vi "ControlProgram6.6_5.vi"() -> ()   [LabVIEW 2016]
uses:
  <vilib>/Utility/miscctls.llb/LVPoint32TypeDef.ctl
  <vilib>/Platform/TimedLoop/XDataNode/timing_clust.ctl
  <vilib>/Platform/TimedLoop/XDataNode/nitl_modes.ctl
  <vilib>/Platform/TimedLoop/XDataNode/wakeup.ctl
  <vilib>/Instr/_visa.llb/Select Event Type.ctl
  <vilib>/vision/Avi1.llb/AviRefnum.ctl
  <vilib>/Utility/error.llb/DialogType.ctl
  <vilib>/DAQmx/write.llb/DAQmx Write (Analog 1D DBL NChan 1Samp).vi
  <vilib>/DAQmx/read.llb/DAQmx Read (Analog 2D DBL NChan NSamp).vi
  <vilib>/Analysis/baseanly.llb/Mean (DBL).vi
  <vilib>/DAQmx/write.llb/DAQmx Write (Digital Bool 1Line 1Point).vi
  <vilib>/DAQmx/create/channels.llb/DAQmx Create Channel (DO-Digital Output).vi
  <vilib>/DAQmx/create/channels.llb/DAQmx Create Channel (AI-Voltage-Basic).vi
  <vilib>/DAQmx/create/channels.llb/DAQmx Create Channel (AO-Voltage-Basic).vi
  <vilib>/DAQmx/configure/timing.llb/DAQmx Timing (Sample Clock).vi
  <vilib>/DAQmx/miscellaneous.llb/DAQmx Fill In Error Info.vi
  <vilib>/Instr/_visa.llb/VISA Configure Serial Port (Instr).vi
  Arnulf--joystick/git(most_up_to_date)/Logitech-joystick/Old Trap/FAST_Global_var.vi
  <vilib>/Utility/inputDevices.llb/mouseAcquire.vi
  <vilib>/Utility/inputDevices.llb/closeMouse.vi
  <vilib>/platform/TimedLoop/XDataNode/XDataNode.xnode
  <vilib>/Platform/TimedLoop/XDataNode/XDNodeRunTimeDep.lvlib
  <resource>/objmgr/daqmx.rc
  <vilib>/Analysis/NI_AALBase.lvlib
panel:
  in  "Save file index":i32
  out "Saving Move":bool
  out "Move time":string
  out "Primary Video Display":T1(plugin-control)
  out "Flush Sample Start Time":u32=2111292881
  out "Sample flush time (s)":dbl=48.0
  in  "Inject Sample":bool
  out "Cal values":T2={"AX alpha"=612.9626061060078, "BX alpha"=549.6584469744151, "AX kappa"=0.3485731373010688, "BX kappa"=0.3853424216291352, "AX offset"=-0.03900484438240665, "BX offset"=-0.11295550662085417, "AY alpha"=582.7562541114835, "BY alpha"=571.1587543790358, "AY kappa"=0.37498408087930674, "BY kappa"=0.36252029651198364, "AY offset"=-0.21125584642206058, "BY offset"=-0.12469077200400738}
  in  "Inject Pump 1":bool
  in  "Inject Pump 2":bool
  in  "Tab Control 2":T3(tab)
  in  "Force FB script":bool
  in  "Got ADig bead":bool
  in  "Move Cap. 2 (ADig Top)":bool
  in  "Dump beads":bool
  in  "Got DNA bead":bool
  in  "Flow on\ncap 2?":bool=TRUE
  in  "Flow on\ncap 1?":bool=TRUE
  in  "Flow on\ndump?":bool=TRUE
  in  "Raster set":i32=1
  in  "Fish After TA?":bool=TRUE
  in  "Delta after tether":dbl=1700.0
  in  "TA Cancel Save?":bool=TRUE
  in  "Min fish\ndelta (nm)":dbl=1425.0 min=0.0 max=5000.0 step=50.0
  in  "Max fish\ndelta (nm)":dbl=1900.0 min=0.0 max=5000.0 step=25.0
  in  "Fish Speed (ms)":i32=5000
  in  "Wait (ms)":i32=1500
  in  "# attempts":dbl=10.0
  in  "Cutoff force (pN)":dbl=4.5
  in  "Raster after\n tether?":bool=TRUE
  out "Tether":bool
  out "Attempt #":i32
  in  "Flow on\nwhile fish?":bool=TRUE
  in  "Flow on\nafter raster?":bool=TRUE
  in  "Offset raster set":i32
  in  "Offset @ Delta (nm)":dbl=1700.0
  in  "Cal @ Delta (nm)":dbl=2500.0
  in  "Cal stage position":i32=3
  out "Cal Final Sampling Rate":dbl=125000.0
  in  "Cal Averaging":i32=1
  in  "Wait before dip (s)":dbl=3.0
  in  "Start dipping after?":bool
  in  "Start trap delta (nm)":dbl=1700.0
  in  "Repeat Dip":bool
  out "Dip #":i32
  in  "Dip attempts":dbl=3.0
  in  "Cancel Rep\n Dip":bool
  out "Return elasped time":i32
  in  "Return duration":dbl=15.0
  in  "Cancel dwell":bool=TRUE
  in  "Pause dwell":bool
  in  "Start/Return position":dbl=3.0
  in  "Dip duration":dbl=15.0
  in  "Dip position":dbl=4.0
  in  "Dip":bool
  out "Dip elasped time":i32
  in  "Stop":bool=TRUE
  in  "?":T4(tab)
  out "FAST X-Y":bool
  out "FAST Z":bool
  in  "Cal time (s)":dbl=5.0
  in  "Save N sets":bool
  in  "N sets":i32=200
  out "Cal sets to save":i32=500
  in  "Reset data stream":bool
  out "Buffer Overflow":bool
  out "Stage moving":bool
  in  "Comment":string
  in  "Raster scan":bool
  out "Saving":bool
  in  "Save cal":bool
  in  "Save Data":bool
  in  "Stop saving":bool
  out "Calibrating":bool
  out "Progress":dbl(slide) scale=0.0..100.0
  in  "Read Cal":bool
  in  "Fish":bool
  in  "Averaging Number":i32=1250
  out "Final Sampling Rate":dbl=100.0
  in  "Trap position (V)":cluster{"X":dbl, "Y":dbl}={"X"=3.9042624789680316, "Y"=0.2}
  in  "Trap delta (nm)":dbl=2500.0 min=0.0 max=5000.0 step=50.0
  in  "Fixed X":dbl=1.1
  in  "Fixed Y":dbl=0.15
  in  "Shutter 1 (B)":bool
  in  "Shutter 2 (A)":bool
  in  "Pulling direction":bool
  out "Raster scanning...":bool
  out "Current file name":path=path "D:/data/160111/160111_006.dat"
  in  "AX alpha":dbl=612.9626061060078 format="%#_3p"
  in  "BX alpha":dbl=549.6584469744151 format="%#_3g"
  in  "AX kappa":dbl=0.3485731373010688 format="%#_3g"
  in  "BX kappa":dbl=0.3853424216291352 format="%#_3g"
  in  "AX offset":dbl=-0.03900484438240665 format="%#_3g"
  in  "BX offset":dbl=-0.11295550662085417 format="%#_3g"
  in  "AY alpha":dbl=582.7562541114835 format="%#_3g"
  in  "BY alpha":dbl=571.1587543790358 format="%#_3g"
  in  "AY kappa":dbl=0.37498408087930674 format="%#_3g"
  in  "BY kappa":dbl=0.36252029651198364 format="%#_3g"
  in  "AY offset":dbl=-0.21125584642206058 format="%#_3g"
  in  "BY offset":dbl=-0.12469077200400738 format="%#_3g"
  out "Buffer status":u8(slide) scale=0.0..100.0
  in  "Target":bool
  in  "Set Current\nPos to (0,0,0)":bool
  in  "dump spot":string="Dump beads spot"
  in  "up flow spot":string="Upper flow spot"
  in  "low flow spot":string="Lower flow spot"
  in  "up cap":string="Upper capillary (ADig beads)"
  in  "bottom cap":string="Lower capillary (DNA beads)"
  in  "Move to Position 5":bool
  in  "Set Position 5":bool
  in  "Saved stage positions":dbl[][](array[numeric])=[[1.0, 0.0, 0.0, 0.0], [2.0, -0.13716, -3.21132, 0.01436], [3.0, 0.45, -0.73974, 0.005], [4.0, 0.45, -2.1978, 0.005], [5.0, 0.45, -2.63158, -0.02256]]
  in  "Set Position 2":bool
  in  "Move to Position 2":bool
  in  "Set Position 1":bool
  in  "Move to Position 1":bool
  in  "Set Position 4":bool
  in  "Move to Position 4":bool
  in  "Set Position 3":bool
  in  "Move to Position 3":bool
  out "Stage error":errorcluster
  in  "Clear Volume":bool
  out "Sample Flush Meter":u8(slide) scale=0.0..100.0
  out "Flushing Sample":bool
  in  "Flush Sample":bool
  in  "Normal \nRate (ul/hr)  3":dbl=100.0
  in  "Normal \nVolume (ul) 3":dbl=250.0
  in  "Normal \nVolume (ul) 2":dbl
  in  "Normal \nRate (ul/hr)":dbl
  in  "Normal \nVolume (ul)":dbl
  in  "Flush\nRate (ul/min)":dbl
  in  "Flush\nVolume (ul)":dbl
  in  "Flush \nRate (ul/min)  2":dbl
  in  "Flush Pump 2":bool
  in  "Flush\nVolume (ul)  2":dbl
  in  "Flush Pump 1":bool
  in  "Normal \nRate (ul/hr)  2":dbl
  in  "Write Wait":i32=1000
  in  "Flush \nRate (ul/min)  3":dbl=100.0
  in  "Flush\nVolume (ul)  3":dbl=80.0
  out "error out":errorcluster
  in  "Use Mouse to Move Trap?":bool
  in  "Pause Mouse/Mirror Connection":bool
  out "Reference Voltage":cluster{dbl, dbl}={0.0, -0.0}
  out "Saved voltage":cluster{dbl, dbl}={5.766666666666665, 1.45}
  out "Real Coordinates":cluster{"Horizontal":i32, "Vertical":i32}={"Horizontal"=897, "Vertical"=-1271}
  out "CoordinatesMousePressed":T5
  in  "Force Feedback 2":bool
  in  "Offset 2":cluster{"Off Y":dbl, "Off X":dbl}={"Off Y"=1.5, "Off X"=0.17}
  in  "Setpoint voltage 2":cluster{"SP Y":dbl, "SP X":dbl}={"SP Y"=0.6, "SP X"=0.0}
  out "Sum error":dbl(knob) scale=-0.2..0.2
  out "Trap sep":waveform(dbl)[](graph)=[{"t0"=timestamp(4.489999999999949 s since 1904-01-01), "dt"=0.002, "Y"=[-1157.7639781743756, -1157.678951177374, -1157.7582331070425, -1157.7490409992681, -1157.8995617642552], "attributes"=variant("NI_ChannelName"=variant(string "T2 X"))}, {"t0"=timestamp(4.489999999999949 s since 1904-01-01), "dt"=0.002, "Y"=[-909.0775466981794, -909.1316439023619, -909.1322956759037, -909.1570630705896, -909.1264297140281], "attributes"=variant("NI_ChannelName"=variant(string "T2 Y"))}]
  in  "Set reading to\nsetpoint 1":bool
  in  "Offset Y (nm)":dbl format="%0.2f"
  in  "Offset X (nm)":dbl format="%0.2f"
  in  "Remove offsets":bool
  in  "Force Feedback 1":bool
  out "Feedback Output \nVoltage 2":cluster{dbl, dbl} {"?" format="%#_4g"; "?" format="%#_4g"}
  in  "Offset 1":cluster{"Off Y":dbl, "Off X":dbl}={"Off Y"=1.5, "Off X"=0.17}
  in  "Setpoint voltage 1":cluster{"SP Y":dbl, "SP X":dbl}={"SP Y"=0.6, "SP X"=0.0}
  in  "Feedback const":T6={"Ki_B_Y"=0.5, "Ki_B_X"=0.0, "Kp Y"=1.0, "Kp X"=0.0}
  out "Mean Trap Pos X 2 (nm)":dbl=-1157.769953044463 format="%0.2f"
  out "Mean Trp Pos Y 2 (nm)":dbl=-909.1249958122125 format="%0.2f"
  out "T2 X RMS (A)":dbl=0.7168002469275427 format="%0.2f"
  out "T2 Y RMS (A)":dbl=0.25997187037503383 format="%0.2f"
  in  "Set reading to\nsetpoint 2":bool
  in  "Scan range (nm)":dbl=425.0
  in  "Scan speed (nm/s)":dbl=100.0 min=0.0 max=100.0
  in  "Step size (nm)":dbl=1.0
  in  "Save scans":bool=TRUE
  in  "# scans":i32=1
  in  "Load param":bool
  in  "Scan Parameters":T7(array[cluster])
  in  "Trap delta\nafter (nm)":dbl=1550.0
  in  "Stop raster":bool
  out "Scan range (V)":dbl=0.47672462142456534
  out "Scan steps (mirror)":u64=425
  out "Scan increment (V)":dbl=0.0011217049915872126
  out "Time per step (ms)":dbl=10.0
  out "Total raster time (s)":dbl=8.5
  out "N sets to be saved":dbl=850.0
  in  "Zoom Factor":sgl=7.0
  in  "Center Point":cluster{"X":i32, "Y":i32}={"X"=335, "Y"=271}
  in  "Intensity Upper":dbl=88.0
  in  "Intensity Lower":dbl=66.0
  out "Window Size":cluster{"Height":i32, "Width":i32}
  in  "Image Index":dbl=1.0 min=1.0
  in  "Save Image":bool
  in  "Averaging":bool
  in  "Reset Averaging":bool
  in  "Save Video":bool
  in  "New Video File":bool
  in  "Video Index":dbl=1.0 min=1.0 step=1.0
  in  "Video Capture Rate (Hz)":dbl=30.0
  in  "Initial Window Size":cluster{"Width":i32, "Height":i32}={"Width"=884, "Height"=619}
  in  "Initial Window Position":cluster{"X Position":i32, "Y Position":i32}={"X Position"=796, "Y Position"=4}
  out "Window Position":cluster{"X Position":i32, "Y Position":i32}={"X Position"=40, "Y Position"=40}
  out "Path Out":path
  in  "Target coordinates":cluster{"X1":dbl, "Y1":dbl, "X2":dbl, "Y2":dbl}={"X1"=328.0, "Y1"=274.0, "X2"=368.0, "Y2"=314.0}
  in  "# Samples/channel (in)":i32=40000 format="%.2f"
  out "Buffer size\n(Samples/channel)":u32=511
  out "DAQ rate\n(Samples/s)":dbl=125000.0 format="%#_6p"
  out "# Samples/channel":i32=1250
  out "# Samples/channel/s":dbl=100.0
  out "AvailSampPerChan":u32=9
  out "Data update period (s/set)":dbl=0.01 format="%#_6p"
  out "AvailSampPerChan 2":u32=110
  in  "PC samp per channel":i32=1000
  in  "Sampling Rate":dbl=125000.0 format="%0.0p"
  in  "DAQ Rate2":dbl=1000000.0 format="%#_6p"
  out "Data period (s)":dbl=8e-06 format="%#_6p"
  in  "Save user params":bool
  in  "User":string(combo)
  in  "Load user params":bool
  in  "Tether break\nforce (pN)":dbl=1.0
  in  "Path":path=path "E:/Data"
  out "Mirror task":refnum<k21>
  in  "Conv X (nm/V)":dbl=891.5
  in  "Conv Y (nm/V)":dbl=505.7
  in  "Min value Y":dbl format="%.1g"
  in  "Max value Y":dbl=10.0 format="%.1f"
  in  "Min value X":dbl format="%0.1f"
  in  "Max value X":dbl=10.0 format="%.1f"
  in  "HWP1":string="Half waveplate 1: differential trap power"
  in  "HWP0":string="Half waveplate 0: total trap power"
  in  "Move 1":bool
  in  "\"Degrees\" 1":dbl
  in  "Move 0":bool
  in  "\"Degrees\" 0":dbl
  in  "Y command":enum16{"Fish", "Dump", "Got ADig", "Got DNA"}(ring)
  in  "B command":enum16{"Got DNA", "Got ADig", "Dump", "Fish"}(ring)
  in  "A command":enum16{"Got ADig", "Dump", "Fish", "Got DNA"}(ring)
  in  "X command":enum16{"Dump", "Fish", "Got ADig", "Got DNA"}(ring)
  out "Logitech":bool
  out "START":bool
  out "BACK":bool
  out "Right stick button":bool
  out "Left Y":i8(slide) scale=-128.0..127.0
  out "Left X":i8(slide) scale=-128.0..127.0
  out "Right Y":i8(slide) scale=-128.0..127.0
  out "Right X":i8(slide) scale=-128.0..127.0
  out "X":bool
  out "Y":bool
  out "A":bool
  out "B":bool
  out "RB":bool
  out "LB":bool
  out "R":bool
  out "L":bool
  out "D":bool
  out "U":bool
  out "Left stick button":bool
  out "FAST Z":bool
  out "FAST X-Y":bool
  in  "XY Speed Definitions":T8={"Slow X velocity input"="0.05", "Slow Y velocity input"="0.05", "Fast1 X velocity input"="0.1", "Fast1 Y velocity input"="0.1", "Fast2 X velocity input"="0.2", "Fast2 Y velocity input"="0.2"}
  in  "Z Speed Definitions":cluster{"Slow Z":string, "Fast Z":string}={"Slow Z"="0.025", "Fast Z"="0.05"}
  in  "Z Wait time":string="120"
  in  "X-Y Wait time":string="125"
  in  "USB port":refnum<visa-resource-name>="USB0::0x046D::0xC21D::CC66247B::RAW"
  out "Deflection":T5
  in  "Sampling Rate":dbl=125000.0 format="%0.2f"
  in  "Averaging Number":i32=12500
  in  "DAQ Rate":dbl=1000000.0
  out "Final Sampling Rate":dbl
  in  "Tab Control":T9(tab)
  in  "Downsamp\nfact":dbl=250.0
  out "Bead sep":waveform(dbl)[](graph)=[{"t0"=timestamp(4.489999999999949 s since 1904-01-01), "dt"=0.002, "Y"=[8093.963535945606, 8103.1617772716045, 8385.72390184118, 8245.733099167523, 8154.925676756515], "attributes"=variant("NI_ChannelName"=variant(string "T2"))}, {"t0"=timestamp(4.489999999999949 s since 1904-01-01), "dt"=0.002, "Y"=[1717.924930434114, 1628.723007842151, 1787.6888378897193, 1598.475730715916, 1776.2517588078954], "attributes"=variant("NI_ChannelName"=variant(string "T1"))}]
  out "Force (pN)":waveform(dbl)[](graph)=[{"t0"=timestamp(4.489999999999949 s since 1904-01-01), "dt"=0.002, "Y"=[2821.5994183803123, 2824.8226375853515, 2923.3663028678166, 2874.5254578927593, 2842.869034836209], "attributes"=variant("NI_ChannelName"=variant(string "T2"))}, {"t0"=timestamp(4.489999999999949 s since 1904-01-01), "dt"=0.002, "Y"=[623.5850847499229, 591.0680427774053, 648.761979867749, 579.944408346982, 644.7436619059413], "attributes"=variant("NI_ChannelName"=variant(string "T1"))}]
  out "Mean force (pN)":dbl=1737.5286029210451 format="%0.2f"
  out "Force noise (pN)":dbl=26.83032703631318 format="%0.2f"
  out "Mean Bead Sep\n(nm)":dbl=4949.257225667222 format="%0.2f"
  out "Bead Sep Noise\n(A)":dbl=757.8078481959694 format="%0.2f"
  out "PSD 2":cluster{dbl[], dbl[]}(graph)
  out "PSD 1":cluster{dbl[], dbl[]}(graph)
  out "PSD 1 Sum":dbl(slide) scale=0.0..10.0
  out "PSD 2 Sum":dbl(slide) scale=0.0..10.0
  in  "Start":bool
  out "All signals 2":waveform(dbl)[](graph)=[{"t0"=timestamp(4.489999999999949 s since 1904-01-01), "dt"=0.002, "Y"=[0.0010396217068286443, 0.0010666908927528754, 0.001103298744846499, 0.0010651440823993424, 0.0010656596859401936], "attributes"=variant("NI_ChannelName"=variant(string "A y"))}, {"t0"=timestamp(4.489999999999949 s since 1904-01-01), "dt"=0.002, "Y"=[0.02000680227246931, 0.020097032918054827, 0.02003412926844257, 0.020136734401221615, 0.020087494249822452], "attributes"=variant("NI_ChannelName"=variant(string "A x"))}, {"t0"=timestamp(4.489999999999949 s since 1904-01-01), "dt"=0.002, "Y"=[-0.0014958587831537804, -0.0015046240440107857, -0.0014930229638311983, -0.001533240041751485, -0.0015262793936602433], "attributes"=variant("NI_ChannelName"=variant(string "B y"))}, {"t0"=timestamp(4.489999999999949 s since 1904-01-01), "dt"=0.002, "Y"=[0.0002901198559372817, 0.0002731049385577592, 0.00026511308349727467, 0.0002517073909711183, 0.0002916666665966012], "attributes"=variant("NI_ChannelName"=variant(string "B x"))}, {"t0"=timestamp(4.489999999999949 s since 1904-01-01), "dt"=0.002, "Y"=[-0.001511556786147372, -0.0015167122027053212, -0.0014612914746018214, -0.0014935128282145193, -0.0015064013696263116], "attributes"=variant("NI_ChannelName"=variant(string "A sum"))}, {"t0"=timestamp(4.489999999999949 s since 1904-01-01), "dt"=0.002, "Y"=[-0.0005242945138364382, -0.0005565158674093218, -0.000501095139248956, -0.0005771375336978897, -0.0005165613890095197], "attributes"=variant("NI_ChannelName"=variant(string "B sum"))}, {"t0"=timestamp(4.489999999999949 s since 1904-01-01), "dt"=0.002, "Y"=[0.0013303666019343777, 0.0014257418088905328, 0.0013368108726387405, 0.0013471217058124534, 0.0011782818123890176], "attributes"=variant("NI_ChannelName"=variant(string "Trap x"))}, {"t0"=timestamp(4.489999999999949 s since 1904-01-01), "dt"=0.002, "Y"=[0.0023382505474007294, 0.002231275652833831, 0.002229986798687363, 0.0021810103409340116, 0.002241586486003531], "attributes"=variant("NI_ChannelName"=variant(string "Trap y"))}]
  out "All signals":waveform(dbl)[](graph)=[{"t0"=timestamp(4.489999999999949 s since 1904-01-01), "dt"=0.002, "Y"=[0.0010396217068286443, 0.0010666908927528754, 0.001103298744846499, 0.0010651440823993424, 0.0010656596859401936], "attributes"=variant("NI_ChannelName"=variant(string "A y"))}, {"t0"=timestamp(4.489999999999949 s since 1904-01-01), "dt"=0.002, "Y"=[0.02000680227246931, 0.020097032918054827, 0.02003412926844257, 0.020136734401221615, 0.020087494249822452], "attributes"=variant("NI_ChannelName"=variant(string "A x"))}, {"t0"=timestamp(4.489999999999949 s since 1904-01-01), "dt"=0.002, "Y"=[-0.0014958587831537804, -0.0015046240440107857, -0.0014930229638311983, -0.001533240041751485, -0.0015262793936602433], "attributes"=variant("NI_ChannelName"=variant(string "B y"))}, {"t0"=timestamp(4.489999999999949 s since 1904-01-01), "dt"=0.002, "Y"=[0.0002901198559372817, 0.0002731049385577592, 0.00026511308349727467, 0.0002517073909711183, 0.0002916666665966012], "attributes"=variant("NI_ChannelName"=variant(string "B x"))}, {"t0"=timestamp(4.489999999999949 s since 1904-01-01), "dt"=0.002, "Y"=[-0.001511556786147372, -0.0015167122027053212, -0.0014612914746018214, -0.0014935128282145193, -0.0015064013696263116], "attributes"=variant("NI_ChannelName"=variant(string "A sum"))}, {"t0"=timestamp(4.489999999999949 s since 1904-01-01), "dt"=0.002, "Y"=[-0.0005242945138364382, -0.0005565158674093218, -0.000501095139248956, -0.0005771375336978897, -0.0005165613890095197], "attributes"=variant("NI_ChannelName"=variant(string "B sum"))}, {"t0"=timestamp(4.489999999999949 s since 1904-01-01), "dt"=0.002, "Y"=[0.0013303666019343777, 0.0014257418088905328, 0.0013368108726387405, 0.0013471217058124534, 0.0011782818123890176], "attributes"=variant("NI_ChannelName"=variant(string "Trap x"))}, {"t0"=timestamp(4.489999999999949 s since 1904-01-01), "dt"=0.002, "Y"=[0.0023382505474007294, 0.002231275652833831, 0.002229986798687363, 0.0021810103409340116, 0.002241586486003531], "attributes"=variant("NI_ChannelName"=variant(string "Trap y"))}]
  out "Chart Freq (Hz)":dbl=500.0
  # "Bead Calibration"
  # "Y"
  # "X"
  # "Pump #1 Controls"
  # "Pump #2 Controls"
  # "Sample Pump Controls"
  # "Retract the pumps manually. Change it back to INFUSE when you're done. Suck it up, don't whine."
  # "Shutter 1 (B)"
  # "Move to Lower Cap"
  # "Inject Sample"
  # "Move to Upper Cap"
  # "Shutter 2 (A)"
  # "Select the Joystick input:"
  # "Overflow happens when >40 commands\nsent in 5 seconds. Then 4 consecutive beeps."
  # "Try increasing wait time to reduce 'following error threshold exceeded' occurances."
  # "Left stick controls Z axis.\nRight on stick: neg Z-dir\nUp on stick: neg Z-dir"
  # "Toggles FAST Z"
  # "Toggles FAST X-Y"
  # "The default Newport max velocity is 0.4"
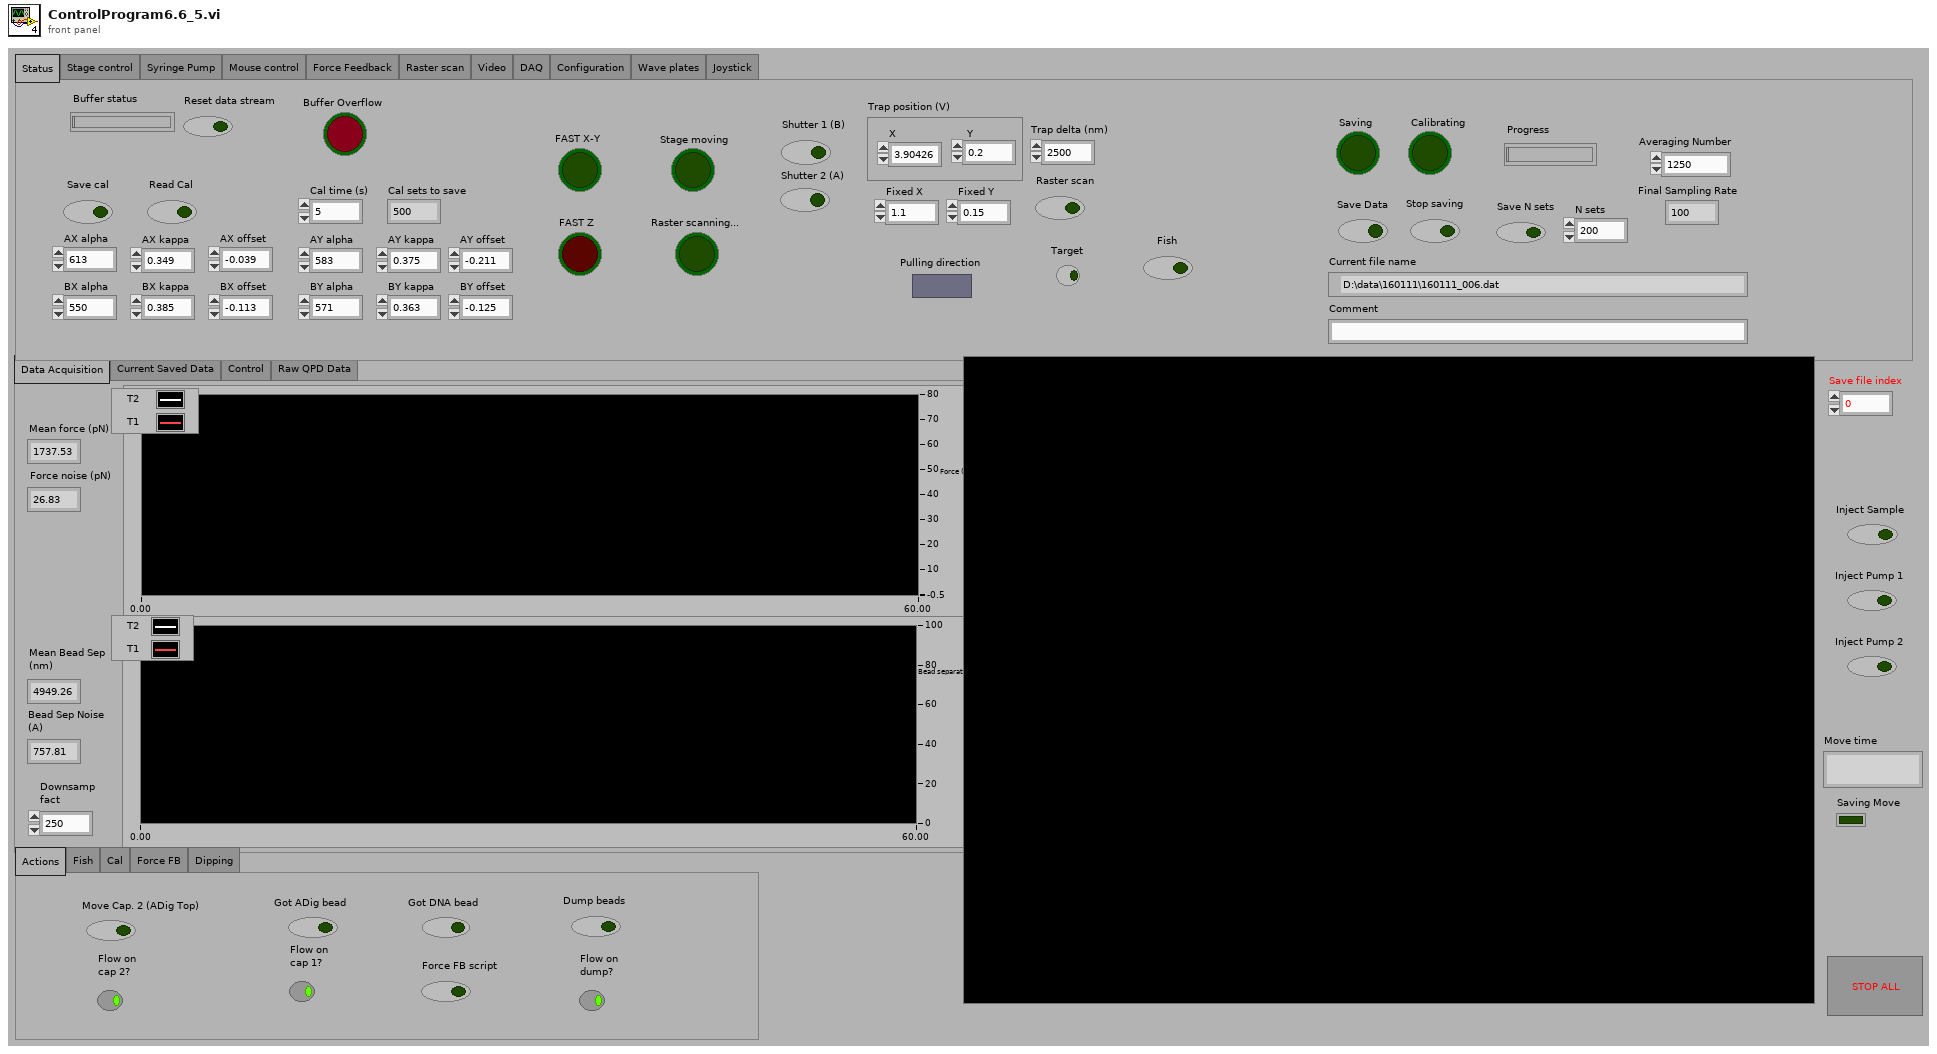
[diagram p1: front panel]
types:
  T1 = typedef "IMAQ Image.ctl" = refnum<image>
  T2 = cluster{"AX alpha":dbl, "BX alpha":dbl, "AX kappa":dbl, "BX kappa":dbl, "AX offset":dbl, "BX offset":dbl, "AY alpha":dbl, "BY alpha":dbl, "AY kappa":dbl, "BY kappa":dbl, "AY offset":dbl, "BY offset":dbl}
  T3 = enum32{"Actions", "Fish", "Cal", "Force FB", "Dipping"}
  T4 = enum32{"Status", "Stage control", "Syringe Pump", "Mouse control", "Force Feedback", "Raster scan", "Video", "DAQ", "Configuration", "Wave plates", "Joystick"}
  T5 = typedef "LVPoint32TypeDef.ctl" = cluster{"Horizontal":i32, "Vertical":i32}
  T6 = cluster{"Ki_B_Y":dbl, "Ki_B_X":dbl, "Kp Y":dbl, "Kp X":dbl}
  T7 = cluster{"Label":string, "Scan range 1":dbl, "Step size 1":dbl, "Scan speed 1":i32, "# scans 2":i32}[]
  T8 = cluster{"Slow X velocity input":string, "Slow Y velocity input":string, "Fast1 X velocity input":string, "Fast1 Y velocity input":string, "Fast2 X velocity input":string, "Fast2 Y velocity input":string}
  T9 = enum32{"Data Acquisition", "Current Saved Data", "Control", "Raw QPD Data"}
  T10 = typedef "Select Event Type.ctl" = u32
  T11 = enum32{"setting", "request", "request control", "info", "statistics", "system settings", "I/O sub system", "HRT control", "camera descriptions", "device specific data", "event sub system settings", "event sub system results", "image memory manager"}
  T12 = typedef "AviRefnum.ctl" = refnum<k1>
  T13 = typedef "XDNodeRunTimeDep.lvlib/timing_clust.ctl" = cluster{"Expected End [f-1]":u64, "Actual End [f-1]":u64, "Finished Late? [f-1]":bool, "Expected End [i-1]":u64, "Actual End [i-1]":u64, "Finished Late? [i-1]":bool, "Expected Start [i]":u64, "Actual Start [i]":u64, "Expected Start [f]":u64, "Actual Start [f]":u64, "Source Name":string, "Structure Name":string, "Period":i64, "Deadline":i64, "Offset":i64, "Start":i64, "Priority":i32, "Timeout":i32, "Mode":T14, "Wakeup Reason":T15, "Error":errorcluster, "Source Type":string, "Secondary Source Type":string, "Global End Time":u64, "Global Start Time":u64, "Frame Duration":u64, "Iteration Duration":u64, "Assigned CPU":i32, "I/O Scan Engine Mode":u32}
  T14 = typedef "XDNodeRunTimeDep.lvlib/nitl_modes.ctl" = enum32{"No Change", "Process missed periods, maintain original phase", "Discard missed periods, maintain original phase", "Process missed periods, ignore original phase", "Discard missed periods, ignore original phase"}
  T15 = typedef "XDNodeRunTimeDep.lvlib/wakeup.ctl" = enum32{"Normal", "Aborted", "Asynchronous wakeup", "Timing source error", "Timed loop error", "Timeout"}
  T16 = typedef "Image Type" = u32
  T17 = typedef "imagedata.ctl" = cluster{"image type":i32, "image depth":i32, "image":u8[], "mask":u8[], "colors":u32[], "Rectangle":cluster{"left":i16, "top":i16, "right":i16, "bottom":i16}}
  T18 = enum16{"open", "replace", "create", "open or create", "replace or create", "replace or create with confirmation"}
  T19 = enum16{"big-endian, network order", "native, host order", "little-endian"}
  T20 = cluster{string, string, string, string, string, string, string, string}
  T21 = cluster{"LB":bool, "RB":bool, "BACK":bool, "Logitech":bool, "START":bool}
  T22 = cluster{"Right X":i8, "Right Y":i8, "Left X":i8, "Left Y":i8}
  T23 = enum32{"Status", "Stage control", "Syringe Pump", "Mouse control", "Force Feedback", "Raster scan", "Video", "DAQ", "Configuration", "Wave plates"}
  T24 = typedef "DialogType.ctl" = u16
  T25 = cluster{"button 1":bool, "button 2":bool, "button 3":bool, "button 4":bool}
  T26 = cluster{"[0]":dbl, "[1]":dbl, "[2]":dbl, "[3]":dbl, "[4]":dbl, "[5]":dbl, "[6]":dbl, "[7]":dbl, "[8]":dbl, "[9]":dbl, "[10]":dbl, "[11]":dbl}
  T27 = cluster{"Label":string, "Scan range 1":dbl, "Step size 1":dbl, "Scan speed 1":i32, "# scans 2":i32}
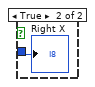
[diagram p5: hidden frame]
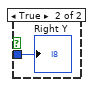
[diagram p6: hidden frame]
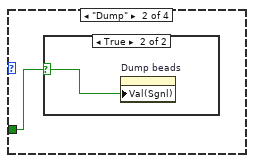
[diagram p10: hidden frame]
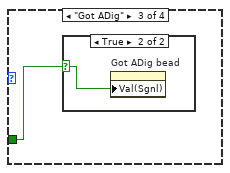
[diagram p12: hidden frame]
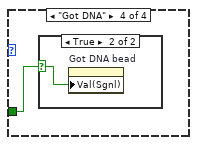
[diagram p14: hidden frame]
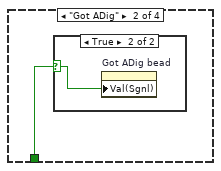
[diagram p17: hidden frame]
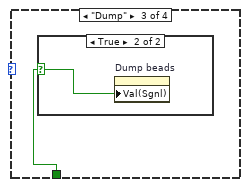
[diagram p19: hidden frame]
diagram:
  w10 = T10 1073684535 items=["Service Request"=1073684491, "Trigger"=3221168138, "Clear"=1073684493, "VXI Signal"=1073684512, "VXI/VME Interrupt"=3221168161, "VXI/VME Sysfail"=1073684509, "VXI/VME Sysreset"=1073684510, "GPIB CIC"=1073684498, "GPIB Talk"=1073684499, "GPIB Listen"=1073684500, "PXI Interrupt"=1073684514, "Serial Break"=1073684515, "Serial TermChar"=1073684516, "Serial CTS"=1073684521, "Serial DSR"=1073684522, "Serial DCD"=1073684524, "Serial RI"=1073684526, "Serial Character"=1073684533, "USB Interrupt"=1073684535, "All Enabled"=1073709055] ("Event Type")
  w49 = 10.0 ("Minimum Value")
  w50 = -10.0 ("Minimum Value")
  w52 = -2.0 ("Minimum Value")
  w53 = 2.0 ("Maximum Value")
  w78 = 10123 items=["Finite Samples"=10178, "Continuous Samples"=10123] ("sample mode")
  w98 = tag "Dev1/port2/line1"  # Shutter 2
  w101 = tag "Dev1/port1/line4"  # Shutter 1
  # "Open the RAW resource"
  # "Enable USB Interrupt Event"
  # "Create channels for movable mirror"
  # "Create channels for detectors"
  n1 = call-poly <vilib>:"DAQmx Create Virtual Channel.vi"("maximum value"=w53, "minimum value"=w52, "physical channels"=tag "Dev1/ai0" ("Physical Channel")) -> ("task out"=w54:refnum<k21>, "error out"=w77:errorcluster)  [unwired: 11 in]
  n2 = call-poly <vilib>:"DAQmx Create Virtual Channel.vi"("task in"=w54, "maximum value"=w53, "minimum value"=w52, "physical channels"=tag "Dev1/ai1", "error in"=w77) -> ("task out"=w75:refnum<k21>, "error out"=w74:errorcluster)  [unwired: 9 in]
  n3 = call-poly <vilib>:"DAQmx Create Virtual Channel.vi"("task in"=w75, "maximum value"=w53, "minimum value"=w52, "physical channels"=tag "Dev1/ai2", "error in"=w74) -> ("task out"=w66:refnum<k21>, "error out"=w65:errorcluster)  [unwired: 9 in]
  n4 = call-poly <vilib>:"DAQmx Create Virtual Channel.vi"("task in"=w66, "maximum value"=w53, "minimum value"=w52, "physical channels"=tag "Dev1/ai3" ("Physical Channel"), "error in"=w65) -> ("task out"=w51:refnum<k21>, "error out"=w71:errorcluster)  [unwired: 9 in]
  n5 = call-poly <vilib>:"DAQmx Create Virtual Channel.vi"("task in"=w51, "maximum value"=w49, "minimum value"=w50, "physical channels"=tag "Dev1/ai4", "error in"=w71) -> ("task out"=w69:refnum<k21>, "error out"=w68:errorcluster)  [unwired: 9 in]
  n6 = call-poly <vilib>:"DAQmx Create Virtual Channel.vi"("task in"=w69, "maximum value"=w49, "minimum value"=w50, "physical channels"=tag "Dev1/ai5", "error in"=w68) -> ("task out"=w64:refnum<k21>, "error out"=w63:errorcluster)  [unwired: 9 in]
  n7 = call-poly <vilib>:"DAQmx Create Virtual Channel.vi"("task in"=w64, "maximum value"=w49, "minimum value"=w50, "physical channels"=tag "Dev1/ai6", "error in"=w63) -> ("task out"=w58:refnum<k21>, "error out"=w56:errorcluster)  [unwired: 9 in]
  n8 = call-poly <vilib>:"DAQmx Create Virtual Channel.vi"("task in"=w58, "maximum value"=w49, "minimum value"=w50, "physical channels"=tag "Dev1/ai7", "error in"=w56) -> ("task out"=w57:refnum<k21>, "error out"=w55:errorcluster)  [unwired: 9 in]
  n9 = call-poly <vilib>:"DAQmx Timing.vi"("task/channels in"=w57, "sample mode"=w78, "samples per channel"="PC samp per channel", "rate"="Sampling Rate", "error in"=w55) -> ("task out"=w61:refnum<k21>, "error out"=w60:errorcluster)  [unwired: 9 in]
  n10 = call-poly <vilib>:"DAQmx Create Virtual Channel.vi"("maximum value"="Max value Y", "minimum value"="Min value Y", "physical channels"=tag "Dev1/ao1" ("Trap X Axis")) -> ("task out"=w46:refnum<k21>, "error out"=w48:errorcluster)  [unwired: 11 in]
  n11 = property class="DAQmx Timing"(reference=w61, error in=w60, "More:AI Convert:Rate"="DAQ Rate2") -> (reference out=w19:refnum<k21>, error out=w18:errorcluster, "SampClk.Rate"=→"DAQ rate\n(Samples/s)":dbl)
  n12 = call-poly <vilib>:"DAQmx Create Virtual Channel.vi"("task in"=w46, "maximum value"="Max value X", "minimum value"="Min value X", "physical channels"=tag "Dev1/ao0" ("Trap Y Axis"), "error in"=w48) -> ("task out"=w37:refnum<k21>, "error out"=w36:errorcluster)  [unwired: 9 in]
  "Mirror task" <- w37
  n13 = property class="DAQmx Buffer"(reference=w19, error in=w18) -> (reference out=w16:refnum<k21>, error out=w15:errorcluster, "Input.OnbrdBufSize"=→"Buffer size\n(Samples/channel)":u32)
  n14 = call <vilib>:"DAQmx Start Task.vi"("task/channels in"=w16, "error in"=w15) -> ("task out"=w38:refnum<k21>)  [unwired: 12 in, 1 out]
  n15 = flat-sequence "Video" {
    tunnel: [w114] -> w13
    tunnel: w13 -> [w155]
    frame #0 {
      n16 = while {
        stop <- w107 continue-if-true
        n17 = call "Close Video Capture.vi"() -> ("error code OUT"=w109:i32)
        n18 = Equal?(x=w109, y=0) -> (x = y?=w107:bool)
      }
      n19 = local write "Stop"(FALSE ("Stop All")) -> ()
    }
    frame #1 {
      n20 = call "DMR_Init.vi"() -> ()  [unwired: 3 out]
    }
    frame #2 {
      # "Setting the destination format to Mono8 makes sure that the image can be displayed in the intensity plot."
      n21 = call "DMR_GetDevice.vi"("search string IN"="DE514724602") -> ("device handle OUT"=w132:i32)  [unwired: 4 in, 2 out]
      n22 = call "DMR_OpenDevice.vi"("device handle IN"=w132) -> ("driver handle OUT"=w115:i32)  [unwired: 4 out]
      n23 = call "DMR_FindList.vi"("flags IN"=u32 0 ("flags"), "list name IN"="" ("String"), "list type IN"=T11."camera descriptions", "driver handle IN"=w115) -> ("list handle OUT"=w118:i32)  [unwired: 2 out]
      n24 = call "DMR_FindList.vi"("flags IN"=u32 0 ("flags"), "list name IN"="Base", "list type IN"=T11."setting", "driver handle IN"=w115) -> ("list handle OUT"=w116:i32)  [unwired: 2 out]
      n25 = call "OBJ_GetHandle.vi"("object name IN"="VideoStandard", "list handle IN"=w118) -> ("object handle OUT"=w112:i32)  [unwired: 3 out]
      n26 = call "OBJ_GetHandle.vi"("object name IN"="PixelFormat", "list handle IN"=w116) -> ("object handle OUT"=w126:i32)  [unwired: 3 out]
      n27 = call "OBJ_SetS.vi"("value index IN"=0, "value IN"="NTSC M", "object handle IN"=w112) -> ()  [unwired: 2 out]
      n28 = call "OBJ_SetS.vi"("value index IN"=0, "value IN"="Mono8" ("value"), "object handle IN"=w126) -> ()  [unwired: 2 out]
      n29 = call "OBJ_GetHandle.vi"("object name IN"="VideoChannel", "list handle IN"=w116) -> ("object handle OUT"=w122:i32)  [unwired: 3 out]
      n30 = while {
        tunnel: [w137] -> w114
        tunnel: w115 -> [w134]
        stop <- w135 continue-if-true
        n31 = call "DMR_ImageRequestSingle.vi"("request control IN"=0, "driver handle IN"=w134) -> ("error code OUT"=w136:i32, "driver handle OUT"=w137:i32)  [unwired: 2 out]
        n32 = Equal To 0?(x=w136) -> (x = 0?=w135:bool)
      }
      n33 = call "OBJ_SetI.vi"("value index IN"=0, "value IN"=0 ("Video channel"), "object handle IN"=w122) -> ()  [unwired: 2 out]
    }
    frame #3 {
      w143 = T16 0 items=["Grayscale (U8)", "Grayscale (I16)", "Grayscale (SGL)", "Complex (CSG)", "RGB (U32)", "HSL (U32)", "RGB (U64)"] ("Image Type")
      w151 = T16 0 items=["Grayscale (U8)", "Grayscale (I16)", "Grayscale (SGL)", "Complex (CSG)", "RGB (U32)", "HSL (U32)", "RGB (U64)"] ("Image Type")
      n34 = for "Create Greyscale map" {
        N: 256 -> [_]
        tunnel: [w157] -> w140 mode=indexing
        workers-P: _ -> [_]
        i -> [w160]
        n35 = To Unsigned Byte Integer(number=w160) -> (unsigned 8bit integer=w156:u8)
        n36 = Join Numbers(hi=w156, lo=w156) -> ((hi.lo)=w159:u16)
        n37 = Join Numbers(hi=w156, lo=w156) -> ((hi.lo)=w158:u16)
        n38 = Join Numbers(hi=w159, lo=w158) -> ((hi.lo)=w157:u32)
      }
      n39 = call "IMAQ Create"("Image Name"="Scaled video", "Image Type"=w143) -> ("New Image"=w142:T1)  [unwired: 2 in, 2 out]
      n40 = call "IMAQ Create"("Image Name"="Main video", "Image Type"=w151) -> ("New Image"=w152:T1)  [unwired: 2 in, 2 out]
      n41 = node-c288(0 ("Processor")) -> (w150:T13)  [unwired: 3 out]
      n42 = Initialize Array(u32 0 ("Window Number (0...15)"), 480 ("dimension size"), 640 ("dimension size")) -> (w145:u32[][])
      n43 = timed-loop {
        tunnel: w155 -> [w177]
        tunnel: [w176] -> w154
        tunnel: w152 -> [w175]
        timing: w150 -> [_]
        timing-out: [_] -> w149
        tunnel: w145 -> [w164]
        tunnel: w142 -> [w162]
        tunnel: w140 -> [w161]
        stop <- w163 stop-if-true
        # "This block performs the \nactual image capture."
        n44 = node-c288() -> ()  [unwired: 2 out]
        n45 = local read "Stop"() -> (w163:bool)
        n46 = Reciprocal(x="Video Capture Rate (Hz)") -> (1/x=w167:dbl)
        n47 = Multiply(x=w167, y=1000.0) -> (x*y=w165:dbl)
        n48 = call "DMR_ImageRequestWaitFor.vi"("queue number IN"=0, "timeout(ms) IN"=500, "driver handle IN"=w177) -> ("error code OUT"=w181:i32, "request number OUT"=w178:i32, "driver handle OUT"=w179:i32)
        n49 = feedback #1(T12 refnum ("Avi Refnum")) -> (w169:T12)
        n50 = case shown="True" "New Video File" {
          tunnel: [T12 refnum ("Avi Refnum") w198] -> w171
          tunnel: [FALSE TRUE] -> w172
          tunnel: w169 -> [_ w194]
          frame False {
          }
          frame True {
            n51 = call "Create new save file.vi"("Ext"=".avi" ("string"), "Index In"="Video Index") -> ("Path Out"=w190:path, "Index Out"=w191:dbl)  [unwired: 1 in]
            "Path Out" <- w190
            n52 = Not Equal?(x=w194, y=T12 refnum ("Avi Refnum")) -> (x != y?=w195:bool)
            n53 = Increment(x=w191) -> (x+1=w200:dbl)
            n54 = case shown="True" w195 {
              tunnel: w194 -> [_ w201]
              frame False {
              }
              frame True {
                n55 = call "IMAQ AVI Close"("Avi Refnum"=w201) -> ()  [unwired: 1 in, 10 out]
              }
            }
            n56 = local write "Video Index"(w200) -> ()
            n57 = call "IMAQ AVI Create"("Frames Per Second"=u32 30, "AVI Path"=w190) -> ("Avi Refnum"=w198:T12)  [unwired: 5 in, 4 out]
          }
        }
        n58 = Equal To 0?(x=w181) -> (x = 0?=w180:bool)
        n59 = Select(t=w171, s=w172, f=w169) -> (s? t:f=w170:T12)
        n60 = feedback-in #1(w170) -> ()
        n61 = case shown="True" w180 {
          tunnel: w179 -> [w202 w229]
          tunnel: w178 -> [_ w228]
          tunnel: [w202 w225] -> w176
          tunnel: w175 -> [_ w206]
          tunnel: w164 -> [_ w213]
          tunnel: w170 -> [_ w211]
          tunnel: w162 -> [_ w207]
          tunnel: w161 -> [_ w208]
          frame False {
          }
          frame True {
            w219 = u32 0 ("X-offset IN")
            n62 = call "DMR_GetImageRequestBufferData.vi"("driver handle IN"=w229, "request number IN"=w228) -> ("width OUT"=w218:i32, "height OUT"=w217:i32, "driver handle OUT"=w224:i32, "request number OUT"=w223:i32, "bytes per pixel OUT"=w220:i32)  [unwired: 13 out]
            n63 = call "DMR_GetImageRequestBufferImageData.vi"("driver handle IN"=w224, "request number IN"=w223, "bytes per pixel IN"=w220, "X-offset IN"=w219, "Y-offset IN"=w219, "height IN"=w217, "width IN"=w218) -> ("driver handle OUT"=w222:u32, "request number OUT"=w221:u32, "image OUT"=w214:u32[][])  [unwired: 10 out]
            n64 = call "DMR_ImageRequestUnlock.vi"("request number IN"=w221, "driver handle IN"=w222) -> ("driver handle OUT"=w227:i32)  [unwired: 1 in, 2 out]
            n65 = case shown="False" "Averaging" {
              tunnel: w214 -> [w270 w275]
              tunnel: [w270 w274] -> w210
              tunnel: w213 -> [_ w272]
              frame False {
              }
              frame True {
                (unwired) 1
                w280 = 1
                n66 = feedback #2(w272) -> (w271:u32[][])
                n67 = Add(x=w275, y=w271) -> (x+y=w276:u32[][])
                n68 = Select(t=w272, s="Reset Averaging", f=w276) -> (s? t:f=w278:u32[][])
                n69 = feedback-in #2(w278) -> ()
                n70 = feedback #3(w280) -> (w273:i32)
                n71 = Divide(x=w276, y=w273) -> (x/y=w277:dbl[][])
                n72 = Increment(x=w273) -> (x+1=w281:i32)
                n73 = To Unsigned Long Integer(number=w277) -> (unsigned 32bit integer=w274:u32[][])
                n74 = Select(t=w280, s="Reset Averaging", f=w281) -> (s? t:f=w279:i32)
                n75 = feedback-in #3(w279) -> ()
              }
            }
            n76 = call "DMR_ImageRequestSingle.vi"("request control IN"=0, "driver handle IN"=w227) -> ("driver handle OUT"=w225:i32)  [unwired: 3 out]
            n77 = disable-structure shown="Disabled" {
              disable-tunnel: w210 -> [w247 _]
              disable-tunnel: w207 -> [w246 _]
              frame Disabled {
                n78 = To Double Precision Float(number=w247) -> (double precision float=w245:dbl[][])
                n79 = In Range and Coerce(upper limit="Intensity Upper", x=w245, lower limit="Intensity Lower") -> (coerced(x)=w244:dbl[][])  [unwired: 1 out]
                n80 = Subtract(x="Intensity Upper", y="Intensity Lower") -> (x-y=w241:dbl)
                n81 = Subtract(x=w244, y="Intensity Lower") -> (x-y=w242:dbl[][])
                n82 = Divide(x=w242, y=w241) -> (x/y=w243:dbl[][])
                n83 = Multiply(x=255.0, y=w243) -> (x*y=w239:dbl[][])
                n84 = To Unsigned Byte Integer(number=w239) -> (unsigned 8bit integer=w248:u8[][])
                n85 = call "IMAQ ArrayToImage"("Image Pixels (U8)"=w248, "Image"=w246) -> ("Image Out"=w235:T1)  [unwired: 4 in, 5 out]
                n86 = First Call?() -> (First Call?: T/F=w236:bool)
                n87 = case shown="True" w236 {
                  tunnel: w235 -> [w249 w260]
                  frame False {
                    n88 = flat-sequence {
                      tunnel: w249 -> [w255]
                      frame #0 {
                        w252 = FALSE ("Get/Set Status? (Set)")
                        w251 = 0 ("Window Number (0...15)")
                        n89 = call "IMAQ WindSize"("Get/Set Status? (Set)"=w252, "Window Number"=w251) -> ("Width & Height out"=→"Window Size":cluster{"Width":i32, "Height":i32})  [unwired: 4 in, 2 out]
                        n90 = call "IMAQ WindMove"("Window Number (0...15)"=w251, "Get/Set Status? (Set)"=w252) -> ("Coordinates (screen)"=→"Window Position":cluster{"X Position":i32, "Y Position":i32})  [unwired: 3 in, 1 out]
                        n91 = call "IMAQ WindDraw"("Resize to Image Size? (Y)"=FALSE, "Window Number (0...15)"=w251, "Image"=w255) -> ()  [unwired: 7 in, 2 out]
                      }
                      frame #1 {
                        n92 = call "IMAQ WindZoom 2"("Center Point"="Center Point", "Zoom to Fit? (False)"=FALSE, "Zoom Factor"="Zoom Factor") -> ()  [unwired: 5 in, 4 out]
                      }
                    }
                  }
                  frame True {
                    n93 = flat-sequence {
                      tunnel: w260 -> [w263]
                      tunnel: [w261] -> w259
                      tunnel: w259 -> [w265]
                      frame #0 {
                        w262 = TRUE ("Resize to Image Size? (Y)")
                        w261 = 0 ("Window Number (0...15)")
                        n94 = call "IMAQ WindNonTearing"("Window Number"=w261, "NonTearing? (True)"=w262) -> ()  [unwired: 8 in, 2 out]
                        n95 = call "IMAQ WindDraw"("Resize to Image Size? (Y)"=w262, "Window Number (0...15)"=w261, "Image"=w263) -> ()  [unwired: 7 in, 2 out]
                      }
                      frame #1 {
                        n96 = call "IMAQ WindSize"("Scrollbars? (N)"=FALSE, "Width & Height"="Initial Window Size", "Window Number"=w265) -> ()  [unwired: 3 in, 3 out]
                        n97 = call "IMAQ WindMove"("Window Number (0...15)"=w265, "Coordinates (screen)"="Initial Window Position") -> ()  [unwired: 3 in, 2 out]
                      }
                    }
                  }
                }
              }
              frame Enabled {
              }
            }
            n98 = To Unsigned Byte Integer(number=w210) -> (unsigned 8bit integer=w209:u8[][])
            n99 = call "IMAQ ArrayToImage"("Image Pixels (U8)"=w209, "Image"=w206) -> ("Image Out"=w204:T1)  [unwired: 4 in, 5 out]
            n100 = case shown="True" "Save Video" {
              tunnel: w211 -> [_ w269]
              tunnel: w204 -> [_ w268]
              frame False {
              }
              frame True {
                n101 = call "IMAQ AVI Write Frame"("Image"=w268, "Avi Refnum"=w269) -> ()  [unwired: 2 in, 8 out]
              }
            }
            n102 = case shown="False" "Save Image" {
              tunnel: w209 -> [_ w284]
              tunnel: w208 -> [_ w283]
              frame False {
              }
              frame True {
                n103 = call <vilib>:"Flatten Pixmap.vi"("colors"=w283, "8-bit pixmap"=w284) -> ("image data"=w290:T17)  [unwired: 4 in, 5 out]
                n104 = call "Create new save file.vi"("Insert"="video_frame_" ("string"), "Ext"=".bmp" ("string"), "Index In"="Image Index") -> ("Path Out"=w286:path, "Index Out"=w291:dbl)
                n105 = Increment(x=w291) -> (x+1=w285:dbl)
                n106 = local write "Image Index"(w285) -> ()
                n107 = call <vilib>:"Write BMP File.vi"("image data"=w290, "path to BMP file"=w286) -> ()  [unwired: 1 in, 9 out]
              }
            }
            n108 = case shown="False" "Target" {
              tunnel: w204 -> [w230 w234]
              tunnel: [w230 w232] -> w203
              frame False {
              }
              frame True {
                n109 = local read "Target coordinates"() -> (w231:cluster{"X1":dbl, "Y1":dbl, "X2":dbl, "Y2":dbl})
                n110 = call "IMAQ Overlay Oval"("Color"=u32 16711680, "Bounding Rectangle"=w231, "Image"=w234) -> ("Image Out"=w232:T1)  [unwired: 7 in, 1 out]
              }
            }
            "Primary Video Display" <- w203
          }
        }
        n111 = node-c288(w165) -> ()  [unwired: 1 out]
      }
      n112 = node-c288(w149) -> ()  [unwired: 1 out]
      n113 = call "DMR_CloseDevice2.vi"("driver handle IN"=w154) -> ()  [unwired: 3 in, 2 out]
    }
    frame #4 {
      n114 = call "DMR_Close.vi"() -> ()  [unwired: 1 out]
    }
  }
  n115 = while {
    tunnel: [w364] -> w84
    tunnel: [w538] -> w85
    tunnel: [w362] -> w83
    tunnel: [w646] -> w80
    tunnel: w38 -> [w349]
    tunnel: w37 -> [w642]
    tunnel: w36 -> [w647]
    stop <- w646 stop-if-true
    w401 = "NI_ChannelName" ("name")
    w305 = "NI_ChannelName" ("name")
    w466 = -1
    # "Negate these value to make Force feedback work in X. 6-14-18 A.T."
    # "BX - AX"
    # "BY - AY"
    # "Scan # counter"
    # "DAQ loop iteration\ncounter (for timing)"
    # "Step counter"
    # "Force feedback"
    # "Raster scan"
    # "Rewire everything"
    # "Invert these because changed\nfrom PSD to QPD"
    # "Trap Y"
    # "Trap X"
    # "Convert to\npN"
    # "Convert to\nnm"
    # "Subtract\noffset"
    # "Normalize by\nsum"
    # "B sum"
    # "BX"
    # "BY"
    # "AX"
    # "AY"
    # "A sum"
    # "Close files when done saving"
    n116 = disable-structure shown="Disabled" {
      frame Disabled {
        n117 = property class="DAQmx Read"() -> ("AvailSampPerChan"=→"AvailSampPerChan 2":u32)  [unwired: 2 in, 2 out]
      }
      frame Enabled {
      }
    }
    n118 = local read "Averaging Number"() -> (w372:i32)
    n119 = local read "Averaging Number"() -> (w374:i32)
    "# Samples/channel" <- w374
    n120 = local read "Sampling Rate"() -> (w645:dbl)
    n121 = call-poly <vilib>:"DAQmx Read.vi"("task/channels in"=w349, "number of samples per channel"=w372, "timeout"=10.0) -> ("task out"=w348:refnum<k21>, "data"=w373:dbl[][], "error out"=w467:errorcluster)  [unwired: 10 in]
    n122 = Unbundle By Name(w467) -> ("status"=w586:bool)
    n123 = Divide(x=w645, y="Cal Averaging") -> (x/y=→"Cal Final Sampling Rate":dbl)
    n124 = Divide(x=w645, y=w374) -> (x/y=→"Final Sampling Rate" →"# Samples/channel/s":dbl)
    n125 = Index Array(array=w373, index (row)=4) -> (element=w463:dbl[])  [unwired: 1 in]
    n126 = disable-structure shown="Disabled" {
      frame Disabled {
        n127 = local read "Buffer size\n(Samples/channel)"() -> (w664:u32)
        n128 = property class="DAQmx Read"() -> ("AvailSampPerChan"=w665:u32)  [unwired: 2 in, 2 out]
        "AvailSampPerChan" <- w665
        n129 = Divide(x=w665, y=w664) -> (x/y=→"Buffer status":dbl)
      }
      frame Enabled {
      }
    }
    n130 = Index Array(array=w373, index (row)=5) -> (element=w462:dbl[])  [unwired: 1 in]
    n131 = Index Array(array=w373, index (row)=0) -> (element=w324:dbl[])  [unwired: 1 in]
    n132 = Index Array(array=w373, index (row)=3) -> (element=w323:dbl[])  [unwired: 1 in]
    n133 = Index Array(array=w373, index (row)=1) -> (element=w322:dbl[])  [unwired: 1 in]
    n134 = Index Array(array=w373, index (row)=7) -> (element=w320:dbl[])  [unwired: 1 in]
    n135 = Index Array(array=w373, index (row)=2) -> (element=w325:dbl[])  [unwired: 1 in]
    n136 = Index Array(array=w373, index (row)=6) -> (element=w321:dbl[])  [unwired: 1 in]
    n137 = case shown="True" w586 {
      frame False {
      }
      frame True {
        n138 = call <vilib>:"Beep.vi"() -> ()  [unwired: 12 in]
        "Buffer Overflow" <- TRUE
      }
    }
    n139 = Divide(x=w325, y=w321) -> (x/y=w319:dbl[])
    n140 = Divide(x=w324, y=w321) -> (x/y=w318:dbl[])
    n141 = Divide(x=w323, y=w320) -> (x/y=w317:dbl[])
    n142 = Divide(x=w322, y=w320) -> (x/y=w316:dbl[])
    n143 = local read "Cal values"() -> (w578:T2)
    n144 = Build Array(w319, w318, w317, w316) -> (w315:dbl[][])
    n145 = Unbundle(w578) -> ("AX alpha"=w566:dbl, "BX alpha"=w562:dbl, "AX kappa"=w558:dbl, "BX kappa"=w554:dbl, "AX offset"=w572:dbl, "BX offset"=w570:dbl, "AY alpha"=w569:dbl, "BY alpha"=w564:dbl, "AY kappa"=w560:dbl, "BY kappa"=w556:dbl, "AY offset"=w576:dbl, "BY offset"=w574:dbl)
    n146 = Multiply(x=w322, y=w466) -> (x*y=w464:dbl[])
    n147 = Multiply(x=w324, y=w466) -> (x*y=w465:dbl[])
    n148 = local write "AX alpha"(w566) -> ()
    n149 = local write "BY offset"(w574) -> ()
    n150 = Build Array(w465, w325, w464, w323, w321, w320, w463, w462) -> (w398:dbl[][])
    n151 = local write "BX alpha"(w562) -> ()
    n152 = case shown="True" "Reset data stream" {
      selector: "Reset data stream" -> [_ w813]
      tunnel: w348 -> [w805 w811]
      tunnel: [w805 w809] -> w538
      tunnel: w467 -> [w804 w808]
      tunnel: [w804 w806] -> _
      frame False {
      }
      frame True {
        n153 = Not(x=w813) -> (.not. x?=w812:bool)
        n154 = call <vilib>:"DAQmx Stop Task.vi"("task/channels in"=w811, "error in"=w808) -> ("task out"=w810:refnum<k21>, "error out"=w807:errorcluster)  [unwired: 12 in]
        n155 = local write "Reset data stream"(w812) -> ()
        n156 = local write "Buffer Overflow"(w812) -> ()
        n157 = call <vilib>:"DAQmx Start Task.vi"("task/channels in"=w810, "error in"=w807) -> ("task out"=w809:refnum<k21>, "error out"=w806:errorcluster)  [unwired: 12 in]
      }
    }
    n158 = call-poly <vilib>:"Mean.vi"("X"=w462) -> ("mean"=w592:dbl)  [unwired: 1 out]
    n159 = local write "AY offset"(w576) -> ()
    n160 = call-poly <vilib>:"Mean.vi"("X"=w463) -> ("mean"=w593:dbl)  [unwired: 1 out]
    n161 = call-poly <vilib>:"Mean.vi"("X"=w325) -> ("mean"=w599:dbl)  [unwired: 1 out]
    n162 = call-poly <vilib>:"Mean.vi"("X"=w323) -> ("mean"=w597:dbl)  [unwired: 1 out]
    n163 = call-poly <vilib>:"Mean.vi"("X"=w321) -> ("mean"=w596:dbl)  [unwired: 1 out]
    n164 = call-poly <vilib>:"Mean.vi"("X"=w320) -> ("mean"=w595:dbl)  [unwired: 1 out]
    n165 = local read "Averaging Number"() -> (w371:i32)
    n166 = local write "BY kappa"(w556) -> ()
    n167 = local write "AX kappa"(w558) -> ()
    n168 = call-poly <vilib>:"Mean.vi"("X"=w464) -> ("mean"=w598:dbl)  [unwired: 1 out]
    n169 = local write "AY kappa"(w560) -> ()
    n170 = call-poly <vilib>:"Mean.vi"("X"=w465) -> ("mean"=w600:dbl)  [unwired: 1 out]
    n171 = local read "DAQ rate\n(Samples/s)"() -> (w377:dbl)
    n172 = Build Array(w593, w592) -> (w591:dbl[])
    n173 = local write "BX kappa"(w554) -> ()
    n174 = local write "BY alpha"(w564) -> ()
    n175 = local write "AX offset"(w572) -> ()
    n176 = local write "BX offset"(w570) -> ()
    n177 = local write "AY alpha"(w569) -> ()
    n178 = Build Array(w600, w599, w598, w597, w596, w595) -> (w589:dbl[])
    n179 = local read "Total raster time (s)"() -> (w345:dbl)
    n180 = Divide(x=w371, y=w377) -> (x/y=w341:dbl)
    "Data update period (s/set)" <- w341
    n181 = Reciprocal(x=w377) -> (1/x=w378:dbl)
    "Data period (s)" <- w378
    n182 = Divide(x=w345, y=w341) -> (x/y=w344:dbl)
    n183 = Divide(x="Cal time (s)", y=w341) -> (x/y=w340:dbl)
    n184 = Divide(x=w600, y=w596) -> (x/y=w630:dbl)
    n185 = Divide(x=w599, y=w596) -> (x/y=w336:dbl)
    n186 = Round Toward -Infinity(1:w344) -> (0:w343:dbl)
    n187 = Divide(x=w598, y=w595) -> (x/y=w637:dbl)
    n188 = Divide(x=w597, y=w595) -> (x/y=w338:dbl)
    n189 = Round Toward -Infinity(1:w340) -> (0:→"Cal sets to save":dbl)
    n190 = local write "N sets to be saved"(w343) -> ()
    n191 = Build Array("Force Feedback 1", "Force Feedback 2") -> (w301:bool[])
    n192 = Boolean Array To Number(Boolean array=w301) -> (number=w300:u32)
    n193 = Negate(x=w336) -> (-x=w335:dbl)
    n194 = Negate(x=w338) -> (-x=w337:dbl)
    n195 = Subtract(x=w630, y="AY offset") -> (x-y=w612:dbl)
    n196 = Subtract(x=w336, y="AX offset") -> (x-y=w613:dbl)
    n197 = Subtract(x=w637, y="BY offset") -> (x-y=w611:dbl)
    n198 = Subtract(x=w338, y="BX offset") -> (x-y=w614:dbl)
    n199 = Subtract(x=w637, y=w630) -> (x-y=w628:dbl)
    n200 = Subtract(x=w337, y=w335) -> (x-y=w629:dbl)
    n201 = feedback #4(0.0) -> (w537:dbl)
    n202 = Multiply(x="Downsamp\nfact", y=w378) -> (x*y=w313:dbl)
    n203 = Multiply(x=w612, y="AY alpha") -> (x*y=w546:dbl)
    n204 = Multiply(x=w613, y="AX alpha") -> (x*y=w544:dbl)
    n205 = Multiply(x=w614, y="BX alpha") -> (x*y=w545:dbl)
    n206 = Multiply(x=w611, y="BY alpha") -> (x*y=w547:dbl)
    n207 = Add(x=w341, y=w537) -> (x+y=w535:dbl)
    n208 = feedback-in #4(w535) -> ()
    n209 = Square(x=w546) -> (x^2=w622:dbl)
    n210 = Square(x=w544) -> (x^2=w623:dbl)
    n211 = Square(x=w547) -> (x^2=w624:dbl)
    n212 = Square(x=w545) -> (x^2=w625:dbl)
    n213 = Bundle(w628, w629) -> (w332:cluster{dbl, dbl})  [unwired: 1 in]
    n214 = case shown="True" "Set reading to\nsetpoint 1" {
      tunnel: w332 -> [_ w802]
      frame False {
      }
      frame True {
        n215 = property on="Setpoint voltage 1" class="Clust (strict)"("Val(Sgnl)"=w802) -> ()  [unwired: 2 in, 2 out]
        n216 = local read "Trap position (V)"() -> (w801:cluster{"X":dbl, "Y":dbl})
        n217 = local write "Set reading to\nsetpoint 1"(FALSE ("Set reading to\nsetpoint")) -> ()
        n218 = Unbundle(w801) -> ("X"=w800:dbl, "Y"=w799:dbl)
        n219 = Bundle("Y"=w799, "X"=w800) -> (w798:cluster{"Y":dbl, "X":dbl})  [unwired: 1 in]
        n220 = property on="Offset 1" class="Clust (strict)"("Val(Sgnl)"=w798) -> ()  [unwired: 2 in, 2 out]
      }
    }
    n221 = Reciprocal(x=w313) -> (1/x=→"Chart Freq (Hz)":dbl)
    n222 = To Time Stamp(1:w535) -> (0:w312:timestamp)
    n223 = Add(x=w622, y=w623) -> (x+y=w626:dbl)
    n224 = Add(x=w624, y=w625) -> (x+y=w636:dbl)
    n225 = Multiply(x=w544, y="AX kappa") -> (x*y=w540:dbl)
    n226 = Bundle("A y", "A x", "B y", "B x", "A sum", "B sum", "Trap x", "Trap y") -> (w526:T20)  [unwired: 1 in]
    n227 = Multiply(x=w545, y="BX kappa") -> (x*y=w541:dbl)
    n228 = Square Root(x=w626) -> (sqrt(x)=w640:dbl)
    n229 = Square Root(x=w636) -> (sqrt(x)=w639:dbl)
    n230 = Multiply(x=w546, y="AY kappa") -> (x*y=w542:dbl)
    n231 = Multiply(x=w547, y="BY kappa") -> (x*y=w543:dbl)
    n232 = Subtract(x=w592, y="Fixed Y") -> (x-y=w627:dbl)
    n233 = Subtract(x=w593, y="Fixed X") -> (x-y=w631:dbl)
    n234 = Cluster To Array(cluster=w526) -> (array=w525:string[])
    n235 = for {
      tunnel: w398 -> [w791] mode=indexing
      tunnel: w313 -> [w790]
      tunnel: "Downsamp\nfact" -> [w796]
      tunnel: [w794] -> w331 mode=indexing
      tunnel: w312 -> [w797]
      tunnel: w525 -> [w793] mode=indexing
      tunnel: w305 -> [w792]
      n236 = call "Downsample 1D array.vi"("Ave N"=w796, "Arrray In"=w791) -> ("Array Out"=w789:dbl[])  [unwired: 9 in]
      n237 = Bundle By Name("Y"=w789, "dt"=w790, "t0"=w797) -> (w795:waveform(dbl))  [unwired: 1 in]
      n238 = Set Waveform Attribute(5:w793, 6:w792, 7:w795) -> (3:w794:waveform(dbl))  [unwired: 1 in, 2 out]
    }
    "All signals" <- w331
    n239 = Square(x=w542) -> (x^2=w615:dbl)
    n240 = Square(x=w540) -> (x^2=w616:dbl)
    n241 = Square(x=w543) -> (x^2=w617:dbl)
    n242 = Square(x=w541) -> (x^2=w618:dbl)
    n243 = Add(x=w615, y=w616) -> (x+y=w619:dbl)
    n244 = Add(x=w617, y=w618) -> (x+y=w620:dbl)
    n245 = Multiply(x=w627, y="Conv Y (nm/V)") -> (x*y=w549:dbl)
    n246 = Multiply(x=w631, y="Conv X (nm/V)") -> (x*y=w550:dbl)
    n247 = feedback #5() -> (w587:cluster{"B_Y":dbl, "B_X":dbl})  [unwired: 1 in]
    n248 = case shown="0, Default" w300 {
      tunnel: [w1150 w1167 w1177] -> w365
      tunnel: [w1149 w1166 w1178] -> w363
      tunnel: w332 -> [_ w1165 w1180]
      tunnel: [cluster{"B_Y":dbl, "B_X":dbl} {"B_Y"=0.0, "B_X"=0.0} ("Sum error past") w1159 w1175] -> w588
      tunnel: w587 -> [_ w1164 w1176]
      tunnel: w642 -> [w1150 w1162 w1171]
      tunnel: w647 -> [w1149 w1161 w1179]
      tunnel: [0.0 ("B_X") w1154 w1169] -> w298
      tunnel: [cluster{"B_Y":dbl, "B_X":dbl} {"B_Y"=0.0, "B_X"=0.0} ("Sum error past") w1153 w1168] -> w297
      tunnel: "Feedback const" -> [_ w1152 w1170]
      frame 0, Default {
        # "Force feedback"
      }
      frame 1 {
        n249 = local write "Force Feedback 2"(FALSE) -> ()
        n250 = call "ForceFeedback2.vi"("PSD/Mirror Voltages"=w1165, "Sum error"=w1164, "task/channels in"=w1162, "error in"=w1161, "Desired voltage"="Setpoint voltage 1", "Feedback const"=w1152, "offset"="Offset 1") -> ("task out"=w1167:refnum<k21>, "Sum error past"=w1159:cluster{"B_Y":dbl, "B_X":dbl}, "Output Voltage"=w1153:cluster{dbl, dbl}, "error out"=w1166:errorcluster)  [unwired: 8 in, 1 out]
        n251 = local read "Pulling direction"() -> (w1158:bool)
        n252 = Unbundle(w1159) -> ("B_Y"=w1157:dbl, "B_X"=w1156:dbl)
        n253 = Select(t=w1157, s=w1158, f=w1156) -> (s? t:f=w1154:dbl)
      }
      frame 2 {
        n254 = local write "Force Feedback 1"(FALSE) -> ()
        n255 = call "ForceFeedback2.vi"("PSD/Mirror Voltages"=w1180, "Sum error"=w1176, "task/channels in"=w1171, "error in"=w1179, "Desired voltage"="Setpoint voltage 2", "Feedback const"=w1170, "offset"="Offset 2") -> ("task out"=w1177:refnum<k21>, "Sum error past"=w1175:cluster{"B_Y":dbl, "B_X":dbl}, "Output Voltage"=w1168:cluster{dbl, dbl}, "error out"=w1178:errorcluster)  [unwired: 8 in, 1 out]
        n256 = local read "Pulling direction"() -> (w1172:bool)
        n257 = Unbundle(w1175) -> ("B_Y"=w1174:dbl, "B_X"=w1173:dbl)
        n258 = Select(t=w1174, s=w1172, f=w1173) -> (s? t:f=w1169:dbl)
      }
    }
    "Sum error" <- w298
    "Feedback Output \nVoltage 2" <- w297
    n259 = feedback-in #5(w588) -> ()
    n260 = Square Root(x=w619) -> (sqrt(x)=w548:dbl)
    n261 = Square Root(x=w620) -> (sqrt(x)=w641:dbl)
    n262 = Add(x=w548, y=w641) -> (x+y=w621:dbl)
    n263 = case shown="True" "Set reading to\nsetpoint 2" {
      tunnel: w332 -> [_ w659]
      frame False {
      }
      frame True {
        n264 = local read "Trap position (V)"() -> (w662:cluster{"X":dbl, "Y":dbl})
        n265 = property on="Setpoint voltage 2" class="Clust (strict)"("Val(Sgnl)"=w659) -> ()  [unwired: 2 in, 2 out]
        n266 = local write "Set reading to\nsetpoint 2"(FALSE) -> ()
        n267 = Unbundle(w662) -> ("X"=w661:dbl, "Y"=w660:dbl)
        n268 = Bundle("Y"=w660, "X"=w661) -> (w658:cluster{"Y":dbl, "X":dbl})  [unwired: 1 in]
        n269 = property on="Offset 2" class="Clust (strict)"("Val(Sgnl)"=w658) -> ()  [unwired: 2 in, 2 out]
      }
    }
    n270 = Build Array(w630, w336, w637, w338, w596, w595, w548, w641, w640, w639, w550, w549) -> ()  [unwired: 1 out]
    n271 = Divide(x=w621, y=2.0) -> (x/y=w585:dbl)
    n272 = Bundle("AX/Asum", "AY/Asum", "BX/Bsum", "BY/Bsum") -> (w307:cluster{string, string, string, string})  [unwired: 1 in]
    n273 = Index Array(array=w331, index=6) -> (element=w403:waveform(dbl))
    n274 = Index Array(array=w331, index=7) -> (element=w405:waveform(dbl))
    n275 = Cluster To Array(cluster=w307) -> (array=w306:string[])
    n276 = for {
      tunnel: w315 -> [w657] mode=indexing
      tunnel: "Downsamp\nfact" -> [w656]
      tunnel: w313 -> [w655]
      tunnel: w312 -> [w653]
      tunnel: w306 -> [w651] mode=indexing
      tunnel: w305 -> [w650]
      tunnel: [w649] -> w304 mode=indexing
      n277 = call "Downsample 1D array.vi"("Ave N"=w656, "Arrray In"=w657) -> ("Array Out"=w654:dbl[])  [unwired: 9 in]
      n278 = Bundle By Name("Y"=w654, "dt"=w655, "t0"=w653) -> (w652:waveform(dbl))  [unwired: 1 in]
      n279 = Set Waveform Attribute(5:w651, 6:w650, 7:w652) -> (3:w649:waveform(dbl))  [unwired: 1 in, 2 out]
    }
    "All signals 2" <- w304
    n280 = local read "Fixed X"() -> (w452:dbl)
    n281 = local read "Fixed Y"() -> (w454:dbl)
    n282 = Unbundle By Name(w403) -> ("Y"=w456:dbl[])
    n283 = Unbundle By Name(w405) -> ("Y"=w455:dbl[])
    n284 = Index Array(array=w331, index=0) -> (element=w410:waveform(dbl))
    n285 = Index Array(array=w331, index=1) -> (element=w522:waveform(dbl))
    n286 = Index Array(array=w331, index=4) -> (element=w516:waveform(dbl))
    n287 = Subtract(x=w456, y=w452) -> (x-y=w453:dbl[])
    n288 = Subtract(x=w455, y=w454) -> (x-y=w450:dbl[])
    n289 = Unbundle By Name(w410) -> ("Y"=w514:dbl[])
    n290 = Unbundle By Name(w522) -> ("Y"=w513:dbl[])
    n291 = Unbundle By Name(w516) -> ("Y"=w512:dbl[])
    n292 = Index Array(array=w331, index=5) -> (element=w515:waveform(dbl))
    n293 = local read "Conv X (nm/V)"() -> (w451:dbl)
    n294 = local read "Conv Y (nm/V)"() -> (w449:dbl)
    n295 = Index Array(array=w331, index=2) -> (element=w326:waveform(dbl))
    n296 = Index Array(array=w331, index=3) -> (element=w519:waveform(dbl))
    n297 = Set Waveform Attribute(5:"T2 X", 6:w401, 7:w403) -> (3:w402:waveform(dbl))  [unwired: 1 in, 2 out]
    n298 = Set Waveform Attribute(5:"T2 Y", 6:w401, 7:w405) -> (3:w404:waveform(dbl))  [unwired: 1 in, 2 out]
    n299 = Unbundle By Name(w515) -> ("Y"=w509:dbl[])
    n300 = Unbundle By Name(w326) -> ("Y"=w511:dbl[])
    n301 = Unbundle By Name(w519) -> ("Y"=w510:dbl[])
    n302 = Divide(x=w514, y=w512) -> (x/y=w330:dbl[])
    n303 = Divide(x=w513, y=w512) -> (x/y=w329:dbl[])
    n304 = local read "AY offset"() -> (w500:dbl)
    n305 = local read "AX offset"() -> (w498:dbl)
    n306 = Multiply(x=w453, y=w451) -> (x*y=w395:dbl[])
    n307 = Multiply(x=w450, y=w449) -> (x*y=w397:dbl[])
    n308 = Divide(x=w510, y=w509) -> (x/y=w327:dbl[])
    n309 = Subtract(x=w329, y=w498) -> (x-y=w501:dbl[])
    n310 = local read "BX offset"() -> (w508:dbl)
    n311 = Subtract(x=w330, y=w500) -> (x-y=w502:dbl[])
    n312 = Divide(x=w511, y=w509) -> (x/y=w328:dbl[])
    n313 = local read "AY alpha"() -> (w499:dbl)
    n314 = local read "AX alpha"() -> (w497:dbl)
    n315 = call-poly <vilib>:"Mean.vi"("X"=w397) -> ("mean"=w432:dbl)  [unwired: 1 out]
    "Mean Trp Pos Y 2 (nm)" <- w432
    n316 = Subtract(x=w328, y=w330) -> (x-y=w422:dbl[])
    n317 = Subtract(x=w327, y=w329) -> (x-y=w421:dbl[])
    n318 = local read "BY offset"() -> (w505:dbl)
    n319 = Subtract(x=w395, y="Offset X (nm)") -> (x-y=w394:dbl[])
    n320 = Subtract(x=w397, y="Offset Y (nm)") -> (x-y=w396:dbl[])
    n321 = Subtract(x=w328, y=w505) -> (x-y=w507:dbl[])
    n322 = Subtract(x=w327, y=w508) -> (x-y=w506:dbl[])
    n323 = Subtract(x=w432, y=w397) -> (x-y=w431:dbl[])
    n324 = call-poly <vilib>:"Mean.vi"("X"=w395) -> ("mean"=w436:dbl)  [unwired: 1 out]
    "Mean Trap Pos X 2 (nm)" <- w436
    n325 = Build Array(w422, w421) -> (w419:dbl[][])
    n326 = Index Array(array=w419, index (row)=0) -> (element=w417:dbl[])  [unwired: 1 in]
    n327 = Index Array(array=w419, index (row)=1) -> (element=w416:dbl[])  [unwired: 1 in]
    n328 = call-poly <vilib>:"Mean.vi"("X"=w417) -> ("mean"=w415:dbl)  [unwired: 1 out]
    n329 = call-poly <vilib>:"Mean.vi"("X"=w416) -> ("mean"=w414:dbl)  [unwired: 1 out]
    n330 = Bundle("mean"=w415, "mean"=w414) -> ()  [unwired: 1 in, 1 out]
    n331 = local read "BX alpha"() -> (w503:dbl)
    n332 = Multiply(x=w502, y=w499) -> (x*y=w490:dbl[])
    n333 = Multiply(x=w501, y=w497) -> (x*y=w489:dbl[])
    n334 = Square(x=w431) -> (x^2=w430:dbl[])
    n335 = Subtract(x=w436, y=w395) -> (x-y=w435:dbl[])
    n336 = Bundle By Name(cluster=w404, "Y"=w396) -> (w447:waveform(dbl))
    n337 = Bundle By Name(cluster=w402, "Y"=w394) -> (w448:waveform(dbl))
    n338 = local read "BY alpha"() -> (w504:dbl)
    n339 = local read "Raster scanning..."() -> (w347:bool)
    n340 = local read "Saving"() -> (w551:bool)
    n341 = local read "Tether"() -> (w552:bool)
    n342 = Square(x=w435) -> (x^2=w434:dbl[])
    n343 = call-poly <vilib>:"Mean.vi"("X"=w430) -> ("mean"=w429:dbl)  [unwired: 1 out]
    n344 = Square(x=w490) -> (x^2=w496:dbl[])
    n345 = Multiply(x=w507, y=w504) -> (x*y=w488:dbl[])
    n346 = Square(x=w489) -> (x^2=w495:dbl[])
    n347 = Multiply(x=w506, y=w503) -> (x*y=w487:dbl[])
    n348 = Less?(x=w585, y="Tether break\nforce (pN)") -> (x < y?=w583:bool)
    n349 = call-poly <vilib>:"Mean.vi"("X"=w434) -> ("mean"=w433:dbl)  [unwired: 1 out]
    n350 = Build Array(w448, w447) -> (w366:waveform(dbl)[])
    "Trap sep" <- w366
    n351 = Square Root(x=w429) -> (sqrt(x)=w428:dbl)
    n352 = Square(x=w488) -> (x^2=w494:dbl[])
    n353 = Square(x=w487) -> (x^2=w493:dbl[])
    n354 = Add(x=w496, y=w495) -> (x+y=w492:dbl[])
    n355 = Square Root(x=w433) -> (sqrt(x)=w426:dbl)
    n356 = Compound Arithmetic op=AND(w551, w552, w583) -> (w582:bool)
    n357 = Multiply(x=w428, y=10) -> (x*y=→"T2 Y RMS (A)":dbl)
    n358 = Square Root(x=w492) -> (sqrt(x)=w390:dbl[])
    n359 = Add(x=w494, y=w493) -> (x+y=w491:dbl[])
    n360 = Set Waveform Attribute(5:"T2", 6:"NI_ChannelName" ("name"), 7:w410) -> (3:w409:waveform(dbl))  [unwired: 1 in, 2 out]
    n361 = Set Waveform Attribute(5:"T1", 6:"NI_ChannelName" ("name"), 7:w326) -> (3:w407:waveform(dbl))  [unwired: 1 in, 2 out]
    n362 = case shown="True" w582 {
      selector: w582 -> [_ w820]
      tunnel: w347 -> [w814 w816]
      tunnel: [w814 w816] -> w346
      frame False {
      }
      frame True {
        n363 = stacked-sequence {
          frame #0 {
            n364 = local write "Cancel Rep\n Dip"(TRUE ("Cancel Rep\n Dip")) -> ()
          }
          frame #1 {
            n365 = local write "Cancel Rep\n Dip"(FALSE ("Cancel Rep\n Dip")) -> ()
          }
        }
        n366 = call <vilib>:"Beep.vi"() -> ()  [unwired: 12 in]
        n367 = Not(x=w820) -> (.not. x?=w815:bool)
        n368 = And(x=w816, y="Fish After TA?") -> (x .and. y?=w818:bool)
        n369 = local write "Force Feedback 1"(w815) -> ()
        n370 = local write "Tether"(w815) -> ()
        n371 = case shown="True" w818 {
          selector: w818 -> [_ w823]
          frame False {
          }
          frame True {
            n372 = property on="Fish" class="Bool (strict)"("Val(Sgnl)"=w823) -> ()  [unwired: 2 in, 2 out]
          }
        }
        n373 = local write "Force Feedback 2"(w815) -> ()
        n374 = property on="Stop saving" class="Bool (strict)"("Val(Sgnl)"="TA Cancel Save?") -> ()  [unwired: 2 in, 2 out]
      }
    }
    n375 = Square Root(x=w491) -> (sqrt(x)=w389:dbl[])
    n376 = Multiply(x=w426, y=10) -> (x*y=→"T2 X RMS (A)":dbl)
    n377 = Bundle By Name(cluster=w409, "Y"=w390) -> (w413:waveform(dbl))
    n378 = Bundle By Name(cluster=w407, "Y"=w389) -> (w469:waveform(dbl))
    n379 = Add(x=w390, y=w389) -> (x+y=w388:dbl[])
    n380 = case shown="True" "Remove offsets" {
      selector: "Remove offsets" -> [_ w787]
      frame False {
      }
      frame True {
        n381 = local read "Mean Trp Pos Y 2 (nm)"() -> (w785:dbl)
        n382 = Not(x=w787) -> (.not. x?=w788:bool)
        n383 = local read "Mean Trap Pos X 2 (nm)"() -> (w786:dbl)
        n384 = local write "Remove offsets"(w788) -> ()
        n385 = local write "Offset Y (nm)"(w785) -> ()
        n386 = local write "Offset X (nm)"(w786) -> ()
      }
    }
    n387 = Build Array(w413, w469) -> (→"Bead sep":waveform(dbl)[])
    n388 = local read "AY kappa"() -> (w486:dbl)
    n389 = local read "AX kappa"() -> (w485:dbl)
    n390 = Divide(x=w388, y=2) -> (x/y=w386:dbl[])
    n391 = local read "BX kappa"() -> (w483:dbl)
    n392 = local read "BY kappa"() -> (w484:dbl)
    n393 = call-poly <vilib>:"Mean.vi"("X"=w386) -> ("mean"=w385:dbl)  [unwired: 1 out]
    "Mean Bead Sep\n(nm)" <- w385
    n394 = local read "Calibrating"() -> (w299:bool)
    n395 = Multiply(x=w490, y=w486) -> (x*y=w479:dbl[])
    n396 = Multiply(x=w489, y=w485) -> (x*y=w480:dbl[])
    n397 = Square(x=w479) -> (x^2=w478:dbl[])
    n398 = Square(x=w480) -> (x^2=w477:dbl[])
    n399 = Subtract(x=w386, y=w385) -> (x-y=w384:dbl[])
    n400 = Multiply(x=w488, y=w484) -> (x*y=w481:dbl[])
    n401 = Multiply(x=w487, y=w483) -> (x*y=w482:dbl[])
    n402 = Or(x=w346, y="Raster scan") -> (x .or. y?=w361:bool)
    n403 = Add(x=w478, y=w477) -> (x+y=w474:dbl[])
    n404 = Square(x=w384) -> (x^2=w383:dbl[])
    n405 = Square Root(x=w474) -> (sqrt(x)=w446:dbl[])
    n406 = Square(x=w481) -> (x^2=w476:dbl[])
    n407 = Square(x=w482) -> (x^2=w475:dbl[])
    n408 = call-poly <vilib>:"Mean.vi"("X"=w383) -> ("mean"=w382:dbl)  [unwired: 1 out]
    n409 = Add(x=w476, y=w475) -> (x+y=w473:dbl[])
    n410 = Bundle By Name(cluster=w409, "Y"=w446) -> (w472:waveform(dbl))
    n411 = local read "Saving"() -> (w581:bool)
    n412 = Or(x=w299, y=w581) -> ()  [unwired: 1 out]
    n413 = Square Root(x=w382) -> (sqrt(x)=w381:dbl)
    n414 = Square Root(x=w473) -> (sqrt(x)=w445:dbl[])
    n415 = Multiply(x=10, y=w381) -> (x*y=→"Bead Sep Noise\n(A)":dbl)
    n416 = Bundle By Name(cluster=w407, "Y"=w445) -> (w471:waveform(dbl))
    n417 = Add(x=w446, y=w445) -> (x+y=w444:dbl[])
    n418 = Build Array(w472, w471) -> (→"Force (pN)":waveform(dbl)[])
    n419 = Divide(x=w444, y=2) -> (x/y=w441:dbl[])
    n420 = call-poly <vilib>:"Mean.vi"("X"=w441) -> ("mean"=w442:dbl)  [unwired: 1 out]
    "Mean force (pN)" <- w442
    n421 = Subtract(x=w442, y=w441) -> (x-y=w440:dbl[])
    n422 = Square(x=w440) -> (x^2=w439:dbl[])
    n423 = call-poly <vilib>:"Mean.vi"("X"=w439) -> ("mean"=w438:dbl)  [unwired: 1 out]
    n424 = flat-sequence {
      tunnel: w299 -> [w866]
      tunnel: w581 -> [_]
      tunnel: w299 -> [_]
      tunnel: w581 -> [_]
      tunnel: w398 -> [w853]
      tunnel: [w853] -> w602
      tunnel: w467 -> [w852]
      tunnel: [w852] -> w601
      tunnel: w589 -> [w851]
      tunnel: [w851] -> w594
      tunnel: w591 -> [w850]
      tunnel: [w850] -> w590
      tunnel: [w847] -> w580
      tunnel: [w844] -> w579
      tunnel: [w841] -> w461
      tunnel: [w840] -> w460
      tunnel: [w837] -> w459
      tunnel: w368 -> [w834]
      tunnel: ["Save Data"] -> w367
      tunnel: [w827] -> w334
      tunnel: w602 -> [w1047]
      tunnel: w601 -> [w1046]
      tunnel: w594 -> [_]
      tunnel: w590 -> [_]
      tunnel: w580 -> [w1045]
      tunnel: w579 -> [w1044]
      tunnel: w461 -> [w1043]
      tunnel: w460 -> [w1042]
      tunnel: w459 -> [w1041]
      tunnel: w367 -> [w1040]
      tunnel: w366 -> [w1039]
      tunnel: w334 -> [w1037]
      frame #0 {
        w833 = 0.0
        # "1: old trap\n0: fleezers"
        # "Create files if saving data"
        n425 = local read "Save N sets"() -> (w836:bool)
        n426 = local read "Fixed X"() -> (w832:dbl)
        n427 = local read "Trap position (V)"() -> (w861:cluster{"X":dbl, "Y":dbl})
        n428 = local read "Fixed Y"() -> (w831:dbl)
        n429 = local read "Sampling Rate"() -> (w864:dbl)
        n430 = Or(x=w836, y="Save Data") -> (x .or. y?=w835:bool)
        n431 = Build Array(w835, "Save cal", w834) -> (w855:bool[])
        n432 = Compound Arithmetic op=OR("Save Data", "Save cal", w834) -> (w857:bool)
        n433 = Boolean Array To Number(Boolean array=w855) -> (number=w854:u32)
        n434 = Unbundle(w861) -> ("X"=w830:dbl, "Y"=w829:dbl)
        n435 = Build Array(w830, w829, w832, w831, w833, w833) -> (w860:dbl[])
        n436 = feedback #6(refnum<k0> refnum) -> (w826:refnum<file>)
        n437 = feedback #7(0) -> (w858:i32)
        n438 = feedback #8(refnum<k0> refnum) -> (w848:refnum<file>)
        n439 = feedback #9() -> (w842:dbl)  [unwired: 1 in]
        n440 = feedback #10(FALSE) -> (w838:bool)
        n441 = feedback #11(refnum<k0> refnum) -> (w845:refnum<file>)
        n442 = case shown="True" w857 {
          tunnel: w866 -> [_ _]
          tunnel: 9 -> [_ w912]
          tunnel: w864 -> [_ w911]
          tunnel: 6 -> [_ w910]
          tunnel: 5 -> [_ w909]
          tunnel: w860 -> [_ w908]
          tunnel: [w872 1] -> w841
          tunnel: w858 -> [w873 _]
          tunnel: w854 -> [_ w884]
          tunnel: [w871 w883] -> w847
          tunnel: w848 -> [w871 _]
          tunnel: [w870 w882] -> w844
          tunnel: w845 -> [w870 _]
          tunnel: 1.0 -> [_ w881]
          tunnel: [w869 w880] -> w840
          tunnel: w842 -> [w869 _]
          tunnel: [w868 w879] -> w837
          tunnel: w838 -> [w868 _]
          tunnel: [w867 w874] -> w827
          tunnel: w826 -> [w867 _]
          frame False {
            n443 = Increment(x=w873) -> (x+1=w872:i32)
          }
          frame True {
            w885 = FALSE ("Save Data")
            w890 = FALSE
            w891 = T19."big-endian, network order" ("byte order (0:big-endian, network order)")
            n444 = local write "Save cal"(w885) -> ()
            n445 = local write "Save Data"(w885) -> ()
            n446 = case shown="1, Default" w884 {
              tunnel: w912 -> [w987 w1005 w1036]
              tunnel: w911 -> [w966 w1004 w1013]
              tunnel: w910 -> [w986 w1002 w1032]
              tunnel: w909 -> [w985 w1001 w1031]
              tunnel: w908 -> [w984 w998 w1028]
              tunnel: [w983 w997 w1017] -> w905
              tunnel: [w964 w988 w1008] -> w879
              tunnel: ["Averaging Number" 200 w1015] -> _
              tunnel: w881 -> [w971 w990 w1014]
              tunnel: [w967 w989 w1009] -> w880
              tunnel: [w964 w988 w1007] -> w876
              frame 1, Default {
                w964 = TRUE
                w972 = 0.0
                # "stage x,yz"
                # "Save N number/length of data. e.g. N =200 \nwill give only 200 long data points"
                # "Time trace"
                n447 = Boolean To (0,1)(Boolean=w964) -> (0, 1=w977:i16)
                n448 = local read "Averaging Number"() -> (w982:i32)
                n449 = Increment(x=w977) -> (x+1=w976:i16)
                n450 = Divide(x=w966, y=w982) -> (x/y=w981:dbl)
                n451 = To Double Precision Float(number=w976) -> (double precision float=w975:dbl)
                n452 = Reciprocal(x=w981) -> (1/x=w980:dbl)
                n453 = Reciprocal(x=w966) -> (1/x=w965:dbl)
                n454 = Build Array(w987, w965, w980, w986, w985, 0 ("f")) -> (w979:dbl[])
                n455 = Build Array(w975, w971, w972, w972, w972) -> (w978:dbl[])
                n456 = Build Array (concatenate)(w979, w984, w978) -> (w983:dbl[])
                n457 = Select(t="N sets", s="Save N sets", f=2147483647) -> (s? t:f=w967:i32)
              }
              frame 2 {
                w988 = FALSE
                w993 = 0.0
                # "Calibration file"
                n458 = Reciprocal(x=w1004) -> (1/x=w1003:dbl)
                n459 = Boolean To (0,1)(Boolean=w988) -> (0, 1=w996:i16)
                n460 = To Double Precision Float(number=w996) -> (double precision float=w995:dbl)
                n461 = Build Array(w1005, w1003, w1003, w1002, w1001, 1) -> (w999:dbl[])
                n462 = Build Array(w995, w990, w993, w993, w993) -> (w994:dbl[])
                n463 = Build Array (concatenate)(w999, w998, w994) -> (w997:dbl[])
                n464 = local read "Cal sets to save"() -> (w989:i32)
                "Calibrating" <- TRUE ("Calibrating")
              }
              frame 4 {
                w1006 = FALSE ("Raster scan")
                w1024 = 0.0
                w1008 = TRUE
                # "Not using ncycles"
                # "FX curve"
                n465 = Not(x=w1008) -> (.not. x?=w1007:bool)
                n466 = local read "Averaging Number"() -> (w1035:i32)
                n467 = Boolean To (0,1)(Boolean=w1008) -> (0, 1=w1027:i16)
                n468 = local write "Saving Move"(w1006) -> ()
                n469 = Divide(x=w1013, y=w1035) -> (x/y=w1034:dbl)
                n470 = Increment(x=w1027) -> (x+1=w1026:i16)
                n471 = local write "Raster scan"(w1006) -> ()
                n472 = To Double Precision Float(number=w1026) -> (double precision float=w1025:dbl)
                n473 = Reciprocal(x=w1034) -> (1/x=w1033:dbl)
                n474 = Reciprocal(x=w1013) -> (1/x=w1012:dbl)
                n475 = Build Array(w1025, w1014, w1024, w1024, w1024) -> (w1023:dbl[])
                n476 = Build Array(w1036, w1012, w1033, w1032, w1031, 2) -> (w1029:dbl[])
                n477 = local read "Scan range (V)"() -> (w1010:dbl)
                n478 = local read "Pulling direction"() -> (w1021:bool)
                n479 = local read "Scan steps (mirror)"() -> (w1011:u64)
                n480 = local read "# scans"() -> (w1019:i32)
                n481 = local read "N sets to be saved"() -> (w1009:dbl)
                n482 = Not(x=w1021) -> (.not. x?=w1020:bool)
                n483 = local read "Averaging Number"() -> (w1015:i32)
                n484 = Boolean To (0,1)(Boolean=w1020) -> (0, 1=w1022:i16)
                n485 = Build Array(w1022, w1010, w1011, 0, w1019) -> (w1018:dbl[])
                n486 = Build Array (concatenate)(w1029, w1028, w1023, w1018) -> (w1017:dbl[])
              }
            }
            n487 = call "CreateSaveFile.vi"("Index In"="Save file index", "Ext"=".dat", "Insert"="", "Directory"="Path") -> ("Index Out"=w878:i32, "Path Out"=w875:path)  [unwired: 6 in]
            "Current file name" <- w875
            n488 = case shown="True" w876 {
              tunnel: w875 -> [_ w924]
              tunnel: [refnum<k0> refnum w921] -> w874
              frame False {
              }
              frame True {
                # "SY 190201 \nAdding functionality to get time points of start and stop moves. \nWehn timetrace save data starts save time point"
                n489 = Path To String(path=w924) -> (string=w928:string)
                n490 = Get Date/Time In Seconds() -> (seconds since 1Jan1904=w938:timestamp)
                n491 = String Length(string=w928) -> (length=w925:i32)
                n492 = Subtract(x=w925, y=4) -> (x-y=w927:i32)
                n493 = Format Date/Time String(time format string (%c)="%H:%M:%S%3u", seconds (now)=w938, UTC format=TRUE) -> (date/time string=w922:string)
                n494 = call <vilib>:"Space Constant.vi"() -> ("String"=w916:string)
                n495 = String Subset(string=w928, length (rest)=w927) -> (substring=w929:string)  [unwired: 1 in]
                n496 = Concatenate Strings(w929, "_stagetime.txt" ("string")) -> (w931:string)
                n497 = String To Path(string=w931) -> (path=w932:path)
                n498 = Open/Create/Replace File(file path (use dialog)=w932, operation (0:open)=T18."create", access (0:read/write)=enum16{"read/write", "read-only", "write-only"}."write-only") -> (refnum out=w936:refnum<file>, error out=w935:errorcluster)  [unwired: 3 in, 1 out]
                n499 = Deny Access(4:w935, 7:w936) -> (3:w937:refnum<file>)  [unwired: 1 in, 1 out]
                n500 = Concatenate Strings(w922, w916, "start", "\r\n") -> (w923:string)
                n501 = Write to Text File(file (use dialog)=w937, text=w923) -> (refnum out=w921:refnum<file>)  [unwired: 2 in, 2 out]
                n502 = local write "Move time"(w922) -> ()
                n503 = local read "Raster scanning..."() -> (w919:bool)
                n504 = local read "Calibrating"() -> (w920:bool)
                n505 = Or(x=w920, y=w919) -> (x .or. y?=w918:bool)
                n506 = Not(x=w918) -> (.not. x?=w917:bool)
                n507 = local write "Saving Move"(w917) -> ()
              }
            }
            n508 = Open/Create/Replace File(file path (use dialog)=w875, operation (0:open)=T18."create", access (0:read/write)=enum16{"read/write", "read-only", "write-only"}."write-only") -> (refnum out=w898:refnum<file>, error out=w899:errorcluster)  [unwired: 3 in, 1 out]
            n509 = local write "Save file index"(w878) -> ()
            n510 = Array Size(array=w905) -> (size(s)=w907:i32)
            n511 = case shown="True" w879 {
              tunnel: w875 -> [_ w963]
              tunnel: [refnum<k0> refnum w942] -> w882
              frame False {
              }
              frame True {
                w949 = 0.0
                n512 = Path To String(path=w963) -> (string=w959:string)
                n513 = Build Array(w949, w949, w949, w949, w949, w949, w949, w949) -> (w946:dbl[])
                n514 = String Length(string=w959) -> (length=w962:i32)
                n515 = Array Size(array=w946) -> (size(s)=w948:i32)
                n516 = Subtract(x=w962, y=4) -> (x-y=w960:i32)
                n517 = To Double Precision Float(number=w948) -> (double precision float=w947:dbl)
                n518 = String Subset(string=w959, length (rest)=w960) -> (substring=w958:string)  [unwired: 1 in]
                n519 = Build Array (concatenate)(w947, w946) -> (w945:dbl[])
                n520 = Concatenate Strings(w958, "_pos.dat" ("string")) -> (w956:string)
                n521 = String To Path(string=w956) -> (path=w955:path)
                n522 = Open/Create/Replace File(file path (use dialog)=w955, operation (0:open)=T18."create", access (0:read/write)=enum16{"read/write", "read-only", "write-only"}."write-only") -> (refnum out=w951:refnum<file>, error out=w952:errorcluster)  [unwired: 3 in, 1 out]
                n523 = Deny Access(4:w952, 7:w951) -> (3:w950:refnum<file>)  [unwired: 1 in, 1 out]
                n524 = Write to Binary File(file (use dialog)=w950, data=w945, 5:FALSE ("prepend array or string size? (T)"), 9:T19."big-endian, network order" ("byte order (0:big-endian, network order)")) -> (refnum out=w942:refnum<file>)  [unwired: 2 in, 2 out]
              }
            }
            n525 = Deny Access(4:w899, 7:w898) -> (0:w889:errorcluster, 3:w897:refnum<file>)  [unwired: 1 in]
            n526 = String Length(string="Comment") -> (length=w904:i32)
            n527 = To Double Precision Float(number=w907) -> (double precision float=w906:dbl)
            n528 = To Double Precision Float(number=w904) -> (double precision float=w903:dbl)
            n529 = Build Array (concatenate)(w906, w905, w903) -> (w894:dbl[])
            n530 = Write to Binary File(file (use dialog)=w897, data=w894, error in=w889, 5:w890, 9:w891) -> (refnum out=w893:refnum<file>, error out=w888:errorcluster)  [unwired: 1 in, 1 out]
            n531 = Write to Binary File(file (use dialog)=w893, data="Comment", error in=w888, 5:w890, 9:w891) -> (refnum out=w883:refnum<file>)  [unwired: 1 in, 2 out]
            "Saving" <- TRUE
          }
        }
        n532 = feedback-in #6(w827) -> ()
        n533 = feedback-in #7(w841) -> ()
        n534 = feedback-in #8(w847) -> ()
        n535 = feedback-in #9(w840) -> ()
        n536 = feedback-in #10(w837) -> ()
        n537 = feedback-in #11(w844) -> ()
      }
      frame #1 {
        n538 = local read "Saving"() -> (w1038:bool)
        n539 = case shown="True" w1038 {
          tunnel: w1047 -> [_ w1067]
          tunnel: w1046 -> [_ w1066]
          tunnel: w1045 -> [_ w1065]
          tunnel: w1044 -> [_ w1064]
          tunnel: w1043 -> [_ w1055]
          tunnel: w1042 -> [_ w1056]
          tunnel: w1041 -> [_ w1059]
          tunnel: w1040 -> [_ w1051]
          tunnel: w1039 -> [_ w1050]
          tunnel: w1037 -> [_ w1048]
          frame False {
            (unwired) FALSE ("Calibrating")
          }
          frame True {
            n540 = local read "Stop"() -> (w1062:bool)
            n541 = Less Or Equal?(x=w1055, y=w1056) -> (x <= y?=w1063:bool)
            n542 = Divide(x=w1055, y=w1056) -> (x/y=w1054:dbl)
            n543 = Or(x=w1062, y="Stop saving") -> (x .or. y?=w1049:bool)
            n544 = Multiply(x=100.0, y=w1054) -> (x*y=w1053:dbl)
            n545 = Not(x=w1049) -> (.not. x?=w1061:bool)
            n546 = And(x=w1063, y=w1061) -> (x .and. y?=w1060:bool)
            n547 = case shown="True" w1060 {
              tunnel: w1065 -> [w1072 w1097]
              tunnel: w1066 -> [_ w1096]
              tunnel: w1067 -> [_ w1095]
              tunnel: w1064 -> [w1071 w1094]
              tunnel: w1059 -> [w1068 _]
              tunnel: [0.0 ("Progress") w1093] -> w1058
              tunnel: w1053 -> [_ w1093]
              tunnel: w1051 -> [_ _]
              tunnel: w1050 -> [_ w1092]
              tunnel: w1048 -> [w1069 w1089]
              frame False {
                n548 = flat-sequence {
                  tunnel: w1072 -> [w1077]
                  tunnel: w1071 -> [w1076]
                  tunnel: w1069 -> [w1075]
                  tunnel: w1068 -> [w1074]
                  frame #0 {
                    n549 = local read "Saving Move"() -> (w1073:bool)
                    n550 = case shown="True" w1074 {
                      tunnel: w1076 -> [_ w1087]
                      frame False {
                      }
                      frame True {
                        n551 = Close File(refnum=w1087) -> ()  [unwired: 1 in, 2 out]
                      }
                    }
                    n552 = case shown="True" w1073 {
                      tunnel: w1075 -> [_ w1082]
                      frame False {
                      }
                      frame True {
                        n553 = Get Date/Time In Seconds() -> (seconds since 1Jan1904=w1086:timestamp)
                        n554 = call <vilib>:"Space Constant.vi"() -> ("String"=w1081:string)
                        n555 = Format Date/Time String(time format string (%c)="%H:%M:%S%3u", seconds (now)=w1086, UTC format=TRUE) -> (date/time string=w1079:string)
                        n556 = Concatenate Strings(w1079, w1081, "end") -> (w1078:string)
                        n557 = Write to Text File(file (use dialog)=w1082, text=w1078) -> (refnum out=w1083:refnum<file>)  [unwired: 2 in, 2 out]
                        n558 = Close File(refnum=w1083) -> ()  [unwired: 1 in, 2 out]
                        n559 = local write "Move time"(w1079) -> ()
                      }
                    }
                    n560 = Close File(refnum=w1077) -> ()  [unwired: 1 in, 2 out]
                  }
                  frame #1 {
                    w1088 = FALSE
                    n561 = local write "Saving"(w1088) -> ()
                    n562 = local write "Stop saving"(w1088) -> ()
                    n563 = local write "Saving Move"(w1088) -> ()
                    n564 = local write "Calibrating"(w1088) -> ()
                    n565 = call <vilib>:"Beep.vi"() -> ()  [unwired: 12 in]
                  }
                }
              }
              frame True {
                n566 = local read "Calibrating"() -> (w1091:bool)
                n567 = local read "Saving Move"() -> (w1090:bool)
                n568 = case shown="True" w1091 {
                  tunnel: w1097 -> [w1130 w1146]
                  tunnel: w1096 -> [_ w1145]
                  tunnel: w1095 -> [w1117 w1139]
                  tunnel: w1094 -> [w1116 _]
                  tunnel: w1092 -> [w1108 _]
                  frame False {
                    n569 = local read "Averaging Number"() -> (w1124:i32)
                    n570 = Array Subset(array=w1117, index (row)=0 ("index"), length (row)=6 ("length")) -> (w1113:dbl[][])  [unwired: 2 in]
                    n571 = Array Subset(array=w1117, index (row)=6 ("index"), length (row)=2 ("length")) -> (w1112:dbl[][])  [unwired: 2 in]
                    n572 = Array Size(array=w1112) -> (size(s)=w1123:i32[])
                    n573 = Array Size(array=w1113) -> (size(s)=w1120:i32[])
                    n574 = Index Array(array=w1108, index=0) -> (element=w1105:waveform(dbl))
                    n575 = Index Array(array=w1108, index=1) -> (element=w1104:waveform(dbl))
                    n576 = for {
                      tunnel: w1113 -> [w1134] mode=indexing
                      tunnel: w1124 -> [w1136]
                      tunnel: [w1135] -> w1111 mode=indexing
                      n577 = call "Downsample 1D array.vi"("Ave N"=w1136, "Arrray In"=w1134) -> ("Array Out"=w1135:dbl[])  [unwired: 9 in]
                    }
                    n578 = Unbundle By Name(w1105) -> ()  [unwired: 1 out]
                    n579 = Unbundle By Name(w1104) -> ()  [unwired: 1 out]
                    n580 = Multiply Array Elements(1:w1120) -> (0:w1119:i32)
                    n581 = for {
                      tunnel: w1112 -> [w1133] mode=indexing
                      tunnel: w1124 -> [w1132]
                      tunnel: [w1131] -> w1115 mode=indexing
                      n582 = call "Downsample 1D array.vi"("Ave N"=w1132, "Arrray In"=w1133) -> ("Array Out"=w1131:dbl[])  [unwired: 9 in]
                    }
                    n583 = Multiply Array Elements(1:w1123) -> (0:w1122:i32)
                    n584 = Divide(x=w1119, y=w1124) -> (x/y=w1125:dbl)
                    n585 = Divide(x=w1122, y=w1124) -> (x/y=w1121:dbl)
                    n586 = Transpose 2D Array(2D array=w1111) -> (transposed array=w1110:dbl[][])
                    n587 = Transpose 2D Array(2D array=w1115) -> (transposed array=w1109:dbl[][])
                    n588 = Reshape Array(w1110, w1125) -> (w1114:dbl[])
                    n589 = Reshape Array(w1109, w1121) -> (w1118:dbl[])
                    n590 = call <vilib>:"Write File+ [SGL].vi"("1D array"=w1118, "refnum"=w1116) -> ()  [unwired: 7 in, 3 out]
                    n591 = call <vilib>:"Write File+ [SGL].vi"("1D array"=w1114, "refnum"=w1130) -> ()  [unwired: 7 in, 3 out]
                  }
                  frame True {
                    n592 = Array Subset(array=w1139, index (row)=0 ("index"), length (row)=6 ("length")) -> (w1137:dbl[][])  [unwired: 2 in]
                    n593 = Transpose 2D Array(2D array=w1137) -> (transposed array=w1143:dbl[][])
                    n594 = Array Size(array=w1137) -> (size(s)=w1138:i32[])
                    n595 = Multiply Array Elements(1:w1138) -> (0:w1144:i32)
                    n596 = Reshape Array(w1143, w1144) -> (w1142:dbl[])
                    n597 = call <vilib>:"Write File+ [SGL].vi"("1D array"=w1142, "error in (no error)"=w1145, "refnum"=w1146) -> ()  [unwired: 6 in, 3 out]
                  }
                }
                n598 = case shown="True" w1090 {
                  tunnel: w1089 -> [_ w1098]
                  frame False {
                  }
                  frame True {
                    n599 = event shown="[0] \"Move time\": Value Change" {
                      selector: _ -> [_ _]
                      dyn-events: _ -> [_ _]
                      timeout: 1 -> [_ _]
                      tunnel: w1098 -> [w1103 _]
                      event "Move time": Value Change {
                        n600 = event-data() -> ("NewVal"=w1102:string)  [unwired: 1 in, 5 out]
                        n601 = Concatenate Strings(w1102, "\r\n") -> (w1100:string)
                        n602 = Write to Text File(file (use dialog)=w1103, text=w1100) -> ()  [unwired: 2 in, 3 out]
                      }
                      event Timeout {
                        n603 = event-data() -> ()  [unwired: 1 in, 3 out]
                      }
                    }
                  }
                }
              }
            }
            "Progress" <- w1058
          }
        }
      }
    }
    n604 = Square Root(x=w438) -> (sqrt(x)=→"Force noise (pN)":dbl)
    n605 = local read "Flushing Sample"() -> (w370:bool)
    n606 = case shown="True" w370 {
      frame False {
      }
      frame True {
        n607 = local read "Flush Sample Start Time"() -> (w781:u32)
        n608 = local read "Sample flush time (s)"() -> (w774:dbl)
        n609 = Tick Count (ms)() -> (millisecond timer value=w782:u32)
        n610 = Subtract(x=w782, y=w781) -> (x-y=w772:u32)
        n611 = Multiply(x=u32 1000, y=w774) -> (x*y=w773:dbl)
        n612 = Divide(x=w772, y=w773) -> (x/y=w777:dbl)
        n613 = Greater?(x=w772, y=w773) -> (0:w780:bool)
        n614 = Not(x=w780) -> (.not. x?=w779:bool)
        n615 = Boolean To (0,1)(Boolean=w779) -> (0, 1=w778:i16)
        n616 = Compound Arithmetic op=MULTIPLY(w778, w777, 100.0 ("value")) -> (→"Sample Flush Meter":dbl)
        n617 = case shown="True" w780 {
          frame False {
          }
          frame True {
            w784 = FALSE ("Inject Sample")
            n618 = property on="Clear Volume" class="Bool (strict)"("Val(Sgnl)"=TRUE ("Value (Signaling)")) -> ()  [unwired: 2 in, 2 out]
            n619 = local write "Inject Sample"(w784) -> ()
            n620 = local write "Flushing Sample"(w784) -> ()
          }
        }
      }
    }
    n621 = feedback #12(0) -> (w354:i32)
    n622 = feedback #13(0) -> (w351:i32)
    n623 = feedback #14(0) -> (w356:i32)
    n624 = case shown="True" w361 {
      tunnel: w365 -> [w673 w731]
      tunnel: [w673 w715] -> w364
      tunnel: w363 -> [w672 w730]
      tunnel: [w672 w714] -> w362
      tunnel: "Raster scan" -> [w671 w708]
      tunnel: [w671 w707] -> w359
      tunnel: [0 w706] -> w357
      tunnel: w356 -> [_ w700]
      tunnel: w354 -> [_ w688]
      tunnel: [0 w691] -> w353
      tunnel: w351 -> [_ w697]
      tunnel: [0 w696] -> w350
      frame False {
      }
      frame True {
        # "Reset step counter"
        # "Current position"
        # "Initial values"
        n625 = local read "Conv Y (nm/V)"() -> (w683:dbl)
        n626 = local read "Conv X (nm/V)"() -> (w684:dbl)
        n627 = local read "Trap delta (nm)"() -> (w682:dbl)
        n628 = disable-structure shown="Disabled" {
          frame Disabled {
            n629 = local write "Raster scan"(FALSE ("Raster scan")) -> ()
            n630 = property on="Reset data stream" class="Bool (strict)"("Val(Sgnl)"=TRUE) -> ()  [unwired: 2 in, 2 out]
          }
          frame Enabled {
          }
        }
        n631 = local read "Data update period (s/set)"() -> (w705:dbl)
        n632 = local read "Time per step (ms)"() -> (w702:dbl)
        n633 = Select(t=w683, s="Pulling direction", f=w684) -> (s? t:f=w681:dbl)
        n634 = Divide(x=w682, y=w681) -> (x/y=w680:dbl)
        n635 = local read "Fixed X"() -> (w724:dbl)
        n636 = local read "Fixed Y"() -> (w725:dbl)
        n637 = local read "Fixed X"() -> (w686:dbl)
        n638 = local read "Fixed Y"() -> (w685:dbl)
        n639 = local read "Trap position (V)"() -> (w687:cluster{"X":dbl, "Y":dbl})
        n640 = Select(t=w685, s="Pulling direction", f=w686) -> (s? t:f=w679:dbl)
        n641 = local read "Scan steps (mirror)"() -> (w713:u64)
        n642 = Unbundle(w687) -> ("X"=w677:dbl, "Y"=w678:dbl)
        n643 = Multiply(x=w705, y=1000.0) -> (x*y=w703:dbl)
        n644 = local read "Stop raster"() -> (w720:bool)
        n645 = local read "Stop saving"() -> (w721:bool)
        n646 = Select(t=w724, s="Pulling direction", f=w725) -> (s? t:f=w732:dbl)
        n647 = Add(x=w680, y=w679) -> ()  [unwired: 1 out]
        n648 = local write "Saving Move"(FALSE) -> ()
        n649 = Divide(x=w702, y=w703) -> (x/y=w701:dbl)
        n650 = Quotient & Remainder(x=w700, y=w701) -> (x-y*floor(x/y)=w699:dbl)  [unwired: 1 out]
        n651 = Not(x=w720) -> (.not. x?=w719:bool)
        n652 = Select(t=w678, s="Pulling direction", f=w677) -> (s? t:f=w675:dbl)
        n653 = Not(x=w721) -> (.not. x?=w718:bool)
        n654 = Multiply(x=u64 2, y=w713) -> (x*y=w709:u64)
        n655 = Equal To 0?(x=w699) -> (x = 0?=w698:bool)
        n656 = Less?(x=w688, y=w709) -> (x < y?=w710:bool)
        n657 = Compound Arithmetic op=AND(w710, w719, w718, w698) -> (w711:bool)
        n658 = Not(x=w710) -> (.not. x?=w694:bool)
        n659 = feedback #15() -> (w716:dbl)  [unwired: 1 in]
        n660 = case shown="True" w711 {
          tunnel: w732 -> [_ w767]
          tunnel: w675 -> [_ w749]
          tunnel: w731 -> [w744 w766]
          tunnel: w730 -> [w743 w765]
          tunnel: [w744 w764] -> w715
          tunnel: [w743 w763] -> w714
          tunnel: [w740 w752] -> w717
          tunnel: w688 -> [w741 w747]
          tunnel: w716 -> [w740 w746]
          tunnel: w708 -> [w742 w751]
          tunnel: [w742 w751] -> w707
          tunnel: [w741 w750] -> w692
          frame False {
          }
          frame True {
            # "Go forward or backward?"
            n661 = local read "Scan increment (V)"() -> (w745:dbl)
            n662 = local read "Scan steps (mirror)"() -> (w756:u64)
            n663 = Multiply(x=w745, y=w747) -> (x*y=w748:dbl)
            n664 = Less?(x=w747, y=w756) -> (x < y?=w755:bool)
            n665 = Add(x=w749, y=w748) -> (x+y=w758:dbl)
            n666 = Subtract(x=w746, y=w745) -> (x-y=w757:dbl)
            n667 = Select(t=w758, s=w755, f=w757) -> (s? t:f=w752:dbl)
            n668 = local read "Pulling direction"() -> (w754:bool)
            n669 = Build Array(w752, w767) -> (w761:dbl[])
            n670 = Build Array(w767, w752) -> (w760:dbl[])
            n671 = Select(t=w761, s=w754, f=w760) -> (s? t:f=w759:dbl[])
            n672 = call-poly <vilib>:"DAQmx Write.vi"("task/channels in"=w766, "auto start"=TRUE, "data"=w759, "error in"=w765) -> ("task out"=w764:refnum<k21>, "error out"=w763:errorcluster)  [unwired: 9 in, 1 out]
            n673 = Increment(x=w747) -> (x+1=w750:i32)
            "Raster scanning..." <- TRUE ("Raster scanning...")
          }
        }
        n674 = feedback-in #15(w717) -> ()
        n675 = case shown="True" w694 {
          tunnel: w697 -> [w737 w739]
          tunnel: [w737 w738] -> w696
          frame False {
          }
          frame True {
            n676 = Increment(x=w739) -> (x+1=w738:i32)
          }
        }
        n677 = local read "# scans"() -> (w695:i32)
        n678 = local read "Stop saving"() -> (w723:bool)
        n679 = Greater Or Equal?(x=w696, y=w695) -> (x >= y?=w689:bool)
        n680 = Not(x=w689) -> (.not. x?=w690:bool)
        n681 = And(x=w694, y=w690) -> (x .and. y?=w693:bool)
        n682 = Compound Arithmetic op=OR(w689, "Stop raster", w723) -> (w726:bool)
        n683 = case shown="True" w726 {
          frame False {
          }
          frame True {
            n684 = flat-sequence {
              frame #0 {
                n685 = Wait (ms)(milliseconds to wait=u32 300) -> ()  [unwired: 1 out]
              }
              frame #1 {
                n686 = property on="Trap delta (nm)" class="DigNum (strict)"("Val(Sgnl)"="Trap delta\nafter (nm)") -> ()  [unwired: 2 in, 2 out]
              }
            }
          }
        }
        n687 = And(x="Flow on\nafter raster?", y=w726) -> (x .and. y?=w727:bool)
        n688 = case shown="True" w727 {
          frame False {
          }
          frame True {
            n689 = property on="Inject Sample" class="Bool (strict)"("Val(Sgnl)"=TRUE ("Value (Signaling)")) -> ()  [unwired: 2 in, 2 out]
          }
        }
        n690 = case shown="True" w693 {
          tunnel: w692 -> [w735 _]
          tunnel: [w735 0] -> w691
          frame False {
          }
          frame True {
          }
        }
        n691 = Not(x=w726) -> (.not. x?=w729:bool)
        n692 = local write "Raster scanning..."(w729) -> ()
        n693 = Increment(x=w700) -> (x+1=w706:i32)
      }
    }
    n694 = And(x="Save scans", y=w359) -> (x .and. y?=w368:bool)
    n695 = feedback-in #12(w353) -> ()
    n696 = feedback-in #13(w350) -> ()
    n697 = feedback-in #14(w357) -> ()
    n698 = local read "Stop"() -> (w646:bool)
  }
  n699 = local write "Progress"(u8 0 ("Progress")) -> ()
  n700 = local write "Calibrating"(FALSE ("Calibrating")) -> ()
  n701 = VISA Open(VISA resource name="USB port") -> (VISA resource name=w12:refnum<visa-resource-name>, error out=w11:errorcluster)  [unwired: 1 in, 3 out]
  n702 = VISA Enable Event(8:w11, 10:w10, 11:w12) -> (0:w7:errorcluster, 3:w8:refnum<visa-resource-name>)  [unwired: 1 out]
  n703 = call-poly "VISA Configure Serial Port"("VISA resource name"=refnum<visa-resource-name> "COM5", "baud rate (9600)"=u32 19200) -> ("VISA resource name out"=w2:refnum<visa-resource-name>, "error out"=w28:errorcluster)  [unwired: 12 in]
  n704 = while {
    tunnel: w2 -> [w1230]
    shift-right: [w1226] -> w4
    shift-left: w8 -> [w1229]
    shift-right: [w1227] -> w3
    shift-left: w7 -> [w1228]
    stop <- w1225 stop-if-true
    n705 = global read "FAST_Global_var.vi" "FAST L"() -> (→"FAST Z" →"FAST Z":bool)
    n706 = global read "FAST_Global_var.vi" "FAST R"() -> (→"FAST X-Y" →"FAST X-Y":bool)
    n707 = call "LogitechSubVi.vi"("USB port"=w1229, "VISA resource name in 2 (for the Newport)"=w1230, "error in (no error)"=w1228, "X-Y Wait time"="X-Y Wait time", "Z Wait time"="Z Wait time", "XY Speed Definitions"="XY Speed Definitions", "Z Speed Definitions"="Z Speed Definitions") -> ("Right stick button"=→"Right stick button":bool, "Left stick button"=→"Left stick button":bool, "USB port out"=w1226:refnum<visa-resource-name>, "error out"=w1227:errorcluster, "A B X Y"=w1219:cluster{"A":bool, "B":bool, "X":bool, "Y":bool}, "LB RB"=w1218:T21, "U D L R"=w1224:cluster{"U":bool, "D":bool, "L":bool, "R":bool}, "Sticks"=w1217:T22)  [unwired: 5 in]
    n708 = Unbundle By Name(w1218) -> ("LB"=w1212:bool, "RB"=w1211:bool, "BACK"=w1185:bool, "Logitech"=w1184:bool, "START"=w1186:bool)
    "RB" <- w1211
    "LB" <- w1212
    "BACK" <- w1185
    "START" <- w1186
    "Logitech" <- w1184
    n709 = case shown="True" w1186 {
      selector: w1186 -> [_ w1234]
      frame False {
      }
      frame True {
        n710 = property on="Move to Position 2" class="Bool (strict)"("Val(Sgnl)"=w1234) -> ()  [unwired: 2 in, 2 out]
      }
    }
    n711 = case shown="True" w1184 {
      frame False {
      }
      frame True {
        n712 = local read "Inject Sample"() -> (w1231:bool)
        n713 = Not(x=w1231) -> (.not. x?=w1232:bool)
        n714 = property on="Inject Sample" class="Bool (strict)"("Val(Sgnl)"=w1232) -> ()  [unwired: 2 in, 2 out]
      }
    }
    n715 = case shown="True" w1212 {
      frame False {
      }
      frame True {
        n716 = local read "Shutter 1 (B)"() -> (w1278:bool)
        n717 = Not(x=w1278) -> (.not. x?=w1277:bool)
        n718 = property on="Shutter 1 (B)" class="Bool (strict)"("Val(Sgnl)"=w1277) -> ()  [unwired: 2 in, 2 out]
      }
    }
    n719 = case shown="True" w1185 {
      selector: w1185 -> [_ w1233]
      frame False {
      }
      frame True {
        n720 = property on="Move to Position 1" class="Bool (strict)"("Val(Sgnl)"=w1233) -> ()  [unwired: 2 in, 2 out]
      }
    }
    n721 = Unbundle By Name(w1224) -> ("U"=→"U":bool, "D"=→"D":bool, "L"=→"L":bool, "R"=→"R":bool)
    n722 = Unbundle By Name(w1219) -> ("A"=w1207:bool, "B"=w1205:bool, "X"=w1210:bool, "Y"=w1203:bool)
    "A" <- w1207
    "B" <- w1205
    "X" <- w1210
    "Y" <- w1203
    n723 = case shown="\"Fish\"" "A command" {
      tunnel: w1207 -> [w1257 w1259 w1261 w1264]
      frame "Got ADig", Default {
        n724 = case shown="True" w1257 {
          selector: w1257 -> [_ w1258]
          frame False {
          }
          frame True {
            n725 = property on="Got ADig bead" class="Bool (strict)"("Val(Sgnl)"=w1258) -> ()  [unwired: 2 in, 2 out]
          }
        }
      }
      frame "Dump" {
        n726 = case shown="True" w1259 {
          selector: w1259 -> [_ w1260]
          frame False {
          }
          frame True {
            n727 = property on="Dump beads" class="Bool (strict)"("Val(Sgnl)"=w1260) -> ()  [unwired: 2 in, 2 out]
          }
        }
      }
      frame "Fish" {
        n728 = case shown="True" w1261 {
          frame False {
          }
          frame True {
            n729 = local read "Fish"() -> (w1262:bool)
            n730 = Not(x=w1262) -> (.not. x?=w1263:bool)
            n731 = property on="Fish" class="Bool (strict)"("Val(Sgnl)"=w1263) -> ()  [unwired: 2 in, 2 out]
          }
        }
      }
      frame "Got DNA" {
        n732 = case shown="True" w1264 {
          selector: w1264 -> [_ w1265]
          frame False {
          }
          frame True {
            n733 = property on="Got DNA bead" class="Bool (strict)"("Val(Sgnl)"=w1265) -> ()  [unwired: 2 in, 2 out]
          }
        }
      }
    }
    n734 = case shown="True" w1211 {
      frame False {
      }
      frame True {
        n735 = local read "Shutter 2 (A)"() -> (w1276:bool)
        n736 = Not(x=w1276) -> (.not. x?=w1275:bool)
        n737 = property on="Shutter 2 (A)" class="Bool (strict)"("Val(Sgnl)"=w1275) -> ()  [unwired: 2 in, 2 out]
      }
    }
    n738 = Unbundle By Name(w1217) -> ("Right X"=w1189:i8, "Right Y"=w1191:i8, "Left X"=w1193:i8, "Left Y"=w1198:i8)
    n739 = Not Equal?(x=w1198, y=i8 0) -> (x != y?=w1199:bool)
    n740 = case shown="True" w1199 {
      tunnel: w1198 -> [_ w1238]
      frame False {
      }
      frame True {
        "Left Y" <- w1238
      }
    }
    n741 = case shown="\"Got DNA\", Default" "B command" {
      tunnel: w1205 -> [w1248 w1250 w1252 w1254]
      frame "Got DNA", Default {
        n742 = case shown="True" w1248 {
          selector: w1248 -> [_ w1249]
          frame False {
          }
          frame True {
            n743 = property on="Got DNA bead" class="Bool (strict)"("Val(Sgnl)"=w1249) -> ()  [unwired: 2 in, 2 out]
          }
        }
      }
      frame "Got ADig" {
        n744 = case shown="True" w1250 {
          selector: w1250 -> [_ w1251]
          frame False {
          }
          frame True {
            n745 = property on="Got ADig bead" class="Bool (strict)"("Val(Sgnl)"=w1251) -> ()  [unwired: 2 in, 2 out]
          }
        }
      }
      frame "Dump" {
        n746 = case shown="True" w1252 {
          selector: w1252 -> [_ w1253]
          frame False {
          }
          frame True {
            n747 = property on="Dump beads" class="Bool (strict)"("Val(Sgnl)"=w1253) -> ()  [unwired: 2 in, 2 out]
          }
        }
      }
      frame "Fish" {
        n748 = case shown="True" w1254 {
          frame False {
          }
          frame True {
            n749 = local read "Fish"() -> (w1255:bool)
            n750 = Not(x=w1255) -> (.not. x?=w1256:bool)
            n751 = property on="Fish" class="Bool (strict)"("Val(Sgnl)"=w1256) -> ()  [unwired: 2 in, 2 out]
          }
        }
      }
    }
    n752 = Not Equal?(x=w1189, y=i8 0) -> (x != y?=w1190:bool)
    n753 = Not Equal?(x=w1191, y=i8 0) -> (x != y?=w1192:bool)
    n754 = Not Equal?(x=w1193, y=i8 0) -> (x != y?=w1194:bool)
    n755 = case shown="True" w1194 {
      tunnel: w1193 -> [_ w1237]
      frame False {
      }
      frame True {
        "Left X" <- w1237
      }
    }
    n756 = case shown="False" w1190 {
      tunnel: w1189 -> [_ w1235]
      frame False {
      }
      frame True {
        "Right X" <- w1235
      }
    }
    n757 = case shown="False" w1192 {
      tunnel: w1191 -> [_ w1236]
      frame False {
      }
      frame True {
        "Right Y" <- w1236
      }
    }
    n758 = case shown="\"Dump\", Default" "X command" {
      tunnel: w1210 -> [w1266 w1268 w1271 w1273]
      frame "Dump", Default {
        n759 = case shown="True" w1266 {
          selector: w1266 -> [_ w1267]
          frame False {
          }
          frame True {
            n760 = property on="Dump beads" class="Bool (strict)"("Val(Sgnl)"=w1267) -> ()  [unwired: 2 in, 2 out]
          }
        }
      }
      frame "Fish" {
        n761 = case shown="True" w1268 {
          frame False {
          }
          frame True {
            n762 = local read "Fish"() -> (w1270:bool)
            n763 = Not(x=w1270) -> (.not. x?=w1269:bool)
            n764 = property on="Fish" class="Bool (strict)"("Val(Sgnl)"=w1269) -> ()  [unwired: 2 in, 2 out]
          }
        }
      }
      frame "Got ADig" {
        n765 = case shown="True" w1271 {
          selector: w1271 -> [_ w1272]
          frame False {
          }
          frame True {
            n766 = property on="Got ADig bead" class="Bool (strict)"("Val(Sgnl)"=w1272) -> ()  [unwired: 2 in, 2 out]
          }
        }
      }
      frame "Got DNA" {
        n767 = case shown="True" w1273 {
          selector: w1273 -> [_ w1274]
          frame False {
          }
          frame True {
            n768 = property on="Got DNA bead" class="Bool (strict)"("Val(Sgnl)"=w1274) -> ()  [unwired: 2 in, 2 out]
          }
        }
      }
    }
    n769 = case shown="\"Fish\", Default" "Y command" {
      tunnel: w1203 -> [w1239 w1242 w1244 w1246]
      frame "Fish", Default {
        n770 = case shown="True" w1239 {
          frame False {
          }
          frame True {
            n771 = local read "Fish"() -> (w1240:bool)
            n772 = Not(x=w1240) -> (.not. x?=w1241:bool)
            n773 = property on="Fish" class="Bool (strict)"("Val(Sgnl)"=w1241) -> ()  [unwired: 2 in, 2 out]
          }
        }
      }
      frame "Dump" {
        n774 = case shown="True" w1242 {
          selector: w1242 -> [_ w1243]
          frame False {
          }
          frame True {
            n775 = property on="Dump beads" class="Bool (strict)"("Val(Sgnl)"=w1243) -> ()  [unwired: 2 in, 2 out]
          }
        }
      }
      frame "Got ADig" {
        n776 = case shown="True" w1244 {
          selector: w1244 -> [_ w1245]
          frame False {
          }
          frame True {
            n777 = property on="Got ADig bead" class="Bool (strict)"("Val(Sgnl)"=w1245) -> ()  [unwired: 2 in, 2 out]
          }
        }
      }
      frame "Got DNA" {
        n778 = case shown="True" w1246 {
          selector: w1246 -> [_ w1247]
          frame False {
          }
          frame True {
            n779 = property on="Got DNA bead" class="Bool (strict)"("Val(Sgnl)"=w1247) -> ()  [unwired: 2 in, 2 out]
          }
        }
      }
    }
    n780 = local read "Stop"() -> (w1225:bool)
  }
  n781 = VISA Close(VISA resource name=w4, error in (no error)=w3) -> (error out=w5:errorcluster)
  n782 = call <vilib>:"Simple Error Handler.vi"("error in (no error)"=w5) -> ()  [unwired: 1 in, 8 out]
  n783 = node-c288(i64 100 ("Period"), 2 ("Processor")) -> (w30:T13)  [unwired: 2 in]
  n784 = timed-loop {
    timing: w30 -> [_]
    timing-out: [_] -> w29
    tunnel: w2 -> [w1279]
    tunnel: w28 -> [w1281]
    tunnel: [w1279] -> w27
    stop <- w1280 stop-if-true
    n785 = node-c288() -> ()  [unwired: 1 in, 1 out]
    n786 = event shown="[1] \"Dump beads\": Value Change" {
      selector: _ -> [_ _ _ _ _ _ _ _ _ _ _ _ _ _ _]
      dyn-events: _ -> [_ _ _ _ _ _ _ _ _ _ _ _ _ _ _]
      timeout: _ -> [_ _ _ _ _ _ _ _ _ _ _ _ _ _ _]
      tunnel: w1279 -> [w1288 w1340 w1360 w1378 w1395 w1416 w1464 w1479 w1554 _ _ _ _ _ _]
      tunnel: w1281 -> [w1287 w1339 w1359 w1377 w1394 w1415 w1463 w1478 w1552 _ _ _ _ _ _]
      tunnel: [_ _ _ _ _ _ _ _ _ _ _ _ _ _ w1736] -> w1280
      event "Got DNA bead": Value Change {
        n787 = event-data() -> ()  [unwired: 1 in, 5 out]
        n788 = flat-sequence {
          tunnel: w1287 -> [w1291]
          tunnel: ["Cal @ Delta (nm)"] -> w1283
          tunnel: w1288 -> [w1293]
          tunnel: [w1307] -> w1286
          tunnel: w1283 -> [w1306]
          tunnel: w1286 -> [w1328]
          tunnel: [w1328] -> w1285
          tunnel: w1285 -> [w1330]
          tunnel: [w1330] -> w1284
          tunnel: w1284 -> [w1332]
          frame #0 {
            n789 = local read "Saved stage positions"() -> (w1294:dbl[][])
            n790 = property on="Inject Sample" class="Bool (strict)"("Val(Sgnl)"=TRUE ("Value (Signaling)")) -> ()  [unwired: 2 in, 2 out]
            n791 = disable-structure shown="Disabled" {
              frame Disabled {
                n792 = property on="Inject Pump 2" class="Bool (strict)"("Val(Sgnl)"=FALSE ("Inject Pump 2")) -> ()  [unwired: 2 in, 2 out]
              }
              frame Enabled {
              }
            }
            n793 = local write "Stage moving"(TRUE ("Stage moving")) -> ()
            n794 = property on="Trap delta (nm)" class="DigNum (strict)"("Val(Sgnl)"="Cal @ Delta (nm)") -> ()  [unwired: 2 in, 2 out]
            n795 = call "move to saved stage position.vi"("error in"=w1291, "Stage VISA resource name in"=w1293, "Position"="Cal stage position", "Saved Stage Positions"=w1294) -> ()  [unwired: 2 out]
          }
          frame #1 {
            n796 = local write "Stage moving"(FALSE ("Stage moving")) -> ()
            n797 = property on="Inject Sample" class="Bool (strict)"("Val(Sgnl)"=FALSE ("Value (Signaling)")) -> ()  [unwired: 2 in, 2 out]
            n798 = call <vilib>:"Beep.vi"() -> ()  [unwired: 12 in]
          }
          frame #2 {
            # "increased from 1000 to 5000 v6.4. \nMar.7,2018."
            n799 = Wait (ms)(milliseconds to wait=u32 5000) -> ()  [unwired: 1 out]
          }
          frame #3 {
            n800 = property on="Save cal" class="Bool (strict)"("Val(Sgnl)"=TRUE ("Value (Signaling)")) -> ()  [unwired: 2 in, 2 out]
          }
          frame #4 {
            n801 = Wait (ms)(milliseconds to wait=u32 2000) -> ()  [unwired: 1 out]
          }
          frame #5 {
            n802 = while {
              stop <- w1303 stop-if-true
              n803 = local read "Saving"() -> (w1304:bool)
              n804 = Not(x=w1304) -> (.not. x?=w1303:bool)
              n805 = Wait (ms)(milliseconds to wait=u32 100) -> ()  [unwired: 1 out]
            }
          }
          frame #6 {
            n806 = Wait (ms)(milliseconds to wait=u32 2000) -> ()  [unwired: 1 out]
          }
          frame #7 {
            n807 = stacked-sequence {
              tunnel: [_ _ _ _ _ _ w1322 _] -> w1307
              tunnel: w1306 -> [_ _ _ _ _ _ _ w1327]
              frame #0 {
                n808 = property on="Trap delta (nm)" class="DigNum (strict)"("Val(Sgnl)"="Offset @ Delta (nm)") -> ()  [unwired: 2 in, 2 out]
                n809 = Replace Array Subset(array=i32[] [0], new element="Offset raster set", index=0) -> (w1311:i32[])
                n810 = property on="Scan Parameters" class="Arr (strict)"("Index Values"=w1311) -> ()  [unwired: 2 in, 2 out]
              }
              frame #1 {
                n811 = Wait (ms)(milliseconds to wait=u32 200) -> ()  [unwired: 1 out]
              }
              frame #2 {
                n812 = property on="Load param" class="Bool (strict)"("Val(Sgnl)"=TRUE ("Load param")) -> ()  [unwired: 2 in, 2 out]
              }
              frame #3 {
                n813 = Wait (ms)(milliseconds to wait=u32 200) -> ()  [unwired: 1 out]
              }
              frame #4 {
                # "Only continue if there is no buffer\noverflow error"
                n814 = local read "Buffer Overflow"() -> (w1317:bool)
                n815 = Not(x=w1317) -> (.not. x?=w1316:bool)
                n816 = case shown="True" w1316 {
                  frame False {
                  }
                  frame True {
                    n817 = property on="Raster scan" class="Bool (strict)"("Val(Sgnl)"=TRUE ("Value (Signaling)")) -> ()  [unwired: 2 in, 2 out]
                  }
                }
              }
              frame #5 {
                n818 = local read "Buffer Overflow"() -> (w1320:bool)
                n819 = Not(x=w1320) -> (.not. x?=w1319:bool)
                n820 = case shown="True" w1319 {
                  frame False {
                  }
                  frame True {
                    n821 = Wait (ms)(milliseconds to wait=u32 2000) -> ()  [unwired: 1 out]
                  }
                }
              }
              frame #6 {
                n822 = local read "Buffer Overflow"() -> (w1323:bool)
                n823 = Not(x=w1323) -> (.not. x?=w1322:bool)
                n824 = case shown="True" w1322 {
                  frame False {
                  }
                  frame True {
                    n825 = while {
                      stop <- w1325 stop-if-true
                      n826 = local read "Saving"() -> (w1326:bool)
                      n827 = Not(x=w1326) -> (.not. x?=w1325:bool)
                      n828 = Wait (ms)(milliseconds to wait=u32 100) -> ()  [unwired: 1 out]
                    }
                  }
                }
              }
              frame #7 {
                n829 = property on="Trap delta (nm)" class="DigNum (strict)"("Val(Sgnl)"=w1327) -> ()  [unwired: 2 in, 2 out]
              }
            }
          }
          frame #8 {
            n830 = case shown="True" w1328 {
              frame False {
              }
              frame True {
                n831 = property on="Read Cal" class="Bool (strict)"("Val(Sgnl)"=TRUE ("Value (Signaling)")) -> ()  [unwired: 2 in, 2 out]
              }
            }
          }
          frame #9 {
            n832 = case shown="True" w1330 {
              frame False {
              }
              frame True {
                n833 = Wait (ms)(milliseconds to wait=u32 1000) -> ()  [unwired: 1 out]
              }
            }
          }
          frame #10 {
            n834 = case shown="True" w1332 {
              frame False {
              }
              frame True {
                n835 = property on="Fish" class="Bool (strict)"("Val(Sgnl)"=TRUE ("Value (Signaling)")) -> ()  [unwired: 2 in, 2 out]
                n836 = case shown="False" "Flow on\nwhile fish?" {
                  frame False {
                    n837 = property on="Inject Sample" class="Bool (strict)"("Val(Sgnl)"=FALSE) -> ()  [unwired: 2 in, 2 out]
                  }
                  frame True {
                    n838 = property on="Inject Sample" class="Bool (strict)"("Val(Sgnl)"=TRUE ("Value (Signaling)")) -> ()  [unwired: 2 in, 2 out]
                  }
                }
              }
            }
          }
        }
        n839 = local write "Got DNA bead"(FALSE) -> ()
      }
      event "Dump beads": Value Change {
        n840 = event-data() -> ()  [unwired: 1 in, 5 out]
        n841 = flat-sequence {
          tunnel: w1339 -> [w1343]
          tunnel: w1340 -> [w1344]
          tunnel: [w1344] -> w1338
          tunnel: [w1343] -> w1337
          tunnel: w1338 -> [w1347]
          tunnel: w1337 -> [w1346]
          frame #0 {
            w1341 = FALSE ("Fish")
            n842 = local read "Saving"() -> (w1342:bool)
            n843 = local write "Force Feedback 2"(w1341) -> ()
            n844 = local write "Pause dwell"(w1341) -> ()
            n845 = local write "Force Feedback 1"(w1341) -> ()
            n846 = local write "Dump beads"(w1341) -> ()
            n847 = property on="Stop saving" class="Bool (strict)"("Val(Sgnl)"=w1342) -> ()  [unwired: 2 in, 2 out]
            n848 = local write "Fish"(w1341) -> ()
          }
          frame #1 {
            n849 = local read "Saved stage positions"() -> (w1349:dbl[][])
            n850 = case shown="True" "Flow on\ndump?" {
              frame False {
              }
              frame True {
                n851 = property on="Inject Sample" class="Bool (strict)"("Val(Sgnl)"=TRUE ("Value (Signaling)")) -> ()  [unwired: 2 in, 2 out]
              }
            }
            n852 = local write "Stage moving"(TRUE ("Stage moving")) -> ()
            n853 = call "move to saved stage position.vi"("error in"=w1346, "Stage VISA resource name in"=w1347, "Position"=5, "Saved Stage Positions"=w1349) -> ()  [unwired: 2 out]
          }
          frame #2 {
            n854 = local read "Shutter 1 (B)"() -> (w1354:bool)
            n855 = local read "Shutter 2 (A)"() -> (w1353:bool)
            n856 = call <vilib>:"Beep.vi"() -> ()  [unwired: 12 in]
            n857 = case shown="True" w1354 {
              frame False {
              }
              frame True {
                n858 = property on="Shutter 1 (B)" class="Bool (strict)"("Val(Sgnl)"=FALSE ("Value (Signaling)")) -> ()  [unwired: 2 in, 2 out]
              }
            }
            n859 = case shown="True" w1353 {
              frame False {
              }
              frame True {
                n860 = property on="Shutter 2 (A)" class="Bool (strict)"("Val(Sgnl)"=FALSE) -> ()  [unwired: 2 in, 2 out]
              }
            }
            n861 = local write "Stage moving"(FALSE ("Stage moving")) -> ()
            n862 = local write "Tether"(FALSE ("Tether")) -> ()
          }
          frame #3 {
            n863 = property on="Move Cap. 2 (ADig Top)" class="Bool (strict)"("Val(Sgnl)"=TRUE ("Value (Signaling)")) -> ()  [unwired: 2 in, 2 out]
          }
        }
      }
      event "Move Cap. 2 (ADig Top)": Value Change {
        n864 = event-data() -> ()  [unwired: 1 in, 5 out]
        n865 = flat-sequence {
          tunnel: w1360 -> [w1364]
          tunnel: w1359 -> [w1363]
          frame #0 {
            n866 = local read "Saved stage positions"() -> (w1362:dbl[][])
            n867 = case shown="True" "Flow on\ncap 2?" {
              frame False {
              }
              frame True {
                n868 = property on="Inject Sample" class="Bool (strict)"("Val(Sgnl)"=TRUE ("Value (Signaling)")) -> ()  [unwired: 2 in, 2 out]
              }
            }
            n869 = local write "Move Cap. 2 (ADig Top)"(FALSE ("Move Cap. 2 (ADig Top)")) -> ()
            n870 = local write "Stage moving"(TRUE ("Stage moving")) -> ()
            n871 = call "move to saved stage position.vi"("error in"=w1363, "Stage VISA resource name in"=w1364, "Position"=2, "Saved Stage Positions"=w1362) -> ()  [unwired: 2 out]
          }
          frame #1 {
            # "Make sure you don't reverse\nwhich is ON and OFF"
            n872 = local read "Cal @ Delta (nm)"() -> (w1372:dbl)
            n873 = local write "Stage moving"(FALSE ("Stage moving")) -> ()
            n874 = call <vilib>:"Beep.vi"() -> ()  [unwired: 12 in]
            n875 = property on="Trap delta (nm)" class="DigNum (strict)"("Val(Sgnl)"=w1372) -> ()  [unwired: 2 in, 2 out]
            n876 = property class="TabCtl (strict)"("Val(Sgnl)"=T4."Status" ("Value (Signaling)")) -> ()  [unwired: 2 in, 2 out]
            n877 = disable-structure shown="Disabled" {
              frame Disabled {
                n878 = property on="Inject Pump 1" class="Bool (strict)"("Val(Sgnl)"=TRUE ("Inject Pump 2")) -> ()  [unwired: 2 in, 2 out]
              }
              frame Enabled {
              }
            }
            n879 = local read "Shutter 2 (A)"() -> (w1371:bool)
            n880 = case shown="False" w1371 {
              frame False {
                n881 = property on="Shutter 2 (A)" class="Bool (strict)"("Val(Sgnl)"=TRUE ("Value (Signaling)")) -> ()  [unwired: 2 in, 2 out]
              }
              frame True {
              }
            }
            n882 = property on="Inject Sample" class="Bool (strict)"("Val(Sgnl)"=FALSE ("Value (Signaling)")) -> ()  [unwired: 2 in, 2 out]
          }
        }
      }
      event "Got ADig bead": Value Change {
        n883 = event-data() -> ()  [unwired: 1 in, 5 out]
        n884 = flat-sequence {
          tunnel: w1378 -> [w1382]
          tunnel: w1377 -> [w1381]
          frame #0 {
            n885 = local read "Saved stage positions"() -> (w1384:dbl[][])
            n886 = property on="Inject Pump 1" class="Bool (strict)"("Val(Sgnl)"=FALSE ("Inject Pump 2")) -> ()  [unwired: 2 in, 2 out]
            n887 = case shown="True" "Flow on\ncap 1?" {
              frame False {
              }
              frame True {
                n888 = property on="Inject Sample" class="Bool (strict)"("Val(Sgnl)"=TRUE ("Value (Signaling)")) -> ()  [unwired: 2 in, 2 out]
              }
            }
            n889 = local write "Stage moving"(TRUE ("Stage moving")) -> ()
            n890 = call "move to saved stage position.vi"("error in"=w1381, "Stage VISA resource name in"=w1382, "Position"=1, "Saved Stage Positions"=w1384) -> ()  [unwired: 2 out]
          }
          frame #1 {
            n891 = local read "Shutter 1 (B)"() -> (w1388:bool)
            n892 = disable-structure shown="Disabled" {
              frame Disabled {
                n893 = property on="Inject Pump 2" class="Bool (strict)"("Val(Sgnl)"=TRUE ("Inject Pump 2")) -> ()  [unwired: 2 in, 2 out]
              }
              frame Enabled {
              }
            }
            n894 = local write "Stage moving"(FALSE ("Stage moving")) -> ()
            n895 = case shown="False" w1388 {
              frame False {
                n896 = property on="Shutter 1 (B)" class="Bool (strict)"("Val(Sgnl)"=TRUE ("Value (Signaling)")) -> ()  [unwired: 2 in, 2 out]
              }
              frame True {
              }
            }
            n897 = property on="Inject Sample" class="Bool (strict)"("Val(Sgnl)"=FALSE ("Value (Signaling)")) -> ()  [unwired: 2 in, 2 out]
            n898 = call <vilib>:"Beep.vi"() -> ()  [unwired: 12 in]
          }
        }
        n899 = local write "Got ADig bead"(FALSE ("Got ADig bead")) -> ()
      }
      event "Set Position 1", "Set Position 2", "Set Position 3", "Set Position 4", "Set Position 5": Value Change {
        n900 = event-data() -> ()  [unwired: 1 in, 5 out]
        n901 = Build Array("Set Position 1", "Set Position 2", "Set Position 3", "Set Position 4", "Set Position 5") -> (w1407:bool[])
        n902 = Boolean Array To Number(Boolean array=w1407) -> (number=w1406:u32)
        n903 = call "Read Stage Position.vi"("error in"=w1394, "VISA resource name in"=w1395) -> ("Current Position"=w1392:cluster{dbl, dbl, dbl}, "error out"=→"Stage error":errorcluster)  [unwired: 1 in, 1 out]
        n904 = Logarithm Base 2(1:w1406) -> (0:w1400:dbl)
        n905 = Cluster To Array(cluster=w1392) -> (array=w1402:dbl[])
        n906 = Increment(x=w1400) -> (x+1=w1403:dbl)
        n907 = Build Array (concatenate)(w1403, w1402) -> (w1401:dbl[])
        n908 = Replace Array Subset(array="Saved stage positions", new element=w1401, index (row)=w1400) -> (w1404:dbl[][])  [unwired: 1 in]
        n909 = local write "Saved stage positions"(w1404) -> ()
      }
      event "Move to Position 2", "Move to Position 4", "Move to Position 3", "Move to Position 5", "Move to Position 1": Value Change {
        w1410 = FALSE
        n910 = event-data() -> ()  [unwired: 1 in, 5 out]
        n911 = Build Array("Move to Position 1", "Move to Position 2", "Move to Position 3", "Move to Position 4", "Move to Position 5") -> (w1419:bool[])
        n912 = Boolean Array To Number(Boolean array=w1419) -> (number=w1418:u32)
        n913 = Logarithm Base 2(1:w1418) -> (0:w1417:dbl)
        n914 = flat-sequence {
          tunnel: w1417 -> [w1428]
          tunnel: w1416 -> [w1427]
          tunnel: w1415 -> [w1426]
          tunnel: [w1421] -> w1409
          tunnel: w1409 -> [w1438]
          frame #0 {
            # "only change move time when \nsaving move in T and calibrating is F"
            n915 = local read "Saved stage positions"() -> (w1429:dbl[][])
            n916 = property on="Saving Move" class="Bool (strict)"() -> ("Value"=w1423:bool)  [unwired: 2 in, 2 out]
            n917 = property on="Calibrating" class="Bool (strict)"() -> ("Value"=w1424:bool)  [unwired: 2 in, 2 out]
            n918 = Not(x=w1424) -> (.not. x?=w1422:bool)
            n919 = Increment(x=w1428) -> (x+1=w1421:dbl)
            n920 = And(x=w1423, y=w1422) -> (x .and. y?=w1425:bool)
            n921 = case shown="True" w1425 {
              frame False {
              }
              frame True {
                n922 = Get Date/Time In Seconds() -> (seconds since 1Jan1904=w1435:timestamp)
                n923 = Format Date/Time String(time format string (%c)="%H:%M:%S%3u", seconds (now)=w1435, UTC format=TRUE) -> (date/time string=w1434:string)
                n924 = call <vilib>:"Space Constant.vi"() -> ("String"=w1433:string)
                n925 = Concatenate Strings(w1434, w1433, "moving") -> (w1431:string)
                n926 = property on="Move time" class="Str"("Val(Sgnl)"=w1431) -> ()  [unwired: 2 in, 2 out]
              }
            }
            n927 = call "move to saved stage position.vi"("error in"=w1426, "Stage VISA resource name in"=w1427, "Position"=w1421, "Saved Stage Positions"=w1429) -> ()  [unwired: 2 out]
            n928 = call <vilib>:"Beep.vi"() -> ()  [unwired: 12 in]
            "Stage moving" <- TRUE ("Stage moving")
          }
          frame #1 {
            n929 = property on="Saving Move" class="Bool (strict)"() -> ("Value"=w1440:bool)  [unwired: 2 in, 2 out]
            n930 = property on="Calibrating" class="Bool (strict)"() -> ("Value"=w1441:bool)  [unwired: 2 in, 2 out]
            n931 = call <vilib>:"Beep.vi"() -> ()  [unwired: 12 in]
            n932 = Not(x=w1441) -> (.not. x?=w1439:bool)
            n933 = local write "Stage moving"(FALSE ("Stage moving")) -> ()
            n934 = And(x=w1440, y=w1439) -> (x .and. y?=w1442:bool)
            n935 = case shown="True" w1442 {
              tunnel: w1438 -> [_ w1446]
              frame False {
              }
              frame True {
                n936 = Get Date/Time In Seconds() -> (seconds since 1Jan1904=w1450:timestamp)
                n937 = Format Date/Time String(time format string (%c)="%H:%M:%S%3u", seconds (now)=w1450, UTC format=TRUE) -> (date/time string=w1449:string)
                n938 = Number To Decimal String(number=w1446, width (-)=i16 1) -> (decimal integer string=w1444:string)
                n939 = call <vilib>:"Space Constant.vi"() -> ("String"=w1447:string)
                n940 = Concatenate Strings(w1449, w1447, w1444) -> (w1448:string)
                n941 = property on="Move time" class="Str"("Val(Sgnl)"=w1448) -> ()  [unwired: 2 in, 2 out]
              }
            }
          }
        }
        n942 = local write "Move to Position 1"(w1410) -> ()
        n943 = local write "Move to Position 2"(w1410) -> ()
        n944 = local write "Move to Position 3"(w1410) -> ()
        n945 = local write "Move to Position 4"(w1410) -> ()
        n946 = local write "Move to Position 5"(w1410) -> ()
      }
      event "Set Current\nPos to (0,0,0)": Value Change {
        w1454 = ";" ("string")
        # "DH is \"Define Home\" -KW"
        n947 = event-data() -> ()  [unwired: 1 in, 5 out]
        n948 = local write "Set Current\nPos to (0,0,0)"(FALSE ("Set Current\nPos to (0,0,0)")) -> ()
        n949 = call-poly "VISA Configure Serial Port"("VISA resource name"=w1464, "baud rate (9600)"=u32 19200, "error in (no error)"=w1463) -> ("VISA resource name out"=w1458:refnum<visa-resource-name>, "error out"=w1457:errorcluster)  [unwired: 11 in]
        n950 = Concatenate Strings("1DH" ("string"), w1454, "2DH" ("string"), w1454, "3DH" ("string"), "\r") -> (w1456:string)
        n951 = VISA Write(VISA resource name=w1458, write buffer=w1456, error in (no error)=w1457) -> (error out=w1455:errorcluster)  [unwired: 2 out]
        n952 = local write "Stage error"(w1455) -> ()
      }
      event "Dip": Value Change {
        n953 = event-data() -> ()  [unwired: 1 in, 5 out]
        n954 = property on="Calibrating" class="Bool (strict)"() -> ("Value"=w1471:bool)  [unwired: 2 in, 2 out]
        n955 = Not(x=w1471) -> (.not. x?=w1469:bool)
        n956 = property on="Saving Move" class="Bool (strict)"() -> ("Value"=w1470:bool)  [unwired: 2 in, 2 out]
        n957 = And(x=w1470, y=w1469) -> (x .and. y?=w1468:bool)
        n958 = flat-sequence {
          tunnel: w1479 -> [w1483]
          tunnel: w1478 -> [w1482]
          tunnel: [w1484] -> w1476
          tunnel: [w1483] -> w1474
          tunnel: [w1482] -> w1472
          tunnel: w1468 -> [w1481]
          tunnel: ["Dip position"] -> w1467
          tunnel: [w1500] -> w1477
          tunnel: w1476 -> [w1500]
          tunnel: [w1499] -> w1475
          tunnel: w1474 -> [w1499]
          tunnel: [w1498] -> w1473
          tunnel: w1472 -> [w1498]
          tunnel: w1468 -> [w1494]
          tunnel: w1467 -> [w1493]
          tunnel: w1477 -> [w1531]
          tunnel: w1475 -> [w1530]
          tunnel: w1473 -> [w1529]
          tunnel: w1468 -> [w1527]
          tunnel: ["Start/Return position"] -> w1466
          tunnel: w1468 -> [w1540]
          tunnel: w1466 -> [w1539]
          frame #0 {
            n959 = local read "Saved stage positions"() -> (w1484:dbl[][])
            n960 = case shown="True" w1481 {
              frame False {
              }
              frame True {
                n961 = Get Date/Time In Seconds() -> (seconds since 1Jan1904=w1492:timestamp)
                n962 = call <vilib>:"Space Constant.vi"() -> ("String"=w1488:string)
                n963 = Format Date/Time String(time format string (%c)="%H:%M:%S%3u", seconds (now)=w1492, UTC format=TRUE) -> (date/time string=w1489:string)
                n964 = Concatenate Strings(w1489, w1488, "moving") -> (w1487:string)
                n965 = property on="Move time" class="Str"("Val(Sgnl)"=w1487) -> ()  [unwired: 2 in, 2 out]
              }
            }
            n966 = local write "Stage moving"(TRUE) -> ()
            n967 = call "move to saved stage position.vi"("error in"=w1482, "Stage VISA resource name in"=w1483, "Position"="Dip position", "Saved Stage Positions"=w1484) -> ()  [unwired: 2 out]
          }
          frame #1 {
            n968 = node-c288() -> (w1497:T13)  [unwired: 4 in]
            n969 = case shown="True" w1494 {
              tunnel: w1493 -> [_ w1504]
              frame False {
              }
              frame True {
                n970 = Get Date/Time In Seconds() -> (seconds since 1Jan1904=w1509:timestamp)
                n971 = Number To Decimal String(number=w1504, width (-)=i16 1) -> (decimal integer string=w1503:string)
                n972 = Format Date/Time String(time format string (%c)="%H:%M:%S%3u", seconds (now)=w1509, UTC format=TRUE) -> (date/time string=w1502:string)
                n973 = call <vilib>:"Space Constant.vi"() -> ("String"=w1506:string)
                n974 = Concatenate Strings(w1502, w1506, w1503) -> (w1501:string)
                n975 = property on="Move time" class="Str"("Val(Sgnl)"=w1501) -> ()  [unwired: 2 in, 2 out]
              }
            }
            n976 = timed-loop {
              timing: w1497 -> [_]
              timing-out: [_] -> w1496
              i -> [w1520]
              stop <- w1513 stop-if-true
              n977 = node-c288() -> ()  [unwired: 1 in, 1 out]
              n978 = local read "Cancel Rep\n Dip"() -> (w1510:bool)
              n979 = Greater Or Equal?(x=w1520, y="Dip duration") -> (x >= y?=w1516:bool)
              n980 = local read "Dump beads"() -> (w1511:bool)
              n981 = Or(x=w1516, y="Cancel dwell") -> (x .or. y?=w1515:bool)
              n982 = Not(x="Pause dwell") -> (.not. x?=w1517:bool)
              n983 = node-c288() -> ()  [unwired: 1 in, 1 out]
              n984 = And(x=w1517, y=w1515) -> (x .and. y?=w1514:bool)
              n985 = Compound Arithmetic op=OR(w1514, w1511, w1510) -> (w1513:bool)
              "Dip elasped time" <- w1520
            }
            n986 = local write "Stage moving"(FALSE ("Stage moving")) -> ()
            n987 = node-c288(w1496) -> ()  [unwired: 1 out]
          }
          frame #2 {
            w1525 = FALSE ("Cancel dwell")
            n988 = case shown="True" w1527 {
              frame False {
              }
              frame True {
                n989 = Get Date/Time In Seconds() -> (seconds since 1Jan1904=w1538:timestamp)
                n990 = Format Date/Time String(time format string (%c)="%H:%M:%S%3u", seconds (now)=w1538, UTC format=TRUE) -> (date/time string=w1535:string)
                n991 = call <vilib>:"Space Constant.vi"() -> ("String"=w1534:string)
                n992 = Concatenate Strings(w1535, w1534, "moving") -> (w1532:string)
                n993 = property on="Move time" class="Str"("Val(Sgnl)"=w1532) -> ()  [unwired: 2 in, 2 out]
              }
            }
            n994 = local write "Cancel dwell"(w1525) -> ()
            n995 = local write "Cancel Rep\n Dip"(w1525) -> ()
            n996 = local write "Stage moving"(TRUE) -> ()
            n997 = call "move to saved stage position.vi"("error in"=w1529, "Stage VISA resource name in"=w1530, "Position"="Start/Return position", "Saved Stage Positions"=w1531) -> ()  [unwired: 2 out]
          }
          frame #3 {
            n998 = case shown="True" w1540 {
              tunnel: w1539 -> [_ w1542]
              frame False {
              }
              frame True {
                n999 = Get Date/Time In Seconds() -> (seconds since 1Jan1904=w1550:timestamp)
                n1000 = Number To Decimal String(number=w1542, width (-)=i16 1) -> (decimal integer string=w1543:string)
                n1001 = call <vilib>:"Space Constant.vi"() -> ("String"=w1547:string)
                n1002 = Format Date/Time String(time format string (%c)="%H:%M:%S%3u", seconds (now)=w1550, UTC format=TRUE) -> (date/time string=w1544:string)
                n1003 = Concatenate Strings(w1544, w1547, w1543) -> (w1545:string)
                n1004 = property on="Move time" class="Str"("Val(Sgnl)"=w1545) -> ()  [unwired: 2 in, 2 out]
              }
            }
            n1005 = local write "Stage moving"(FALSE ("Stage moving")) -> ()
          }
          frame #4 {
            n1006 = local write "Dip"(FALSE ("Dip")) -> ()
          }
        }
      }
      event "Repeat Dip": Value Change {
        n1007 = event-data() -> ()  [unwired: 1 in, 6 out]
        n1008 = local read "Saved stage positions"() -> (w1555:dbl[][])
        n1009 = local read "Calibrating"() -> (w1558:bool)
        n1010 = local read "Saving Move"() -> (w1557:bool)
        n1011 = Not(x=w1558) -> (.not. x?=w1556:bool)
        n1012 = And(x=w1557, y=w1556) -> (x .and. y?=w1553:bool)
        n1013 = flat-sequence {
          tunnel: w1555 -> [w1562]
          tunnel: w1554 -> [w1561]
          tunnel: w1553 -> [w1560]
          tunnel: w1552 -> [w1559]
          frame #0 {
            n1014 = while {
              tunnel: w1562 -> [w1579]
              tunnel: w1561 -> [w1576]
              tunnel: w1560 -> [w1573]
              tunnel: w1560 -> [w1572]
              tunnel: w1559 -> [w1571]
              tunnel: w1559 -> [w1570]
              i -> [w1580]
              stop <- w1569 stop-if-true
              n1015 = flat-sequence {
                tunnel: w1579 -> [w1586]
                tunnel: [w1586] -> w1577
                tunnel: w1576 -> [w1585]
                tunnel: [w1585] -> w1574
                tunnel: w1573 -> [w1584]
                tunnel: w1571 -> [w1583]
                tunnel: [w1582] -> w1565
                tunnel: [w1598] -> w1578
                tunnel: w1577 -> [w1598]
                tunnel: [w1597] -> w1575
                tunnel: w1574 -> [w1597]
                tunnel: w1572 -> [w1596]
                tunnel: w1565 -> [w1595]
                tunnel: w1578 -> [w1631]
                tunnel: w1575 -> [w1630]
                tunnel: w1572 -> [w1629]
                tunnel: w1570 -> [w1628]
                tunnel: [w1627] -> w1564
                tunnel: w1572 -> [w1641]
                tunnel: w1564 -> [w1640]
                frame #0 {
                  n1016 = case shown="True" w1584 {
                    frame False {
                    }
                    frame True {
                      n1017 = Get Date/Time In Seconds() -> (seconds since 1Jan1904=w1594:timestamp)
                      n1018 = call <vilib>:"Space Constant.vi"() -> ("String"=w1590:string)
                      n1019 = Format Date/Time String(time format string (%c)="%H:%M:%S%3u", seconds (now)=w1594, UTC format=TRUE) -> (date/time string=w1591:string)
                      n1020 = Concatenate Strings(w1591, w1590, "moving") -> (w1588:string)
                      n1021 = property on="Move time" class="Str"("Val(Sgnl)"=w1588) -> ()  [unwired: 2 in, 2 out]
                    }
                  }
                  n1022 = local read "Dip position"() -> (w1582:dbl)
                  n1023 = local write "Stage moving"(TRUE) -> ()
                  n1024 = call "move to saved stage position.vi"("error in"=w1583, "Stage VISA resource name in"=w1585, "Position"=w1582, "Saved Stage Positions"=w1586) -> ()  [unwired: 2 out]
                }
                frame #1 {
                  # "IN DIPPING POSITION"
                  n1025 = node-c288() -> (w1601:T13)  [unwired: 4 in]
                  n1026 = case shown="True" w1596 {
                    tunnel: w1595 -> [_ w1606]
                    frame False {
                    }
                    frame True {
                      n1027 = Get Date/Time In Seconds() -> (seconds since 1Jan1904=w1610:timestamp)
                      n1028 = Format Date/Time String(time format string (%c)="%H:%M:%S%3u", seconds (now)=w1610, UTC format=TRUE) -> (date/time string=w1605:string)
                      n1029 = Number To Decimal String(number=w1606, width (-)=i16 1) -> (decimal integer string=w1603:string)
                      n1030 = call <vilib>:"Space Constant.vi"() -> ("String"=w1604:string)
                      n1031 = Concatenate Strings(w1605, w1604, w1603) -> (w1602:string)
                      n1032 = property on="Move time" class="Str"("Val(Sgnl)"=w1602) -> ()  [unwired: 2 in, 2 out]
                    }
                  }
                  n1033 = timed-loop {
                    timing: w1601 -> [_]
                    timing-out: [_] -> w1600
                    i -> [w1620]
                    stop <- w1612 stop-if-true
                    n1034 = node-c288() -> ()  [unwired: 1 in, 1 out]
                    n1035 = local read "Dip duration"() -> (w1619:dbl)
                    n1036 = local read "Cancel dwell"() -> (w1618:bool)
                    n1037 = local write "Dip elasped time"(w1620) -> ()
                    n1038 = To Double Precision Float(number=w1620) -> (double precision float=w1621:dbl)
                    n1039 = local read "Pause dwell"() -> (w1622:bool)
                    n1040 = Greater Or Equal?(x=w1621, y=w1619) -> (x >= y?=w1617:bool)
                    n1041 = local read "Dump beads"() -> (w1613:bool)
                    n1042 = Or(x=w1617, y=w1618) -> (x .or. y?=w1616:bool)
                    n1043 = Not(x=w1622) -> (.not. x?=w1615:bool)
                    n1044 = local read "Cancel Rep\n Dip"() -> (w1611:bool)
                    n1045 = And(x=w1615, y=w1616) -> (x .and. y?=w1614:bool)
                    n1046 = node-c288() -> ()  [unwired: 1 in, 1 out]
                    n1047 = Compound Arithmetic op=OR(w1611, w1614, w1613) -> (w1612:bool)
                  }
                  n1048 = local write "Stage moving"(FALSE) -> ()
                  n1049 = node-c288(w1600) -> ()  [unwired: 1 out]
                }
                frame #2 {
                  n1050 = case shown="True" w1629 {
                    frame False {
                    }
                    frame True {
                      n1051 = Get Date/Time In Seconds() -> (seconds since 1Jan1904=w1639:timestamp)
                      n1052 = call <vilib>:"Space Constant.vi"() -> ("String"=w1635:string)
                      n1053 = Format Date/Time String(time format string (%c)="%H:%M:%S%3u", seconds (now)=w1639, UTC format=TRUE) -> (date/time string=w1636:string)
                      n1054 = Concatenate Strings(w1636, w1635, "moving") -> (w1633:string)
                      n1055 = property on="Move time" class="Str"("Val(Sgnl)"=w1633) -> ()  [unwired: 2 in, 2 out]
                    }
                  }
                  n1056 = local read "Start/Return position"() -> (w1627:dbl)
                  n1057 = local write "Stage moving"(TRUE) -> ()
                  n1058 = call "move to saved stage position.vi"("error in"=w1628, "Stage VISA resource name in"=w1630, "Position"=w1627, "Saved Stage Positions"=w1631) -> ()  [unwired: 2 out]
                }
                frame #3 {
                  # "IN RETURN POSITION"
                  n1059 = node-c288() -> (w1644:T13)  [unwired: 4 in]
                  n1060 = timed-loop {
                    timing: w1644 -> [_]
                    timing-out: [_] -> w1643
                    i -> [w1664]
                    stop <- w1655 stop-if-true
                    n1061 = node-c288() -> ()  [unwired: 1 in, 1 out]
                    n1062 = local read "Return duration"() -> (w1662:dbl)
                    n1063 = local read "Cancel dwell"() -> (w1660:bool)
                    n1064 = local write "Return elasped time"(w1664) -> ()
                    n1065 = To Double Precision Float(number=w1664) -> (double precision float=w1665:dbl)
                    n1066 = local read "Pause dwell"() -> (w1663:bool)
                    n1067 = Greater Or Equal?(x=w1665, y=w1662) -> (x >= y?=w1661:bool)
                    n1068 = local read "Dump beads"() -> (w1656:bool)
                    n1069 = Or(x=w1661, y=w1660) -> (x .or. y?=w1659:bool)
                    n1070 = local read "Cancel Rep\n Dip"() -> (w1654:bool)
                    n1071 = Not(x=w1663) -> (.not. x?=w1658:bool)
                    n1072 = node-c288() -> ()  [unwired: 1 in, 1 out]
                    n1073 = And(x=w1658, y=w1659) -> (x .and. y?=w1657:bool)
                    n1074 = Compound Arithmetic op=OR(w1654, w1657, w1656) -> (w1655:bool)
                  }
                  n1075 = case shown="True" w1641 {
                    tunnel: w1640 -> [_ w1649]
                    frame False {
                    }
                    frame True {
                      n1076 = Get Date/Time In Seconds() -> (seconds since 1Jan1904=w1653:timestamp)
                      n1077 = Format Date/Time String(time format string (%c)="%H:%M:%S%3u", seconds (now)=w1653, UTC format=TRUE) -> (date/time string=w1646:string)
                      n1078 = Number To Decimal String(number=w1649, width (-)=i16 1) -> (decimal integer string=w1648:string)
                      n1079 = call <vilib>:"Space Constant.vi"() -> ("String"=w1647:string)
                      n1080 = Concatenate Strings(w1646, w1647, w1648) -> (w1645:string)
                      n1081 = property on="Move time" class="Str"("Val(Sgnl)"=w1645) -> ()  [unwired: 2 in, 2 out]
                    }
                  }
                  n1082 = local write "Stage moving"(FALSE) -> ()
                  n1083 = node-c288(w1643) -> ()  [unwired: 1 out]
                }
              }
              n1084 = Increment(x=w1580) -> (x+1=w1567:i32)
              "Dip #" <- w1567
              n1085 = property on="Cancel Rep\n Dip" class="Bool (strict)"() -> ("Value"=w1563:bool)  [unwired: 2 in, 2 out]
              n1086 = To Double Precision Float(number=w1567) -> (double precision float=w1566:dbl)
              n1087 = Greater Or Equal?(x=w1566, y="Dip attempts") -> (x >= y?=w1581:bool)
              n1088 = Or(x=w1563, y=w1581) -> (x .or. y?=w1569:bool)
            }
          }
          frame #1 {
            w1670 = FALSE
            n1089 = local write "Cancel Rep\n Dip"(w1670) -> ()
            n1090 = call <vilib>:"Beep.vi"() -> ()  [unwired: 12 in]
            n1091 = local write "Repeat Dip"(w1670) -> ()
          }
        }
      }
      event "Force FB script": Value Change {
        n1092 = event-data() -> ()  [unwired: 1 in, 5 out]
        n1093 = flat-sequence {
          frame #0 {
            n1094 = disable-structure shown="Disabled" {
              frame Disabled {
                n1095 = local read "# Samples/channel"() -> (w1673:i32)
                n1096 = local write "# Samples/channel (in)"(w1673) -> ()
              }
              frame Enabled {
              }
            }
            n1097 = local write "Force FB script"(FALSE ("Force FB script")) -> ()
            n1098 = property on="Trap delta (nm)" class="DigNum (strict)"("Val(Sgnl)"="Start trap delta (nm)") -> ()  [unwired: 2 in, 2 out]
          }
          frame #1 {
            n1099 = Wait (ms)(milliseconds to wait=u32 500) -> ()  [unwired: 1 out]
          }
          frame #2 {
            n1100 = property on="Set reading to\nsetpoint 1" class="Bool (strict)"("Val(Sgnl)"=TRUE ("Value (Signaling)")) -> ()  [unwired: 2 in, 2 out]
          }
          frame #3 {
            n1101 = Wait (ms)(milliseconds to wait=u32 300) -> ()  [unwired: 1 out]
          }
          frame #4 {
            n1102 = local write "Force Feedback 1"(TRUE ("Force Feedback")) -> ()
            n1103 = property on="Tabs" class="TabCtl (strict)"("Val(Sgnl)"=T23."Force Feedback" ("Value (Signaling)")) -> ()  [unwired: 2 in, 2 out]
          }
          frame #5 {
            n1104 = property on="Save Data" class="Bool (strict)"("Val(Sgnl)"=TRUE ("Value (Signaling)")) -> ()  [unwired: 2 in, 2 out]
          }
          frame #6 {
            n1105 = Multiply(x="Wait before dip (s)", y=1000) -> (x*y=w1680:dbl)
            n1106 = Wait (ms)(milliseconds to wait=w1680) -> ()  [unwired: 1 out]
          }
          frame #7 {
            n1107 = case shown="True" "Start dipping after?" {
              selector: "Start dipping after?" -> [_ w1685]
              frame False {
              }
              frame True {
                n1108 = property on="Dip" class="Bool (strict)"("Val(Sgnl)"=w1685) -> ()  [unwired: 2 in, 2 out]
              }
            }
            n1109 = property on="Remove offsets" class="Bool (strict)"("Val(Sgnl)"=TRUE ("Value (Signaling)")) -> ()  [unwired: 2 in, 2 out]
          }
        }
      }
      event "Move 0": Value Change {
        n1110 = event-data() -> ()  [unwired: 1 in, 5 out]
        n1111 = local write "Move 0"(FALSE) -> ()
        n1112 = call "HalfWavePlate.vi"("Degrees"="\"Degrees\" 0", "Motor"=0) -> ()  [unwired: 1 in]
      }
      event "Move 1": Value Change {
        n1113 = event-data() -> ()  [unwired: 1 in, 5 out]
        n1114 = local write "Move 1"(FALSE) -> ()
        n1115 = call "HalfWavePlate.vi"("Degrees"="\"Degrees\" 1", "Motor"=1) -> ()  [unwired: 1 in]
      }
      event "Save user params": Value Change {
        n1116 = event-data() -> ()  [unwired: 1 in, 6 out]
        n1117 = local write "Save user params"(FALSE) -> ()
        n1118 = call "save control values.vi"("User"="User") -> ()  [unwired: 8 in, 1 out]
      }
      event "Load user params": Value Change {
        # "Exceptions. Don't load these parameters."
        n1119 = event-data() -> ()  [unwired: 1 in, 6 out]
        n1120 = local write "Load user params"(FALSE) -> ()
        n1121 = flat-sequence {
          tunnel: [w1718] -> w1709
          tunnel: [w1717] -> w1707
          tunnel: [w1716] -> w1705
          tunnel: [w1715] -> w1703
          tunnel: [w1714] -> w1701
          tunnel: [w1713] -> w1699
          tunnel: [w1712] -> w1697
          tunnel: [w1711] -> w1694
          tunnel: [w1726] -> w1710
          tunnel: w1709 -> [w1726]
          tunnel: [w1725] -> w1708
          tunnel: w1707 -> [w1725]
          tunnel: [w1724] -> w1706
          tunnel: w1705 -> [w1724]
          tunnel: [w1723] -> w1704
          tunnel: w1703 -> [w1723]
          tunnel: [w1722] -> w1702
          tunnel: w1701 -> [w1722]
          tunnel: [w1721] -> w1700
          tunnel: w1699 -> [w1721]
          tunnel: [w1720] -> w1698
          tunnel: w1697 -> [w1720]
          tunnel: [w1719] -> w1695
          tunnel: w1694 -> [w1719]
          tunnel: w1710 -> [w1735]
          tunnel: w1708 -> [w1734]
          tunnel: w1706 -> [w1733]
          tunnel: w1704 -> [w1732]
          tunnel: w1702 -> [w1731]
          tunnel: w1700 -> [w1730]
          tunnel: w1698 -> [w1729]
          tunnel: w1695 -> [w1728]
          frame #0 {
            n1122 = local read "Force Feedback 2"() -> (w1711:bool)
            n1123 = local read "Force Feedback 1"() -> (w1712:bool)
            n1124 = local read "Shutter 1 (B)"() -> (w1718:bool)
            n1125 = local read "Shutter 2 (A)"() -> (w1717:bool)
            n1126 = local read "Inject Sample"() -> (w1715:bool)
            n1127 = local read "Trap delta (nm)"() -> (w1714:dbl)
            n1128 = local read "Save file index"() -> (w1713:i32)
            n1129 = local read "Fish"() -> (w1716:bool)
          }
          frame #1 {
            n1130 = local read "User"() -> (w1727:string)
            n1131 = call "retrieve control values.vi"("User"=w1727) -> ()  [unwired: 10 in, 1 out]
          }
          frame #2 {
            n1132 = local write "Force Feedback 1"(w1729) -> ()
            n1133 = local write "Force Feedback 2"(w1728) -> ()
            n1134 = local write "Trap delta (nm)"(w1731) -> ()
            n1135 = local write "Save file index"(w1730) -> ()
            n1136 = local write "Inject Sample"(w1732) -> ()
            n1137 = local write "Shutter 2 (A)"(w1734) -> ()
            n1138 = local write "Shutter 1 (B)"(w1735) -> ()
            n1139 = local write "Fish"(w1733) -> ()
          }
        }
      }
      event "Stop": Value Change {
        n1140 = event-data() -> ()  [unwired: 1 in, 5 out]
        n1141 = local read "Stop"() -> (w1736:bool)
      }
    }
    n1142 = node-c288() -> ()  [unwired: 1 in, 1 out]
  }
  n1143 = call-poly <vilib>:"DAQmx Create Virtual Channel.vi"("lines"=w98) -> ("task out"=w97:refnum<k21>)  [unwired: 13 in, 1 out]
  n1144 = call-poly <vilib>:"DAQmx Create Virtual Channel.vi"("lines"=w101) -> ("task out"=w100:refnum<k21>)  [unwired: 13 in, 1 out]
  n1145 = node-c288(2 ("Processor")) -> (w82:T13)  [unwired: 3 in]
  n1146 = timed-loop {
    timing: w82 -> [_]
    timing-out: [_] -> w81
    stop <- w1739 stop-if-true
    n1147 = node-c288() -> ()  [unwired: 1 in, 1 out]
    n1148 = case shown="\"Control\"" "Tab Control" {
      frame "Control" {
        n1149 = case shown="True" "Start" {
          frame False {
          }
          frame True {
            w1752 = T24 3 items=["no dialog", "OK message", "continue or stop message", "OK message + warnings", "continue/stop + warnings"] ("type of dialog (OK msg:1)")
            n1150 = call "InitializeAcquireFF.vi"("DAQ Rate"="DAQ Rate", "Averaging Number"="Averaging Number", "Sampling Rate"="Sampling Rate") -> ("error out"=w1746:errorcluster, "task out"=w1745:refnum<k21>, "Final Sampling Rate"=→"Final Sampling Rate":dbl)  [unwired: 4 in, 2 out]
            n1151 = while {
              tunnel: [w1764] -> w1751
              tunnel: [w1763] -> w1744
              tunnel: "Averaging Number" -> [w1762]
              tunnel: w1746 -> [w1761]
              tunnel: w1745 -> [w1759]
              stop <- w1760 continue-if-true
              n1152 = call "Acquire2_QPD.vi"("task/channels in"=w1759, "Save Data?"=FALSE ("Take Data?"), "Averaging Number"=w1762, "error in"=w1761) -> ("PSD 1"=→"PSD 1":cluster{dbl[], dbl[]}, "PSD 1 Sum"=→"PSD 1 Sum":dbl, "PSD 2"=→"PSD 2":cluster{dbl[], dbl[]}, "PSD 2 Sum"=→"PSD 2 Sum":dbl, "task out"=w1764:refnum<k21>, "error out"=w1763:errorcluster)  [unwired: 14 in, 4 out]
              n1153 = local read "Start"() -> (w1760:bool)
            }
            n1154 = call <vilib>:"DAQmx Clear Task.vi"("task in"=w1751, "error in"=w1744) -> ("error out"=w1753:errorcluster)  [unwired: 13 in]
            n1155 = call <vilib>:"Simple Error Handler.vi"("type of dialog (OK msg:1)"=w1752, "error in (no error)"=w1753) -> ()  [unwired: 3 in, 5 out]
          }
        }
      }
      frame "Current Saved Data" {
      }
      frame "Data Acquisition" {
      }
      frame "Raw QPD Data" {
      }
    }
    n1156 = local read "Stop"() -> (w1739:bool)
    n1157 = node-c288() -> ()  [unwired: 1 in, 1 out]
  }
  n1158 = node-c288(2 ("Processor")) -> (w34:T13)  [unwired: 3 in]
  n1159 = timed-loop {
    timing: w34 -> [_]
    timing-out: [_] -> w33
    stop <- w1765 stop-if-true
    n1160 = node-c288() -> ()  [unwired: 1 in, 1 out]
    n1161 = event shown="[0] \"Pause Mouse/Mirror Connection\": Value Change" {
      selector: _ -> [_ _]
      dyn-events: _ -> [_ _]
      timeout: _ -> [_ _]
      tunnel: [w1858 _] -> w1766
      tunnel: [_ w1859] -> w1765
      event "Pause Mouse/Mirror Connection": Value Change {
        n1162 = event-data() -> ("NewVal"=w1858:bool)  [unwired: 1 in]
      }
      event "Stop": Value Change {
        n1163 = event-data() -> ("NewVal"=w1859:bool)  [unwired: 1 in]
      }
    }
    n1164 = case shown="True" w1766 {
      frame False {
      }
      frame True {
        n1165 = call "InitializeMouseControl.vi"() -> ("error out 2"=w1775:errorcluster, "task out"=w1776:refnum<k21>, "error out"=w1778:errorcluster, "device ID"=w1777:refnum<k1>)  [unwired: 8 in]
        n1166 = while {
          tunnel: w1778 -> [w1790]
          tunnel: w1777 -> [w1789]
          tunnel: w1776 -> [w1788]
          tunnel: w1775 -> [w1787]
          tunnel: [w1786] -> w1773
          tunnel: [w1785] -> w1772
          tunnel: [w1784] -> w1769
          tunnel: [w1783] -> w1770
          stop <- w1782 stop-if-true
          n1167 = case shown="True" "Use Mouse to Move Trap?" {
            tunnel: w1789 -> [w1797 w1820]
            tunnel: w1790 -> [w1796 w1819]
            tunnel: w1788 -> [w1795 w1818]
            tunnel: w1787 -> [w1794 w1817]
            tunnel: [w1797 w1816] -> w1784
            tunnel: [w1796 w1815] -> w1783
            tunnel: [w1795 w1814] -> w1786
            tunnel: [w1794 w1813] -> w1785
            frame False {
              (unwired) FALSE ("button 1")
            }
            frame True {
              w1808 = 0.0 ("y")
              w1810 = 10
              n1168 = local read "Deflection"() -> (w1821:T5)
              n1169 = call-poly <vilib>:"Acquire Input Data.vi"("device ID"=w1820, "error in (no error)"=w1819) -> ("device ID"=w1816:refnum<k1>, "button info"=w1834:T25, "error out"=w1815:errorcluster)  [unwired: 14 in, 1 out]
              n1170 = Unbundle By Name(w1821) -> ("Horizontal"=w1823:i32, "Vertical"=w1822:i32)
              n1171 = local read "Saved voltage"() -> (w1799:cluster{dbl, dbl})
              n1172 = Divide(x=w1823, y=30) -> (x/y=w1826:dbl)
              n1173 = Divide(x=w1822, y=-20) -> (x/y=w1827:dbl)
              n1174 = Unbundle By Name(w1834) -> ("button 1"=w1812:bool, "button 2"=w1828:bool)
              n1175 = Bundle(w1826, w1827) -> (w1804:cluster{dbl, dbl})  [unwired: 1 in]
              n1176 = local write "Reference Voltage"(w1804) -> ()
              n1177 = Add(x=w1804, y=w1799) -> (x+y=w1832:cluster{dbl, dbl})
              n1178 = case shown="True" w1812 {
                frame False {
                  n1179 = stacked-sequence {
                    frame #0 {
                      n1180 = local write "CoordinatesMousePressed"(T5 {"Horizontal"=0, "Vertical"=0} ("Coords when pressed")) -> ()
                      n1181 = local write "Deflection"(T5 {"Horizontal"=0, "Vertical"=0} ("deflaction")) -> ()
                    }
                  }
                }
                frame True {
                  n1182 = local read "CoordinatesMousePressed"() -> (w1857:T5)
                  n1183 = local read "Real Coordinates"() -> (w1856:cluster{"Horizontal":i32, "Vertical":i32})
                  n1184 = Subtract(x=w1856, y=w1857) -> (x-y=w1855:T5)
                  n1185 = local write "Deflection"(w1855) -> ()
                }
              }
              n1186 = Unbundle(w1832) -> (w1809:dbl, w1800:dbl)
              n1187 = case shown="True" w1828 {
                frame False {
                }
                frame True {
                  n1188 = local read "Reference Voltage"() -> (w1838:cluster{dbl, dbl})
                  n1189 = local read "Saved voltage"() -> (w1836:cluster{dbl, dbl})
                  n1190 = Add(x=w1838, y=w1836) -> (x+y=→"Saved voltage":cluster{dbl, dbl})
                  n1191 = local read "Real Coordinates"() -> (w1837:cluster{"Horizontal":i32, "Vertical":i32})
                  n1192 = local write "CoordinatesMousePressed"(w1837) -> ()
                }
              }
              n1193 = Less?(x=w1809, y=w1810) -> (x < y?=w1807:bool)
              n1194 = Greater?(x=w1809, y=w1808) -> (0:w1806:bool)
              n1195 = Greater?(x=w1800, y=w1808) -> (0:w1802:bool)
              n1196 = Less?(x=w1800, y=w1810) -> (x < y?=w1803:bool)
              n1197 = And(x=w1802, y=w1803) -> (x .and. y?=w1801:bool)
              n1198 = And(x=w1807, y=w1806) -> (x .and. y?=w1805:bool)
              n1199 = case shown="False" w1801 {
                tunnel: [w1848 w1852] -> w1811
                tunnel: w1800 -> [w1846 w1852]
                frame False {
                  n1200 = Greater?(x=w1846, y=10.0) -> (0:w1849:bool)
                  n1201 = case shown="True" w1849 {
                    tunnel: [0.0 10.0] -> w1848
                    frame False {
                    }
                    frame True {
                    }
                  }
                }
                frame True {
                }
              }
              n1202 = case shown="False" w1805 {
                tunnel: w1809 -> [w1840 w1845]
                tunnel: [w1841 w1845] -> w1833
                frame False {
                  n1203 = Greater?(x=w1840, y=10.0) -> (0:w1842:bool)
                  n1204 = case shown="True" w1842 {
                    tunnel: [0.0 10.0] -> w1841
                    frame False {
                    }
                    frame True {
                    }
                  }
                }
                frame True {
                }
              }
              n1205 = Bundle(w1833, w1811) -> (w1798:cluster{dbl, dbl})  [unwired: 1 in]
              n1206 = Cluster To Array(cluster=w1798) -> (array=w1829:dbl[])
              n1207 = call-poly <vilib>:"DAQmx Write.vi"("task/channels in"=w1818, "data"=w1829, "error in"=w1817) -> ("task out"=w1831:refnum<k21>, "error out"=w1830:errorcluster)  [unwired: 10 in, 1 out]
              n1208 = call <vilib>:"DAQmx Is Task Done.vi"("task/channels in"=w1831, "error in"=w1830) -> ("task out"=w1814:refnum<k21>, "error out"=w1813:errorcluster)  [unwired: 11 in, 1 out]
            }
          }
          n1209 = event shown="[0] \"Pane\": Mouse Move" {
            selector: _ -> [_ _ _]
            dyn-events: _ -> [_ _ _]
            timeout: _ -> [_ _ _]
            event Mouse Move {
              n1210 = event-data() -> ("Coords"=w1792:T5)  [unwired: 1 in]
              n1211 = local write "Real Coordinates"(w1792) -> ()
            }
            event Mouse Down {
              n1212 = event-data() -> ("Coords"=w1793:T5)  [unwired: 1 in]
              n1213 = local write "CoordinatesMousePressed"(w1793) -> ()
            }
            event "Pause Mouse/Mirror Connection": Value Change {
              n1214 = event-data() -> ()  [unwired: 1 in, 3 out]
            }
          }
          n1215 = local read "Stop"() -> (w1779:bool)
          n1216 = Not(x="Pause Mouse/Mirror Connection") -> (.not. x?=w1780:bool)
          n1217 = Or(x=w1780, y=w1779) -> (x .or. y?=w1782:bool)
        }
        n1218 = call <vilib>:"DAQmx Clear Task.vi"("task in"=w1773, "error in"=w1772) -> ("error out"=w1774:errorcluster)  [unwired: 13 in]
        n1219 = call <vilib>:"Simple Error Handler.vi"("error in (no error)"=w1774) -> ()  [unwired: 4 in, 5 out]
        n1220 = call-poly <vilib>:"Close Input Device.vi"("error in (no error)"=w1770, "device ID"=w1769) -> ("error out"=w1771:errorcluster)  [unwired: 8 in]
        n1221 = call <vilib>:"Simple Error Handler.vi"("error in (no error)"=w1771) -> ()  [unwired: 4 in, 5 out]
      }
    }
    n1222 = node-c288() -> ()  [unwired: 1 in, 1 out]
  }
  n1223 = node-c288(i64 100 ("Period")) -> (w95:T13)  [unwired: 3 in]
  n1224 = timed-loop {
    tunnel: w97 -> [w1862]
    tunnel: [w1861] -> w96
    tunnel: w100 -> [w1864]
    tunnel: [w1863] -> w99
    timing: w95 -> [_]
    timing-out: [_] -> w94
    stop <- w1860 stop-if-true
    n1225 = node-c288() -> ()  [unwired: 1 in, 1 out]
    n1226 = event shown="[1] \"Shutter 2 (A)\": Value Change" {
      selector: _ -> [_ _ _]
      dyn-events: _ -> [_ _ _]
      timeout: _ -> [_ _ _]
      tunnel: w1864 -> [w1868 _ w1905]
      tunnel: [w1867 _ w1905] -> w1863
      tunnel: w1862 -> [_ w1888 w1906]
      tunnel: [_ w1886 w1906] -> w1861
      tunnel: [_ _ w1907] -> w1860
      event "Shutter 1 (B)": Value Change {
        n1227 = event-data() -> ()  [unwired: 1 in, 1 out]
        n1228 = flat-sequence {
          tunnel: [w1874] -> w1871
          tunnel: w1868 -> [w1873]
          tunnel: [w1878] -> w1870
          tunnel: [w1881] -> w1869
          tunnel: w1871 -> [w1876]
          tunnel: w1870 -> [w1885]
          tunnel: w1869 -> [w1883]
          tunnel: [w1882] -> w1867
          frame #0 {
            n1229 = call-poly <vilib>:"DAQmx Write.vi"("task/channels in"=w1873, "data"=FALSE) -> ("task out"=w1874:refnum<k21>)  [unwired: 11 in, 2 out]
            n1230 = Wait (ms)(milliseconds to wait=100) -> ()  [unwired: 1 out]
          }
          frame #1 {
            n1231 = Or(x="Shutter 1 (B)", y=TRUE) -> (x .or. y?=w1878:bool)
            n1232 = call-poly <vilib>:"DAQmx Write.vi"("task/channels in"=w1876, "data"=w1878) -> ("task out"=w1881:refnum<k21>)  [unwired: 11 in, 2 out]
            n1233 = Wait (ms)(milliseconds to wait=100) -> ()  [unwired: 1 out]
          }
          frame #2 {
            n1234 = Not(x=w1885) -> (.not. x?=w1884:bool)
            n1235 = call-poly <vilib>:"DAQmx Write.vi"("task/channels in"=w1883, "data"=w1884) -> ("task out"=w1882:refnum<k21>)  [unwired: 11 in, 2 out]
          }
        }
      }
      event "Shutter 2 (A)": Value Change {
        n1236 = event-data() -> ()  [unwired: 1 in, 1 out]
        n1237 = flat-sequence {
          tunnel: w1888 -> [w1893]
          tunnel: [w1892] -> w1887
          tunnel: [w1897] -> w1890
          tunnel: [w1900] -> w1889
          tunnel: w1887 -> [w1895]
          tunnel: w1890 -> [w1904]
          tunnel: w1889 -> [w1902]
          tunnel: [w1901] -> w1886
          frame #0 {
            n1238 = call-poly <vilib>:"DAQmx Write.vi"("task/channels in"=w1893, "data"=FALSE) -> ("task out"=w1892:refnum<k21>)  [unwired: 11 in, 2 out]
            n1239 = Wait (ms)(milliseconds to wait=100) -> ()  [unwired: 1 out]
          }
          frame #1 {
            n1240 = Or(x="Shutter 2 (A)", y=TRUE) -> (x .or. y?=w1897:bool)
            n1241 = call-poly <vilib>:"DAQmx Write.vi"("task/channels in"=w1895, "data"=w1897) -> ("task out"=w1900:refnum<k21>)  [unwired: 11 in, 2 out]
            n1242 = Wait (ms)(milliseconds to wait=100) -> ()  [unwired: 1 out]
          }
          frame #2 {
            n1243 = Not(x=w1904) -> (.not. x?=w1903:bool)
            n1244 = call-poly <vilib>:"DAQmx Write.vi"("task/channels in"=w1902, "data"=w1903) -> ("task out"=w1901:refnum<k21>)  [unwired: 11 in, 2 out]
          }
        }
      }
      event "Stop": Value Change {
        n1245 = event-data() -> ("NewVal"=w1907:bool)  [unwired: 1 in, 5 out]
      }
    }
    n1246 = node-c288() -> ()  [unwired: 1 in, 1 out]
  }
  n1247 = node-c288(w94) -> ()  [unwired: 1 out]
  n1248 = node-c288(w81) -> ()  [unwired: 1 out]
  n1249 = call <vilib>:"DAQmx Clear Task.vi"("task in"=w96) -> ()  [unwired: 14 in, 1 out]
  n1250 = call <vilib>:"DAQmx Clear Task.vi"("task in"=w99) -> ()  [unwired: 14 in, 1 out]
  n1251 = node-c288(w33) -> ()  [unwired: 1 out]
  n1252 = node-c288(w29) -> ()  [unwired: 1 out]
  n1253 = local write "Tether"(FALSE ("Tether")) -> ()
  n1254 = local read "Path"() -> (w88:path)
  n1255 = node-c288(i64 1 ("Period"), 2 ("Processor")) -> (w93:T13)  [unwired: 2 in]
  n1256 = timed-loop {
    timing: w93 -> [_]
    timing-out: [_] -> w92
    tunnel: w88 -> [w1909]
    stop <- w1908 stop-if-true
    n1257 = node-c288() -> ()  [unwired: 1 in, 1 out]
    n1258 = event shown="[5] \"Fish\": Value Change" {
      selector: _ -> [_ _ _ _ _ _ _ _ _ _]
      dyn-events: _ -> [_ _ _ _ _ _ _ _ _ _]
      timeout: _ -> [_ _ _ _ _ _ _ _ _ _]
      tunnel: w1909 -> [_ w1913 _ _ _ _ _ _ _ _]
      tunnel: [_ _ w1933 _ _ _ _ _ _ _] -> w1908
      event Timeout {
        n1259 = event-data() -> ()  [unwired: 1 in, 2 out]
      }
      event "Read Cal": Value Change {
        n1260 = event-data() -> ()  [unwired: 1 in, 6 out]
        n1261 = Path To String(path=w1913) -> (string=w1912:string)
        n1262 = Format Date/Time String(time format string (%c)="%y%m%d") -> (date/time string=w1914:string)  [unwired: 2 in]
        n1263 = Concatenate Strings(w1912, "\\" ("string"), w1914, "\\" ("string"), "current.cal") -> (w1932:string)
        n1264 = String To Path(string=w1932) -> (path=w1931:path)
        n1265 = Open/Create/Replace File(file path (use dialog)=w1931, operation (0:open)=T18."open", access (0:read/write)=enum16{"read/write", "read-only", "write-only"}."read-only") -> (refnum out=w1927:refnum<file>, error out=w1928:errorcluster)  [unwired: 3 in, 1 out]
        n1266 = Deny Access(4:w1928, 7:w1927) -> (0:w1926:errorcluster, 3:w1925:refnum<file>)  [unwired: 1 in]
        n1267 = Read from Binary File(5:0.0, 8:w1926, 9:T19."big-endian, network order" ("byte order (0:big-endian, network order)"), 10:12 ("count"), 11:w1925) -> (0:w1921:errorcluster, 2:w1919:dbl[], 3:w1922:refnum<file>)  [unwired: 1 in, 1 out]
        n1268 = Array To Cluster(array=w1919) -> (cluster=→"Cal values":T26)
        n1269 = Close File(refnum=w1922, error in=w1921) -> ()  [unwired: 2 out]
        n1270 = local write "Read Cal"(FALSE ("Read Cal")) -> ()
      }
      event "Stop": Value Change {
        n1271 = event-data() -> ("NewVal"=w1933:bool)  [unwired: 1 in, 5 out]
      }
      event "Trap position (V)": Value Change {
        # "Need to rotate so X and Y don't get mixed up."
        n1272 = event-data() -> ()  [unwired: 1 in, 6 out]
        n1273 = local read "Mirror task"() -> (w1934:refnum<k21>)
        n1274 = Cluster To Array(cluster="Trap position (V)") -> (array=w1937:dbl[])
        n1275 = Rotate 1D Array(1:w1937, 2:1 ("n")) -> (0:w1935:dbl[])
        n1276 = call-poly <vilib>:"DAQmx Write.vi"("task/channels in"=w1934, "data"=w1935) -> ("task out"=w1940:refnum<k21>, "error out"=w1939:errorcluster)  [unwired: 11 in, 1 out]
        n1277 = call <vilib>:"DAQmx Stop Task.vi"("task/channels in"=w1940, "error in"=w1939) -> ("error out"=w1938:errorcluster)  [unwired: 12 in, 1 out]
        n1278 = call <vilib>:"Simple Error Handler.vi"("error in (no error)"=w1938) -> ()  [unwired: 4 in, 5 out]
      }
      event "Trap delta (nm)": Value Change {
        n1279 = event-data() -> ()  [unwired: 1 in, 6 out]
        n1280 = local read "Pulling direction"() -> (w1942:bool)
        n1281 = local read "Conv Y (nm/V)"() -> (w1943:dbl)
        n1282 = local read "Conv X (nm/V)"() -> (w1944:dbl)
        n1283 = Select(t=w1943, s=w1942, f=w1944) -> (s? t:f=w1945:dbl)
        n1284 = local read "Fixed Y"() -> (w1951:dbl)
        n1285 = Divide(x="Trap delta (nm)", y=w1945) -> (x/y=w1946:dbl)
        n1286 = local read "Fixed X"() -> (w1950:dbl)
        n1287 = Select(t=w1951, s=w1942, f=w1950) -> (s? t:f=w1949:dbl)
        n1288 = Add(x=w1946, y=w1949) -> (x+y=w1947:dbl)
        n1289 = case shown="False" w1942 {
          tunnel: w1947 -> [w1952 w1953]
          frame False {
            n1290 = property on="X" class="DigNum (strict)"("Val(Sgnl)"=w1952) -> ()  [unwired: 2 in, 2 out]
          }
          frame True {
            n1291 = property on="Y" class="DigNum (strict)"("Val(Sgnl)"=w1953) -> ()  [unwired: 2 in, 2 out]
          }
        }
      }
      event "Fish": Value Change {
        n1292 = event-data() -> ()  [unwired: 1 in, 6 out]
        n1293 = local read "Fish"() -> (w1954:bool)
        n1294 = case shown="True" w1954 {
          frame False {
          }
          frame True {
            w1964 = 0.0 ("minimum value")
            w1965 = 10.0 ("maximum value")
            # "Grab offset in pulling\ndirection and add to \ndelta values"
            n1295 = call-poly <vilib>:"DAQmx Create Virtual Channel.vi"("maximum value"=w1965, "minimum value"=w1964, "physical channels"=tag "Dev1/ao0") -> ("task out"=w1969:refnum<k21>, "error out"=w1968:errorcluster)  [unwired: 11 in]
            n1296 = call-poly <vilib>:"DAQmx Create Virtual Channel.vi"("task in"=w1969, "maximum value"=w1965, "minimum value"=w1964, "physical channels"=tag "Dev1/ao1", "error in"=w1968) -> ("task out"=w1963:refnum<k21>, "error out"=w1962:errorcluster)  [unwired: 9 in]
            n1297 = node-c288(i64 1 ("Period")) -> (w1971:T13)  [unwired: 3 in]
            n1298 = timed-loop {
              timing: w1971 -> [_]
              timing-out: [_] -> w1970
              tunnel: w1963 -> [w2040]
              tunnel: w1962 -> [w2039]
              tunnel: [w2038] -> w1959
              tunnel: [w2037] -> w1958
              tunnel: [w1997] -> w1960
              tunnel: [w1998] -> w1957
              i -> [w2023]
              stop <- w1998 stop-if-true
              # "x direction"
              # "y direction"
              # "Send offset in direction\nof not-pulling to DAQ"
              n1299 = node-c288() -> ()  [unwired: 1 in, 1 out]
              n1300 = local read "Pulling direction"() -> (w2002:bool)
              n1301 = local read "Conv Y (nm/V)"() -> (w2004:dbl)
              n1302 = local read "Conv X (nm/V)"() -> (w2003:dbl)
              n1303 = local read "Fixed X"() -> (w2011:dbl)
              n1304 = local read "Fixed Y"() -> (w2010:dbl)
              n1305 = Select(t=w2010, s=w2002, f=w2011) -> (s? t:f=w2012:dbl)
              n1306 = Select(t=w2011, s=w2002, f=w2010) -> (s? t:f=w2009:dbl)
              n1307 = Select(t=w2004, s=w2002, f=w2003) -> (s? t:f=w1999:dbl)
              n1308 = Divide(x="Max fish\ndelta (nm)", y=w1999) -> (x/y=w2001:dbl)
              n1309 = Divide(x="Min fish\ndelta (nm)", y=w1999) -> (x/y=w2000:dbl)
              n1310 = Add(x=w2012, y=w2001) -> (x+y=w2014:dbl)
              n1311 = Subtract(x=w2001, y=w2000) -> (x-y=w2016:dbl)
              n1312 = Divide(x=w2016, y="Fish Speed (ms)") -> (x/y=w2017:dbl)
              n1313 = flat-sequence {
                tunnel: w2002 -> [w2060]
                tunnel: w2009 -> [w2059]
                tunnel: w2040 -> [w2058]
                tunnel: w2039 -> [w2057]
                tunnel: w2017 -> [w2056]
                tunnel: w2014 -> [w2055]
                tunnel: "Fish Speed (ms)" -> [w2050]
                tunnel: [w2054] -> w2036
                tunnel: [w2053] -> w2035
                tunnel: [w2052] -> w2034
                tunnel: [w2051] -> w2033
                tunnel: [w2044] -> w2022
                tunnel: [w2043] -> w2008
                tunnel: [w2042] -> w2005
                tunnel: [w2041] -> w1995
                tunnel: [w2113] -> w2032
                tunnel: w2036 -> [w2113]
                tunnel: [w2112] -> w2031
                tunnel: w2035 -> [w2112]
                tunnel: [w2111] -> w2030
                tunnel: w2034 -> [w2111]
                tunnel: [w2110] -> w2029
                tunnel: w2033 -> [w2110]
                tunnel: w2022 -> [w2109]
                tunnel: [w2109] -> w2021
                tunnel: w2008 -> [w2108]
                tunnel: [w2107] -> w2006
                tunnel: w2005 -> [w2107]
                tunnel: [w2106] -> w1996
                tunnel: w1995 -> [w2106]
                tunnel: w2032 -> [w2125]
                tunnel: w2031 -> [w2124]
                tunnel: w2030 -> [w2123]
                tunnel: w2029 -> [w2122]
                tunnel: w2019 -> [w2121]
                tunnel: [w2120] -> w2038
                tunnel: [w2119] -> w2037
                tunnel: w2021 -> [w2118]
                tunnel: [w2117] -> w2007
                tunnel: w2006 -> [w2116]
                tunnel: [w2115] -> w1994
                tunnel: w1996 -> [w2115]
                frame #0 {
                  n1314 = local read "Mean force (pN)"() -> (w2049:dbl)
                  n1315 = local read "Cutoff force (pN)"() -> (w2048:dbl)
                  n1316 = Less Or Equal?(x=w2049, y=w2048) -> (x <= y?=w2046:bool)
                  n1317 = And(x="Fish", y=w2046) -> (x .and. y?=w2047:bool)
                  n1318 = case shown="True" w2047 {
                    selector: w2047 -> [w2063 _]
                    tunnel: w2060 -> [w2066 w2083]
                    tunnel: w2059 -> [_ w2082]
                    tunnel: w2058 -> [w2068 w2081]
                    tunnel: w2057 -> [w2067 w2080]
                    tunnel: w2056 -> [w2065 w2079]
                    tunnel: w2055 -> [w2064 w2078]
                    tunnel: [w2068 w2077] -> w2054
                    tunnel: [w2067 w2076] -> w2053
                    tunnel: [w2066 w2075] -> w2052
                    tunnel: [w2064 w2074] -> w2042
                    tunnel: [w2065 w2073] -> w2051
                    tunnel: w2050 -> [_ w2072]
                    tunnel: [w2063 w2071] -> w2044
                    tunnel: [FALSE w2070] -> w2043
                    tunnel: [FALSE w2069] -> w2041
                    frame False {
                    }
                    frame True {
                      n1319 = while {
                        tunnel: w2083 -> [w2095]
                        tunnel: w2082 -> [w2094]
                        tunnel: w2081 -> [w2102]
                        tunnel: w2080 -> [w2101]
                        tunnel: w2079 -> [w2093]
                        tunnel: w2078 -> [w2099]
                        tunnel: [w2097] -> w2077
                        tunnel: [w2096] -> w2076
                        tunnel: [w2095] -> w2075
                        tunnel: [w2094] -> w2074
                        tunnel: [w2093] -> w2073
                        tunnel: w2072 -> [w2092]
                        tunnel: [w2085] -> w2071
                        tunnel: [w2085] -> w2070
                        tunnel: [w2084] -> w2069
                        i -> [w2091]
                        stop <- w2088 stop-if-true
                        # "top: x"
                        # "x direction"
                        # "y direction"
                        n1320 = Multiply(x=w2093, y=w2091) -> (x*y=w2100:dbl)
                        n1321 = local read "Cutoff force (pN)"() -> (w2086:dbl)
                        n1322 = local read "Mean force (pN)"() -> (w2087:dbl)
                        n1323 = Subtract(x=w2099, y=w2100) -> (x-y=w2098:dbl)
                        n1324 = Build Array(w2094, w2098) -> (w2105:dbl[])
                        n1325 = Build Array(w2098, w2094) -> (w2104:dbl[])
                        n1326 = Greater Or Equal?(x=w2091, y=w2092) -> (x >= y?=w2085:bool)
                        n1327 = Select(t=w2105, s=w2095, f=w2104) -> (s? t:f=w2103:dbl[])
                        n1328 = Greater?(x=w2087, y=w2086) -> (0:w2084:bool)
                        n1329 = local read "Fish"() -> (w2089:bool)
                        n1330 = Not(x=w2089) -> (.not. x?=w2090:bool)
                        n1331 = call-poly <vilib>:"DAQmx Write.vi"("task/channels in"=w2102, "data"=w2103, "error in"=w2101) -> ("task out"=w2097:refnum<k21>, "error out"=w2096:errorcluster)  [unwired: 10 in, 1 out]
                        n1332 = Compound Arithmetic op=OR(w2085, w2090, w2084) -> (w2088:bool)
                      }
                    }
                  }
                }
                frame #1 {
                  n1333 = case shown="True" w2108 {
                    frame False {
                    }
                    frame True {
                      n1334 = Wait (ms)(milliseconds to wait="Wait (ms)") -> ()  [unwired: 1 out]
                    }
                  }
                }
                frame #2 {
                  n1335 = case shown="True" w2118 {
                    tunnel: w2125 -> [w2128 w2137]
                    tunnel: w2124 -> [w2127 w2136]
                    tunnel: w2123 -> [_ w2135]
                    tunnel: w2122 -> [_ w2134]
                    tunnel: w2121 -> [_ w2133]
                    tunnel: [w2128 w2132] -> w2120
                    tunnel: [w2127 w2131] -> w2119
                    tunnel: [FALSE w2130] -> w2117
                    tunnel: w2116 -> [_ w2129]
                    frame False {
                    }
                    frame True {
                      n1336 = while {
                        tunnel: w2137 -> [w2169]
                        tunnel: w2136 -> [w2168]
                        tunnel: w2135 -> [w2140]
                        tunnel: w2134 -> [w2166]
                        tunnel: w2133 -> [w2165]
                        tunnel: [w2163] -> w2132
                        tunnel: [w2162] -> w2131
                        tunnel: [w2147] -> w2130
                        tunnel: w2129 -> [w2138]
                        i -> [w2154]
                        stop <- w2159 stop-if-true
                        # "y direction"
                        # "If tether formed,\nimmediately change\nto new delta."
                        n1337 = local read "Conv Y (nm/V)"() -> (w2141:dbl)
                        n1338 = local read "Conv X (nm/V)"() -> (w2139:dbl)
                        n1339 = local read "Fixed Y"() -> (w2148:dbl)
                        n1340 = local read "Fixed X"() -> (w2153:dbl)
                        n1341 = Select(t=w2141, s=w2140, f=w2139) -> (s? t:f=w2142:dbl)
                        n1342 = local read "Cutoff force (pN)"() -> (w2155:dbl)
                        n1343 = Divide(x="Delta after tether", y=w2142) -> (x/y=w2143:dbl)
                        n1344 = Multiply(x=w2166, y=w2154) -> (x*y=w2167:dbl)
                        n1345 = local read "Mean force (pN)"() -> (w2156:dbl)
                        n1346 = Add(x=w2165, y=w2167) -> (x+y=w2150:dbl)
                        n1347 = Select(t=w2148, s=w2140, f=w2153) -> (s? t:f=w2152:dbl)
                        n1348 = Greater?(x=w2156, y=w2155) -> (0:w2147:bool)
                        n1349 = Add(x=w2152, y=w2143) -> (x+y=w2151:dbl)
                        n1350 = Select(t=w2151, s=w2147, f=w2150) -> (s? t:f=w2149:dbl)
                        n1351 = local read "Fish Speed (ms)"() -> (w2161:i32)
                        n1352 = Build Array(w2138, w2149) -> (w2164:dbl[])
                        n1353 = Build Array(w2149, w2138) -> (w2145:dbl[])
                        n1354 = Select(t=w2164, s=w2140, f=w2145) -> (s? t:f=w2144:dbl[])
                        n1355 = case shown="True" w2147 {
                          tunnel: w2143 -> [_ _]
                          tunnel: w2144 -> [_ w2171]
                          frame False {
                          }
                          frame True {
                            n1356 = Array To Cluster(array=w2171) -> (cluster=w2170:cluster{"[0]":dbl, "[1]":dbl})
                            n1357 = property on="Trap position (V)" class="Clust (strict)"("Val(Sgnl)"=w2170) -> ()  [unwired: 2 in, 2 out]
                          }
                        }
                        n1358 = local read "Fish"() -> (w2158:bool)
                        n1359 = Greater Or Equal?(x=w2154, y=w2161) -> (x >= y?=w2160:bool)
                        n1360 = Not(x=w2158) -> (.not. x?=w2157:bool)
                        n1361 = call-poly <vilib>:"DAQmx Write.vi"("task/channels in"=w2169, "data"=w2144, "error in"=w2168) -> ("task out"=w2163:refnum<k21>, "error out"=w2162:errorcluster)  [unwired: 10 in, 1 out]
                        n1362 = Compound Arithmetic op=OR(w2160, w2157, w2147) -> (w2159:bool)
                      }
                    }
                  }
                }
              }
              n1363 = Add(x=w2012, y=w2000) -> (x+y=w2019:dbl)
              n1364 = Decrement(x="# attempts") -> (x-1=w2027:dbl)
              n1365 = Greater Or Equal?(x=w2023, y=w2027) -> (x >= y?=w2026:bool)
              n1366 = local read "Mean force (pN)"() -> (w2025:dbl)
              n1367 = Greater?(x=w2025, y="Cutoff force (pN)") -> (0:w2020:bool)
              n1368 = Compound Arithmetic op=OR(w1994, w2007, w2020, w2026) -> (w1998:bool)
              n1369 = Or(x=w2007, y=w1994) -> (x .or. y?=w1997:bool)
              "Tether" <- w1997
              n1370 = case shown="True" w1997 {
                frame False {
                }
                frame True {
                  n1371 = call <vilib>:"Beep.vi"() -> ()  [unwired: 12 in]
                }
              }
              n1372 = node-c288() -> ()  [unwired: 1 in, 1 out]
              "Attempt #" <- w2023
            }
            n1373 = node-c288(w1970) -> ()  [unwired: 1 out]
            n1374 = flat-sequence {
              tunnel: w1960 -> [w1978]
              tunnel: [w1978] -> w1956
              tunnel: w1959 -> [w1975]
              tunnel: w1958 -> [w1974]
              tunnel: w1957 -> [w1972]
              tunnel: w1956 -> [w1980]
              tunnel: [w1980] -> w1955
              tunnel: w1955 -> [w1982]
              frame #0 {
                w1977 = T24 1 items=["no dialog", "OK message", "continue or stop message", "OK message + warnings", "continue/stop + warnings"] ("type of dialog (OK msg:1)")
                n1375 = call <vilib>:"DAQmx Clear Task.vi"("task in"=w1975, "error in"=w1974) -> ("error out"=w1976:errorcluster)  [unwired: 13 in]
                n1376 = Not(x=w1972) -> (.not. x?=w1973:bool)
                n1377 = local write "Fish"(w1973) -> ()
                n1378 = call <vilib>:"Simple Error Handler.vi"("type of dialog (OK msg:1)"=w1977, "error in (no error)"=w1976) -> ()  [unwired: 3 in, 5 out]
              }
              frame #1 {
                n1379 = Wait (ms)(milliseconds to wait=u32 500) -> ()  [unwired: 1 out]
              }
              frame #2 {
                n1380 = And(x=w1982, y="Raster after\n tether?") -> (x .and. y?=w1983:bool)
                n1381 = case shown="True" w1983 {
                  selector: w1983 -> [_ w1984]
                  frame False {
                  }
                  frame True {
                    n1382 = stacked-sequence {
                      tunnel: w1984 -> [_ _ _ _ w1993]
                      frame #0 {
                        n1383 = local read "Raster set"() -> (w1988:i32)
                        n1384 = property on="Inject Sample" class="Bool (strict)"("Val(Sgnl)"=FALSE ("Value (Signaling)")) -> ()  [unwired: 2 in, 2 out]
                        n1385 = Replace Array Subset(array=i32[] [0], new element=w1988, index=0) -> (w1985:i32[])
                        n1386 = property on="Scan Parameters" class="Arr (strict)"("Index Values"=w1985) -> ()  [unwired: 2 in, 2 out]
                      }
                      frame #1 {
                        n1387 = Wait (ms)(milliseconds to wait=u32 500) -> ()  [unwired: 1 out]
                      }
                      frame #2 {
                        n1388 = property on="Load param" class="Bool (strict)"("Val(Sgnl)"=TRUE ("Value (Signaling)")) -> ()  [unwired: 2 in, 2 out]
                      }
                      frame #3 {
                        n1389 = Wait (ms)(milliseconds to wait=u32 500) -> ()  [unwired: 1 out]
                      }
                      frame #4 {
                        n1390 = property on="Raster scan" class="Bool (strict)"("Val(Sgnl)"=w1993) -> ()  [unwired: 2 in, 2 out]
                      }
                    }
                  }
                }
              }
            }
          }
        }
      }
      event "Load param": Value Change {
        n1391 = event-data() -> ()  [unwired: 1 in, 6 out]
        n1392 = property on="Scan Parameters" class="Arr (strict)"() -> ("Index Values"=w2187:u32[])  [unwired: 2 in, 2 out]
        n1393 = Index Array(array=w2187, index=0) -> (element=w2184:u32)
        n1394 = Index Array(array="Scan Parameters", index=w2184) -> (element=w2183:T27)
        n1395 = Unbundle(w2183) -> ("Scan range 1"=w2181:dbl, "Step size 1"=w2180:dbl, "Scan speed 1"=w2178:i32, "# scans 2"=w2179:i32)  [unwired: 1 out]
        n1396 = property on="# scans" class="DigNum (strict)"("Val(Sgnl)"=w2179) -> ()  [unwired: 2 in, 2 out]
        n1397 = property on="Scan range (nm)" class="DigNum (strict)"("Val(Sgnl)"=w2181) -> ()  [unwired: 2 in, 2 out]
        n1398 = property on="Step size 1" class="DigNum (strict)"("Val(Sgnl)"=w2180) -> ()  [unwired: 2 in, 2 out]
        n1399 = property on="Scan speed (nm/s)" class="DigNum (strict)"("Val(Sgnl)"=w2178) -> ()  [unwired: 2 in, 2 out]
        n1400 = local write "Load param"(FALSE ("Load param")) -> ()
      }
      event "# scans", "Scan range (nm)", "Step size (nm)", "Scan speed (nm/s)": Value Change {
        n1401 = event-data() -> ()  [unwired: 1 in, 6 out]
        n1402 = local read "Pulling direction"() -> (w2218:bool)
        n1403 = Reciprocal(x="Scan speed (nm/s)") -> (1/x=w2210:dbl)
        n1404 = local read "Conv Y (nm/V)"() -> (w2216:dbl)
        n1405 = local read "Conv X (nm/V)"() -> (w2217:dbl)
        n1406 = Multiply(x="Step size (nm)", y=w2210) -> (x*y=w2208:dbl)
        n1407 = Divide(x="Scan range (nm)", y="Step size (nm)") -> (x/y=w2215:dbl)
        n1408 = Absolute Value(x=w2215) -> (abs(x)=w2214:dbl)
        n1409 = Multiply(x=w2208, y=1000.0) -> (x*y=w2195:dbl)
        n1410 = Select(t=w2216, s=w2218, f=w2217) -> (s? t:f=w2206:dbl)
        n1411 = Multiply(x="# scans", y=2) -> (x*y=w2194:i32)
        n1412 = To Unsigned Quad Integer(1:w2214) -> (0:w2204:u64)
        "Scan steps (mirror)" <- w2204
        n1413 = Divide(x="Scan range (nm)", y=w2206) -> (x/y=→"Scan range (V)":dbl)
        n1414 = Multiply(x=w2204, y=w2195) -> (x*y=w2203:dbl)
        n1415 = Divide(x="Step size (nm)", y=w2206) -> (x/y=→"Scan increment (V)":dbl)
        n1416 = Round Toward +Infinity(x=w2195) -> (ceil(x): smallest int >= x=w2192:dbl)
        "Time per step (ms)" <- w2192
        n1417 = local read "Data update period (s/set)"() -> (w2198:dbl)
        n1418 = Multiply(x=w2194, y=w2203) -> (x*y=w2201:dbl)
        n1419 = Divide(x=w2201, y=1000.0) -> (x/y=w2199:dbl)
        "Total raster time (s)" <- w2199
        n1420 = local read "Data update period (s/set)"() -> (w2190:dbl)
        n1421 = Divide(x=w2199, y=w2198) -> (x/y=w2197:dbl)
        n1422 = Round Toward -Infinity(1:w2197) -> (0:→"N sets to be saved":dbl)
        n1423 = Multiply(x=w2190, y=1000.0) -> (x*y=w2188:dbl)
        n1424 = Less?(x=w2192, y=w2188) -> (x < y?=w2191:bool)
        n1425 = case shown="True" w2191 {
          selector: w2191 -> [_ w2219]
          frame False {
          }
          frame True {
            n1426 = call "Display Message to User"("Enable"=w2219) -> ()  [unwired: 9 in, 2 out]
          }
        }
      }
      event "Pulling direction": Value Change {
        n1427 = event-data() -> ()  [unwired: 1 in, 6 out]
        n1428 = local read "Pulling direction"() -> (w2225:bool)
        n1429 = local read "Conv Y (nm/V)"() -> (w2227:dbl)
        n1430 = local read "Conv X (nm/V)"() -> (w2226:dbl)
        n1431 = local read "Scan range (nm)"() -> (w2224:dbl)
        n1432 = Select(t=w2227, s=w2225, f=w2226) -> (s? t:f=w2221:dbl)
        n1433 = local read "Step size (nm)"() -> (w2222:dbl)
        n1434 = case shown="False" w2225 {
          frame False {
            n1435 = local read "Fixed Y"() -> (w2230:dbl)
            n1436 = local read "Trap delta (nm)"() -> (w2235:dbl)
            n1437 = local read "Conv X (nm/V)"() -> (w2234:dbl)
            n1438 = local read "Fixed X"() -> (w2232:dbl)
            n1439 = Divide(x=w2235, y=w2234) -> (x/y=w2233:dbl)
            n1440 = Add(x=w2233, y=w2232) -> (x+y=w2231:dbl)
            n1441 = Build Array(w2231, w2230) -> (w2229:dbl[])
            n1442 = Array To Cluster(array=w2229) -> (cluster=w2228:cluster{"[0]":dbl, "[1]":dbl})
            n1443 = property on="Trap position (V)" class="Clust (strict)"("Val(Sgnl)"=w2228) -> ()  [unwired: 2 in, 2 out]
          }
          frame True {
            n1444 = local read "Trap delta (nm)"() -> (w2243:dbl)
            n1445 = local read "Conv Y (nm/V)"() -> (w2242:dbl)
            n1446 = local read "Fixed X"() -> (w2238:dbl)
            n1447 = local read "Fixed Y"() -> (w2240:dbl)
            n1448 = Divide(x=w2243, y=w2242) -> (x/y=w2241:dbl)
            n1449 = Add(x=w2241, y=w2240) -> (x+y=w2239:dbl)
            n1450 = Build Array(w2238, w2239) -> (w2237:dbl[])
            n1451 = Array To Cluster(array=w2237) -> (cluster=w2236:cluster{"[0]":dbl, "[1]":dbl})
            n1452 = property on="Trap position (V)" class="Clust (strict)"("Val(Sgnl)"=w2236) -> ()  [unwired: 2 in, 2 out]
          }
        }
        n1453 = Divide(x=w2224, y=w2221) -> (x/y=w2223:dbl)
        n1454 = Divide(x=w2222, y=w2221) -> (x/y=w2220:dbl)
        n1455 = local write "Scan range (V)"(w2223) -> ()
        n1456 = local write "Scan increment (V)"(w2220) -> ()
      }
      event "Averaging Number": Value Change {
        n1457 = event-data() -> ()  [unwired: 1 in, 6 out]
        n1458 = local read "# Samples/channel (in)"() -> (w2247:i32)
        n1459 = local read "Averaging Number"() -> (w2245:i32)
        n1460 = Quotient & Remainder(x=w2247, y=w2245) -> (floor(x/y)=w2246:i32)  [unwired: 1 out]
        n1461 = Multiply(x=w2246, y=w2245) -> (x*y=w2244:i32)
        n1462 = local write "# Samples/channel (in)"(w2244) -> ()
      }
    }
    n1463 = node-c288() -> ()  [unwired: 1 in, 1 out]
  }
  n1464 = VISA Close(VISA resource name=w27) -> (error out=w105:errorcluster)  [unwired: 1 in]
  n1465 = call <vilib>:"Simple Error Handler.vi"("error in (no error)"=w105) -> ()  [unwired: 4 in, 5 out]
  n1466 = disable-structure shown="Enabled" {
    frame Disabled {
      n1467 = node-c288(2 ("Processor")) -> (w2253:T13)  [unwired: 3 in]
      n1468 = timed-loop "Pump Control" {
        timing: w2253 -> [_]
        timing-out: [_] -> w2252
        tunnel: refnum<visa-resource-name> "COM6" ("VISA resource name") -> [w2255]
        stop <- w2254 stop-if-true
        n1469 = node-c288() -> ()  [unwired: 1 in, 1 out]
        n1470 = event shown="[4] \"Inject Pump 1\": Value Change" {
          selector: _ -> [_ _ _ _ _ _ _ _ _]
          dyn-events: _ -> [_ _ _ _ _ _ _ _ _]
          timeout: _ -> [_ _ _ _ _ _ _ _ _]
          tunnel: w2255 -> [w2263 w2359 _ w2435 w2563 w2706 w2751 w2809 w2868]
          tunnel: [_ _ w2434 _ _ _ _ _ _] -> w2254
          event "Flush Pump 1": Value Change {
            w2264 = "\r"
            n1471 = event-data() -> ()  [unwired: 1 in, 5 out]
            n1472 = call-poly "VISA Configure Serial Port"("VISA resource name"=w2263) -> ("VISA resource name out"=w2277:refnum<visa-resource-name>, "error out"=w2278:errorcluster)  [unwired: 13 in]
            n1473 = local read "Write Wait"() -> (w2256:i32)
            n1474 = Concatenate Strings("enter pump1", w2264) -> (w2265:string)
            n1475 = flat-sequence {
              tunnel: w2278 -> [w2297]
              tunnel: w2277 -> [w2299]
              tunnel: [w2298] -> w2294
              tunnel: [w2296] -> w2293
              tunnel: w2265 -> [w2295]
              tunnel: w2294 -> [w2302]
              tunnel: [w2302] -> w2292
              tunnel: w2293 -> [w2301]
              tunnel: [w2301] -> w2291
              tunnel: w2256 -> [w2300]
              tunnel: [w2307] -> w2290
              tunnel: w2270 -> [w2306]
              tunnel: [w2303] -> w2289
              tunnel: w2292 -> [w2305]
              tunnel: w2291 -> [w2304]
              tunnel: w2290 -> [w2310]
              tunnel: [w2310] -> w2288
              tunnel: [w2309] -> w2287
              tunnel: w2289 -> [w2309]
              tunnel: w2256 -> [w2308]
              tunnel: w2288 -> [w2315]
              tunnel: [w2314] -> w2286
              tunnel: w2273 -> [w2313]
              tunnel: w2287 -> [w2312]
              tunnel: [w2311] -> w2285
              tunnel: w2286 -> [w2318]
              tunnel: [w2318] -> w2284
              tunnel: [w2317] -> w2283
              tunnel: w2285 -> [w2317]
              tunnel: w2256 -> [w2316]
              tunnel: w2284 -> [w2323]
              tunnel: [w2322] -> w2282
              tunnel: w2276 -> [w2321]
              tunnel: w2283 -> [w2320]
              tunnel: [w2319] -> w2281
              tunnel: [w2326] -> w2280
              tunnel: w2282 -> [w2326]
              tunnel: [w2325] -> w2279
              tunnel: w2281 -> [w2325]
              tunnel: w2256 -> [w2324]
              tunnel: w2280 -> [w2331]
              tunnel: w2279 -> [w2328]
              tunnel: [w2330] -> w2259
              tunnel: [w2329] -> w2257
              tunnel: [w2336] -> w2260
              tunnel: w2259 -> [w2336]
              tunnel: [w2335] -> w2258
              tunnel: w2257 -> [w2335]
              tunnel: w2256 -> [w2334]
              tunnel: w2260 -> [w2338]
              tunnel: w2258 -> [w2337]
              frame #0 {
                n1476 = VISA Write(VISA resource name=w2299, write buffer=w2295, error in (no error)=w2297) -> (VISA resource name out=w2298:refnum<visa-resource-name>, error out=w2296:errorcluster)  [unwired: 1 out]
              }
              frame #1 {
                n1477 = Wait (ms)(milliseconds to wait=w2300) -> ()  [unwired: 1 out]
              }
              frame #2 {
                n1478 = VISA Write(VISA resource name=w2305, write buffer=w2306, error in (no error)=w2304) -> (VISA resource name out=w2307:refnum<visa-resource-name>, error out=w2303:errorcluster)  [unwired: 1 out]
              }
              frame #3 {
                n1479 = Wait (ms)(milliseconds to wait=w2308) -> ()  [unwired: 1 out]
              }
              frame #4 {
                n1480 = VISA Write(VISA resource name=w2315, write buffer=w2313, error in (no error)=w2312) -> (VISA resource name out=w2314:refnum<visa-resource-name>, error out=w2311:errorcluster)  [unwired: 1 out]
              }
              frame #5 {
                n1481 = Wait (ms)(milliseconds to wait=w2316) -> ()  [unwired: 1 out]
              }
              frame #6 {
                n1482 = VISA Write(VISA resource name=w2323, write buffer=w2321, error in (no error)=w2320) -> (VISA resource name out=w2322:refnum<visa-resource-name>, error out=w2319:errorcluster)  [unwired: 1 out]
              }
              frame #7 {
                n1483 = Wait (ms)(milliseconds to wait=w2324) -> ()  [unwired: 1 out]
              }
              frame #8 {
                n1484 = Concatenate Strings("start ", "\r") -> (w2327:string)
                n1485 = VISA Write(VISA resource name=w2331, write buffer=w2327, error in (no error)=w2328) -> (VISA resource name out=w2330:refnum<visa-resource-name>, error out=w2329:errorcluster)  [unwired: 1 out]
              }
              frame #9 {
                n1486 = Wait (ms)(milliseconds to wait=w2334) -> ()  [unwired: 1 out]
              }
              frame #10 {
                n1487 = local write "Flush Pump 1"(FALSE ("Flush Pump 1")) -> ()
                n1488 = Concatenate Strings("enter main ", "\r") -> (w2342:string)
                n1489 = VISA Write(VISA resource name=w2338, write buffer=w2342, error in (no error)=w2337) -> (VISA resource name out=w2341:refnum<visa-resource-name>, error out=w2340:errorcluster)  [unwired: 1 out]
                n1490 = VISA Close(VISA resource name=w2341, error in (no error)=w2340) -> ()  [unwired: 1 out]
              }
            }
            n1491 = Concatenate Strings("set units 4 ", w2264) -> (w2270:string)
            n1492 = Multiply(x="Flush\nRate (ul/min)", y=60) -> (x*y=w2268:dbl)
            n1493 = Number To Decimal String(number=w2268) -> (decimal integer string=w2271:string)  [unwired: 1 in]
            n1494 = Concatenate Strings("set rate ", w2271, w2264) -> (w2273:string)
            n1495 = Number To Decimal String(number="Flush\nVolume (ul)") -> (decimal integer string=w2275:string)  [unwired: 1 in]
            n1496 = Concatenate Strings("set volume ", w2275, w2264) -> (w2276:string)
          }
          event "Flush Pump 2": Value Change {
            w2350 = "\r"
            n1497 = event-data() -> ()  [unwired: 1 in, 5 out]
            n1498 = call-poly "VISA Configure Serial Port"("VISA resource name"=w2359) -> ("VISA resource name out"=w2370:refnum<visa-resource-name>, "error out"=w2371:errorcluster)  [unwired: 13 in]
            n1499 = local read "Write Wait"() -> (w2345:i32)
            n1500 = Concatenate Strings("enter pump2", w2350) -> (w2351:string)
            n1501 = flat-sequence {
              tunnel: w2371 -> [w2386]
              tunnel: w2370 -> [w2388]
              tunnel: [w2387] -> w2356
              tunnel: [w2385] -> w2354
              tunnel: w2351 -> [w2384]
              tunnel: w2356 -> [w2391]
              tunnel: [w2391] -> w2355
              tunnel: w2354 -> [w2390]
              tunnel: [w2390] -> w2353
              tunnel: w2345 -> [w2389]
              tunnel: [w2396] -> w2383
              tunnel: w2363 -> [w2395]
              tunnel: [w2392] -> w2382
              tunnel: w2355 -> [w2394]
              tunnel: w2353 -> [w2393]
              tunnel: w2383 -> [w2399]
              tunnel: [w2399] -> w2381
              tunnel: [w2398] -> w2380
              tunnel: w2382 -> [w2398]
              tunnel: w2345 -> [w2397]
              tunnel: w2381 -> [w2404]
              tunnel: [w2403] -> w2379
              tunnel: w2366 -> [w2402]
              tunnel: w2380 -> [w2401]
              tunnel: [w2400] -> w2378
              tunnel: w2379 -> [w2407]
              tunnel: [w2407] -> w2377
              tunnel: [w2406] -> w2376
              tunnel: w2378 -> [w2406]
              tunnel: w2345 -> [w2405]
              tunnel: w2377 -> [w2412]
              tunnel: [w2411] -> w2375
              tunnel: w2369 -> [w2410]
              tunnel: w2376 -> [w2409]
              tunnel: [w2408] -> w2374
              tunnel: [w2415] -> w2373
              tunnel: w2375 -> [w2415]
              tunnel: [w2414] -> w2372
              tunnel: w2374 -> [w2414]
              tunnel: w2345 -> [w2413]
              tunnel: w2373 -> [w2422]
              tunnel: w2372 -> [w2421]
              tunnel: [w2417] -> w2349
              tunnel: [w2416] -> w2347
              tunnel: w2349 -> [w2425]
              tunnel: [w2425] -> w2348
              tunnel: w2347 -> [w2424]
              tunnel: [w2424] -> w2346
              tunnel: w2345 -> [w2423]
              tunnel: w2348 -> [w2429]
              tunnel: w2346 -> [w2428]
              frame #0 {
                n1502 = VISA Write(VISA resource name=w2388, write buffer=w2384, error in (no error)=w2386) -> (VISA resource name out=w2387:refnum<visa-resource-name>, error out=w2385:errorcluster)  [unwired: 1 out]
              }
              frame #1 {
                n1503 = Wait (ms)(milliseconds to wait=w2389) -> ()  [unwired: 1 out]
              }
              frame #2 {
                n1504 = VISA Write(VISA resource name=w2394, write buffer=w2395, error in (no error)=w2393) -> (VISA resource name out=w2396:refnum<visa-resource-name>, error out=w2392:errorcluster)  [unwired: 1 out]
              }
              frame #3 {
                n1505 = Wait (ms)(milliseconds to wait=w2397) -> ()  [unwired: 1 out]
              }
              frame #4 {
                n1506 = VISA Write(VISA resource name=w2404, write buffer=w2402, error in (no error)=w2401) -> (VISA resource name out=w2403:refnum<visa-resource-name>, error out=w2400:errorcluster)  [unwired: 1 out]
              }
              frame #5 {
                n1507 = Wait (ms)(milliseconds to wait=w2405) -> ()  [unwired: 1 out]
              }
              frame #6 {
                n1508 = VISA Write(VISA resource name=w2412, write buffer=w2410, error in (no error)=w2409) -> (VISA resource name out=w2411:refnum<visa-resource-name>, error out=w2408:errorcluster)  [unwired: 1 out]
              }
              frame #7 {
                n1509 = Wait (ms)(milliseconds to wait=w2413) -> ()  [unwired: 1 out]
              }
              frame #8 {
                n1510 = Concatenate Strings("start ", "\r") -> (w2420:string)
                n1511 = VISA Write(VISA resource name=w2422, write buffer=w2420, error in (no error)=w2421) -> (VISA resource name out=w2417:refnum<visa-resource-name>, error out=w2416:errorcluster)  [unwired: 1 out]
              }
              frame #9 {
                n1512 = Wait (ms)(milliseconds to wait=w2423) -> ()  [unwired: 1 out]
              }
              frame #10 {
                n1513 = local write "Flush Pump 2"(FALSE ("Flush Pump 1")) -> ()
                n1514 = Concatenate Strings("enter main ", "\r") -> (w2430:string)
                n1515 = VISA Write(VISA resource name=w2429, write buffer=w2430, error in (no error)=w2428) -> (VISA resource name out=w2427:refnum<visa-resource-name>, error out=w2426:errorcluster)  [unwired: 1 out]
                n1516 = VISA Close(VISA resource name=w2427, error in (no error)=w2426) -> ()  [unwired: 1 out]
              }
            }
            n1517 = Concatenate Strings("set units 4 ", w2350) -> (w2363:string)
            n1518 = Multiply(x="Flush \nRate (ul/min)  2", y=60) -> (x*y=w2361:dbl)
            n1519 = Number To Decimal String(number=w2361) -> (decimal integer string=w2364:string)  [unwired: 1 in]
            n1520 = Concatenate Strings("set rate ", w2364, w2350) -> (w2366:string)
            n1521 = Number To Decimal String(number="Flush\nVolume (ul)  2") -> (decimal integer string=w2368:string)  [unwired: 1 in]
            n1522 = Concatenate Strings("set volume ", w2368, w2350) -> (w2369:string)
          }
          event "Stop": Value Change {
            n1523 = event-data() -> ()  [unwired: 1 in, 5 out]
            n1524 = local read "Stop"() -> (w2434:bool)
          }
          event "Inject Pump 2": Value Change {
            n1525 = event-data() -> ()  [unwired: 1 in, 5 out]
            n1526 = case shown="True" "Inject Pump 2" {
              tunnel: w2435 -> [w2438 w2480]
              frame False {
                n1527 = local read "Write Wait"() -> (w2437:i32)
                n1528 = call-poly "VISA Configure Serial Port"("VISA resource name"=w2438) -> ("VISA resource name out"=w2442:refnum<visa-resource-name>, "error out"=w2443:errorcluster)  [unwired: 13 in]
                n1529 = Concatenate Strings("enter pump2", "\r") -> (w2440:string)
                n1530 = flat-sequence {
                  tunnel: w2443 -> [w2454]
                  tunnel: w2442 -> [w2456]
                  tunnel: [w2455] -> w2451
                  tunnel: [w2453] -> w2450
                  tunnel: w2440 -> [w2452]
                  tunnel: w2451 -> [w2459]
                  tunnel: w2450 -> [w2458]
                  tunnel: [w2459] -> w2449
                  tunnel: [w2458] -> w2448
                  tunnel: w2437 -> [w2457]
                  tunnel: [w2463] -> w2447
                  tunnel: [w2462] -> w2446
                  tunnel: w2449 -> [w2461]
                  tunnel: w2448 -> [w2460]
                  tunnel: w2447 -> [w2469]
                  tunnel: [w2469] -> w2445
                  tunnel: w2446 -> [w2468]
                  tunnel: [w2468] -> w2444
                  tunnel: w2437 -> [w2467]
                  tunnel: w2445 -> [w2473]
                  tunnel: w2444 -> [w2472]
                  frame #0 {
                    n1531 = VISA Write(VISA resource name=w2456, write buffer=w2452, error in (no error)=w2454) -> (VISA resource name out=w2455:refnum<visa-resource-name>, error out=w2453:errorcluster)  [unwired: 1 out]
                  }
                  frame #1 {
                    n1532 = Wait (ms)(milliseconds to wait=w2457) -> ()  [unwired: 1 out]
                  }
                  frame #2 {
                    n1533 = Concatenate Strings("stop ", "\r") -> (w2466:string)
                    n1534 = VISA Write(VISA resource name=w2461, write buffer=w2466, error in (no error)=w2460) -> (VISA resource name out=w2463:refnum<visa-resource-name>, error out=w2462:errorcluster)  [unwired: 1 out]
                  }
                  frame #3 {
                    n1535 = Wait (ms)(milliseconds to wait=w2467) -> ()  [unwired: 1 out]
                  }
                  frame #4 {
                    n1536 = Concatenate Strings("enter main ", "\r") -> (w2474:string)
                    n1537 = VISA Write(VISA resource name=w2473, write buffer=w2474, error in (no error)=w2472) -> (VISA resource name out=w2471:refnum<visa-resource-name>, error out=w2470:errorcluster)  [unwired: 1 out]
                    n1538 = VISA Close(VISA resource name=w2471, error in (no error)=w2470) -> ()  [unwired: 1 out]
                  }
                }
              }
              frame True {
                w2493 = "\r"
                n1539 = call-poly "VISA Configure Serial Port"("VISA resource name"=w2480) -> ("VISA resource name out"=w2482:refnum<visa-resource-name>, "error out"=w2481:errorcluster)  [unwired: 13 in]
                n1540 = local read "Write Wait"() -> (w2477:i32)
                n1541 = Concatenate Strings("enter pump2", w2493) -> (w2492:string)
                n1542 = flat-sequence {
                  tunnel: w2481 -> [w2516]
                  tunnel: w2482 -> [w2518]
                  tunnel: [w2517] -> w2513
                  tunnel: [w2515] -> w2512
                  tunnel: w2492 -> [w2514]
                  tunnel: w2513 -> [w2521]
                  tunnel: [w2521] -> w2511
                  tunnel: w2512 -> [w2520]
                  tunnel: [w2520] -> w2510
                  tunnel: w2477 -> [w2519]
                  tunnel: [w2526] -> w2509
                  tunnel: w2489 -> [w2525]
                  tunnel: [w2522] -> w2508
                  tunnel: w2511 -> [w2524]
                  tunnel: w2510 -> [w2523]
                  tunnel: w2509 -> [w2529]
                  tunnel: [w2529] -> w2507
                  tunnel: [w2528] -> w2506
                  tunnel: w2508 -> [w2528]
                  tunnel: w2477 -> [w2527]
                  tunnel: w2507 -> [w2534]
                  tunnel: [w2533] -> w2505
                  tunnel: w2486 -> [w2532]
                  tunnel: w2506 -> [w2531]
                  tunnel: [w2530] -> w2504
                  tunnel: w2505 -> [w2537]
                  tunnel: [w2537] -> w2503
                  tunnel: [w2536] -> w2502
                  tunnel: w2504 -> [w2536]
                  tunnel: w2477 -> [w2535]
                  tunnel: w2503 -> [w2542]
                  tunnel: [w2541] -> w2501
                  tunnel: w2483 -> [w2540]
                  tunnel: w2502 -> [w2539]
                  tunnel: [w2538] -> w2500
                  tunnel: [w2545] -> w2499
                  tunnel: w2501 -> [w2545]
                  tunnel: [w2544] -> w2498
                  tunnel: w2500 -> [w2544]
                  tunnel: w2477 -> [w2543]
                  tunnel: w2499 -> [w2552]
                  tunnel: w2498 -> [w2551]
                  tunnel: [w2547] -> w2497
                  tunnel: [w2546] -> w2496
                  tunnel: w2497 -> [w2555]
                  tunnel: [w2555] -> w2495
                  tunnel: w2496 -> [w2554]
                  tunnel: [w2554] -> w2494
                  tunnel: w2477 -> [w2553]
                  tunnel: w2495 -> [w2559]
                  tunnel: w2494 -> [w2558]
                  frame #0 {
                    n1543 = VISA Write(VISA resource name=w2518, write buffer=w2514, error in (no error)=w2516) -> (VISA resource name out=w2517:refnum<visa-resource-name>, error out=w2515:errorcluster)  [unwired: 1 out]
                  }
                  frame #1 {
                    n1544 = Wait (ms)(milliseconds to wait=w2519) -> ()  [unwired: 1 out]
                  }
                  frame #2 {
                    n1545 = VISA Write(VISA resource name=w2524, write buffer=w2525, error in (no error)=w2523) -> (VISA resource name out=w2526:refnum<visa-resource-name>, error out=w2522:errorcluster)  [unwired: 1 out]
                  }
                  frame #3 {
                    n1546 = Wait (ms)(milliseconds to wait=w2527) -> ()  [unwired: 1 out]
                  }
                  frame #4 {
                    n1547 = VISA Write(VISA resource name=w2534, write buffer=w2532, error in (no error)=w2531) -> (VISA resource name out=w2533:refnum<visa-resource-name>, error out=w2530:errorcluster)  [unwired: 1 out]
                  }
                  frame #5 {
                    n1548 = Wait (ms)(milliseconds to wait=w2535) -> ()  [unwired: 1 out]
                  }
                  frame #6 {
                    n1549 = VISA Write(VISA resource name=w2542, write buffer=w2540, error in (no error)=w2539) -> (VISA resource name out=w2541:refnum<visa-resource-name>, error out=w2538:errorcluster)  [unwired: 1 out]
                  }
                  frame #7 {
                    n1550 = Wait (ms)(milliseconds to wait=w2543) -> ()  [unwired: 1 out]
                  }
                  frame #8 {
                    n1551 = Concatenate Strings("start ", "\r") -> (w2550:string)
                    n1552 = VISA Write(VISA resource name=w2552, write buffer=w2550, error in (no error)=w2551) -> (VISA resource name out=w2547:refnum<visa-resource-name>, error out=w2546:errorcluster)  [unwired: 1 out]
                  }
                  frame #9 {
                    n1553 = Wait (ms)(milliseconds to wait=w2553) -> ()  [unwired: 1 out]
                  }
                  frame #10 {
                    n1554 = Concatenate Strings("enter main ", "\r") -> (w2560:string)
                    n1555 = VISA Write(VISA resource name=w2559, write buffer=w2560, error in (no error)=w2558) -> (VISA resource name out=w2557:refnum<visa-resource-name>, error out=w2556:errorcluster)  [unwired: 1 out]
                    n1556 = VISA Close(VISA resource name=w2557, error in (no error)=w2556) -> ()  [unwired: 1 out]
                  }
                }
                n1557 = local read "Normal \nRate (ul/hr)  2"() -> (w2478:dbl)
                n1558 = Concatenate Strings("set units 4 ", w2493) -> (w2489:string)
                n1559 = local read "Normal \nVolume (ul) 2"() -> (w2479:dbl)
                n1560 = Number To Decimal String(number=w2478) -> (decimal integer string=w2488:string)  [unwired: 1 in]
                n1561 = Concatenate Strings("set rate ", w2488, w2493) -> (w2486:string)
                n1562 = Number To Decimal String(number=w2479) -> (decimal integer string=w2484:string)  [unwired: 1 in]
                n1563 = Concatenate Strings("set volume ", w2484, w2493) -> (w2483:string)
              }
            }
          }
          event "Inject Pump 1": Value Change {
            n1564 = event-data() -> ()  [unwired: 1 in, 5 out]
            n1565 = case shown="True" "Inject Pump 1" {
              tunnel: w2563 -> [w2566 w2608]
              frame False {
                n1566 = local read "Write Wait"() -> (w2565:i32)
                n1567 = call-poly "VISA Configure Serial Port"("VISA resource name"=w2566) -> ("VISA resource name out"=w2570:refnum<visa-resource-name>, "error out"=w2571:errorcluster)  [unwired: 13 in]
                n1568 = Concatenate Strings("enter pump1", "\r") -> (w2568:string)
                n1569 = flat-sequence {
                  tunnel: w2571 -> [w2582]
                  tunnel: w2570 -> [w2584]
                  tunnel: [w2583] -> w2579
                  tunnel: [w2581] -> w2578
                  tunnel: w2568 -> [w2580]
                  tunnel: w2579 -> [w2587]
                  tunnel: w2578 -> [w2586]
                  tunnel: [w2587] -> w2577
                  tunnel: [w2586] -> w2576
                  tunnel: w2565 -> [w2585]
                  tunnel: [w2591] -> w2575
                  tunnel: [w2590] -> w2574
                  tunnel: w2577 -> [w2589]
                  tunnel: w2576 -> [w2588]
                  tunnel: w2575 -> [w2597]
                  tunnel: [w2597] -> w2573
                  tunnel: w2574 -> [w2596]
                  tunnel: [w2596] -> w2572
                  tunnel: w2565 -> [w2595]
                  tunnel: w2573 -> [w2601]
                  tunnel: w2572 -> [w2600]
                  frame #0 {
                    n1570 = VISA Write(VISA resource name=w2584, write buffer=w2580, error in (no error)=w2582) -> (VISA resource name out=w2583:refnum<visa-resource-name>, error out=w2581:errorcluster)  [unwired: 1 out]
                  }
                  frame #1 {
                    n1571 = Wait (ms)(milliseconds to wait=w2585) -> ()  [unwired: 1 out]
                  }
                  frame #2 {
                    n1572 = Concatenate Strings("stop ", "\r") -> (w2594:string)
                    n1573 = VISA Write(VISA resource name=w2589, write buffer=w2594, error in (no error)=w2588) -> (VISA resource name out=w2591:refnum<visa-resource-name>, error out=w2590:errorcluster)  [unwired: 1 out]
                  }
                  frame #3 {
                    n1574 = Wait (ms)(milliseconds to wait=w2595) -> ()  [unwired: 1 out]
                  }
                  frame #4 {
                    n1575 = Concatenate Strings("enter main ", "\r") -> (w2602:string)
                    n1576 = VISA Write(VISA resource name=w2601, write buffer=w2602, error in (no error)=w2600) -> (VISA resource name out=w2599:refnum<visa-resource-name>, error out=w2598:errorcluster)  [unwired: 1 out]
                    n1577 = VISA Close(VISA resource name=w2599, error in (no error)=w2598) -> ()  [unwired: 1 out]
                  }
                }
              }
              frame True {
                w2621 = "\r"
                n1578 = call-poly "VISA Configure Serial Port"("VISA resource name"=w2608) -> ("VISA resource name out"=w2610:refnum<visa-resource-name>, "error out"=w2609:errorcluster)  [unwired: 13 in]
                n1579 = local read "Write Wait"() -> (w2605:i32)
                n1580 = flat-sequence {
                  tunnel: w2609 -> [w2644]
                  tunnel: w2610 -> [w2646]
                  tunnel: [w2645] -> w2641
                  tunnel: [w2643] -> w2640
                  tunnel: w2620 -> [w2642]
                  tunnel: w2641 -> [w2649]
                  tunnel: [w2649] -> w2639
                  tunnel: w2640 -> [w2648]
                  tunnel: [w2648] -> w2638
                  tunnel: w2605 -> [w2647]
                  tunnel: [w2654] -> w2637
                  tunnel: w2617 -> [w2653]
                  tunnel: [w2650] -> w2636
                  tunnel: w2639 -> [w2652]
                  tunnel: w2638 -> [w2651]
                  tunnel: w2637 -> [w2657]
                  tunnel: [w2657] -> w2635
                  tunnel: [w2656] -> w2634
                  tunnel: w2636 -> [w2656]
                  tunnel: w2605 -> [w2655]
                  tunnel: w2635 -> [w2662]
                  tunnel: [w2661] -> w2633
                  tunnel: w2614 -> [w2660]
                  tunnel: w2634 -> [w2659]
                  tunnel: [w2658] -> w2632
                  tunnel: w2633 -> [w2665]
                  tunnel: [w2665] -> w2631
                  tunnel: [w2664] -> w2630
                  tunnel: w2632 -> [w2664]
                  tunnel: w2605 -> [w2663]
                  tunnel: w2631 -> [w2670]
                  tunnel: [w2669] -> w2629
                  tunnel: w2611 -> [w2668]
                  tunnel: w2630 -> [w2667]
                  tunnel: [w2666] -> w2628
                  tunnel: [w2673] -> w2627
                  tunnel: w2629 -> [w2673]
                  tunnel: [w2672] -> w2626
                  tunnel: w2628 -> [w2672]
                  tunnel: w2605 -> [w2671]
                  tunnel: w2627 -> [w2680]
                  tunnel: w2626 -> [w2679]
                  tunnel: [w2675] -> w2625
                  tunnel: [w2674] -> w2624
                  tunnel: w2625 -> [w2683]
                  tunnel: [w2683] -> w2623
                  tunnel: w2624 -> [w2682]
                  tunnel: [w2682] -> w2622
                  tunnel: w2605 -> [w2681]
                  tunnel: w2623 -> [w2687]
                  tunnel: w2622 -> [w2686]
                  frame #0 {
                    n1581 = VISA Write(VISA resource name=w2646, write buffer=w2642, error in (no error)=w2644) -> (VISA resource name out=w2645:refnum<visa-resource-name>, error out=w2643:errorcluster)  [unwired: 1 out]
                  }
                  frame #1 {
                    n1582 = Wait (ms)(milliseconds to wait=w2647) -> ()  [unwired: 1 out]
                  }
                  frame #2 {
                    n1583 = VISA Write(VISA resource name=w2652, write buffer=w2653, error in (no error)=w2651) -> (VISA resource name out=w2654:refnum<visa-resource-name>, error out=w2650:errorcluster)  [unwired: 1 out]
                  }
                  frame #3 {
                    n1584 = Wait (ms)(milliseconds to wait=w2655) -> ()  [unwired: 1 out]
                  }
                  frame #4 {
                    n1585 = VISA Write(VISA resource name=w2662, write buffer=w2660, error in (no error)=w2659) -> (VISA resource name out=w2661:refnum<visa-resource-name>, error out=w2658:errorcluster)  [unwired: 1 out]
                  }
                  frame #5 {
                    n1586 = Wait (ms)(milliseconds to wait=w2663) -> ()  [unwired: 1 out]
                  }
                  frame #6 {
                    n1587 = VISA Write(VISA resource name=w2670, write buffer=w2668, error in (no error)=w2667) -> (VISA resource name out=w2669:refnum<visa-resource-name>, error out=w2666:errorcluster)  [unwired: 1 out]
                  }
                  frame #7 {
                    n1588 = Wait (ms)(milliseconds to wait=w2671) -> ()  [unwired: 1 out]
                  }
                  frame #8 {
                    n1589 = Concatenate Strings("start ", "\r") -> (w2678:string)
                    n1590 = VISA Write(VISA resource name=w2680, write buffer=w2678, error in (no error)=w2679) -> (VISA resource name out=w2675:refnum<visa-resource-name>, error out=w2674:errorcluster)  [unwired: 1 out]
                  }
                  frame #9 {
                    n1591 = Wait (ms)(milliseconds to wait=w2681) -> ()  [unwired: 1 out]
                  }
                  frame #10 {
                    n1592 = Concatenate Strings("enter main ", "\r") -> (w2688:string)
                    n1593 = VISA Write(VISA resource name=w2687, write buffer=w2688, error in (no error)=w2686) -> (VISA resource name out=w2685:refnum<visa-resource-name>, error out=w2684:errorcluster)  [unwired: 1 out]
                    n1594 = VISA Close(VISA resource name=w2685, error in (no error)=w2684) -> ()  [unwired: 1 out]
                  }
                }
                n1595 = Concatenate Strings("enter pump1", w2621) -> (w2620:string)
                n1596 = local read "Normal \nRate (ul/hr)"() -> (w2606:dbl)
                n1597 = Concatenate Strings("set units 4 ", w2621) -> (w2617:string)
                n1598 = local read "Normal \nVolume (ul)"() -> (w2607:dbl)
                n1599 = Number To Decimal String(number=w2606) -> (decimal integer string=w2616:string)  [unwired: 1 in]
                n1600 = Concatenate Strings("set rate ", w2616, w2621) -> (w2614:string)
                n1601 = Number To Decimal String(number=w2607) -> (decimal integer string=w2612:string)  [unwired: 1 in]
                n1602 = Concatenate Strings("set volume ", w2612, w2621) -> (w2611:string)
              }
            }
          }
          event "Normal \nVolume (ul)": Value Change {
            n1603 = event-data() -> ()  [unwired: 1 in, 5 out]
            n1604 = call-poly "VISA Configure Serial Port"("VISA resource name"=w2706) -> ("VISA resource name out"=w2708:refnum<visa-resource-name>, "error out"=w2707:errorcluster)  [unwired: 13 in]
            n1605 = local read "Write Wait"() -> (w2691:i32)
            n1606 = Concatenate Strings("enter pump1", "\r") -> (w2710:string)
            n1607 = flat-sequence {
              tunnel: w2707 -> [w2720]
              tunnel: w2708 -> [w2722]
              tunnel: [w2721] -> w2700
              tunnel: [w2719] -> w2699
              tunnel: w2710 -> [w2718]
              tunnel: w2700 -> [w2725]
              tunnel: [w2725] -> w2698
              tunnel: w2699 -> [w2724]
              tunnel: [w2724] -> w2696
              tunnel: w2691 -> [w2723]
              tunnel: w2698 -> [w2729]
              tunnel: [w2730] -> w2697
              tunnel: w2696 -> [w2728]
              tunnel: [w2727] -> w2695
              tunnel: w2692 -> [w2726]
              tunnel: w2697 -> [w2733]
              tunnel: w2695 -> [w2732]
              tunnel: [w2733] -> w2717
              tunnel: [w2732] -> w2716
              tunnel: w2691 -> [w2731]
              tunnel: [w2738] -> w2715
              tunnel: [w2737] -> w2714
              tunnel: w2717 -> [w2736]
              tunnel: w2716 -> [w2735]
              tunnel: w2701 -> [w2734]
              tunnel: w2715 -> [w2741]
              tunnel: [w2741] -> w2713
              tunnel: w2714 -> [w2740]
              tunnel: [w2740] -> w2712
              tunnel: w2691 -> [w2739]
              tunnel: w2713 -> [w2745]
              tunnel: w2712 -> [w2744]
              frame #0 {
                n1608 = VISA Write(VISA resource name=w2722, write buffer=w2718, error in (no error)=w2720) -> (VISA resource name out=w2721:refnum<visa-resource-name>, error out=w2719:errorcluster)  [unwired: 1 out]
              }
              frame #1 {
                n1609 = Wait (ms)(milliseconds to wait=w2723) -> ()  [unwired: 1 out]
              }
              frame #2 {
                n1610 = VISA Write(VISA resource name=w2729, write buffer=w2726, error in (no error)=w2728) -> (VISA resource name out=w2730:refnum<visa-resource-name>, error out=w2727:errorcluster)  [unwired: 1 out]
              }
              frame #3 {
                n1611 = Wait (ms)(milliseconds to wait=w2731) -> ()  [unwired: 1 out]
              }
              frame #4 {
                n1612 = VISA Write(VISA resource name=w2736, write buffer=w2734, error in (no error)=w2735) -> (VISA resource name out=w2738:refnum<visa-resource-name>, error out=w2737:errorcluster)  [unwired: 1 out]
              }
              frame #5 {
                n1613 = Wait (ms)(milliseconds to wait=w2739) -> ()  [unwired: 1 out]
              }
              frame #6 {
                n1614 = Concatenate Strings("enter main ", "\r") -> (w2746:string)
                n1615 = VISA Write(VISA resource name=w2745, write buffer=w2746, error in (no error)=w2744) -> (VISA resource name out=w2743:refnum<visa-resource-name>, error out=w2742:errorcluster)  [unwired: 1 out]
                n1616 = VISA Close(VISA resource name=w2743, error in (no error)=w2742) -> ()  [unwired: 1 out]
              }
            }
            n1617 = Concatenate Strings("set units 4", "\r") -> (w2692:string)
            n1618 = Number To Decimal String(number="Normal \nVolume (ul)") -> (decimal integer string=w2703:string)  [unwired: 1 in]
            n1619 = Concatenate Strings("set volume", w2703, "\r") -> (w2701:string)
          }
          event "Normal \nRate (ul/hr)": Value Change {
            n1620 = event-data() -> ()  [unwired: 1 in, 5 out]
            n1621 = call-poly "VISA Configure Serial Port"("VISA resource name"=w2751) -> ("VISA resource name out"=w2759:refnum<visa-resource-name>, "error out"=w2758:errorcluster)  [unwired: 13 in]
            n1622 = local read "Write Wait"() -> (w2749:i32)
            n1623 = Concatenate Strings("enter pump1", "\r") -> (w2761:string)
            n1624 = flat-sequence {
              tunnel: w2758 -> [w2778]
              tunnel: w2759 -> [w2780]
              tunnel: [w2779] -> w2774
              tunnel: [w2777] -> w2773
              tunnel: w2761 -> [w2776]
              tunnel: w2774 -> [w2783]
              tunnel: [w2783] -> w2772
              tunnel: w2773 -> [w2782]
              tunnel: [w2782] -> w2771
              tunnel: w2749 -> [w2781]
              tunnel: w2772 -> [w2787]
              tunnel: [w2788] -> w2770
              tunnel: w2771 -> [w2786]
              tunnel: [w2785] -> w2769
              tunnel: w2752 -> [w2784]
              tunnel: w2770 -> [w2791]
              tunnel: w2769 -> [w2790]
              tunnel: [w2791] -> w2768
              tunnel: [w2790] -> w2767
              tunnel: w2749 -> [w2789]
              tunnel: [w2796] -> w2766
              tunnel: [w2795] -> w2765
              tunnel: w2768 -> [w2794]
              tunnel: w2767 -> [w2793]
              tunnel: w2755 -> [w2792]
              tunnel: w2766 -> [w2799]
              tunnel: [w2799] -> w2764
              tunnel: w2765 -> [w2798]
              tunnel: [w2798] -> w2763
              tunnel: w2749 -> [w2797]
              tunnel: w2764 -> [w2803]
              tunnel: w2763 -> [w2802]
              frame #0 {
                n1625 = VISA Write(VISA resource name=w2780, write buffer=w2776, error in (no error)=w2778) -> (VISA resource name out=w2779:refnum<visa-resource-name>, error out=w2777:errorcluster)  [unwired: 1 out]
              }
              frame #1 {
                n1626 = Wait (ms)(milliseconds to wait=w2781) -> ()  [unwired: 1 out]
              }
              frame #2 {
                n1627 = VISA Write(VISA resource name=w2787, write buffer=w2784, error in (no error)=w2786) -> (VISA resource name out=w2788:refnum<visa-resource-name>, error out=w2785:errorcluster)  [unwired: 1 out]
              }
              frame #3 {
                n1628 = Wait (ms)(milliseconds to wait=w2789) -> ()  [unwired: 1 out]
              }
              frame #4 {
                n1629 = VISA Write(VISA resource name=w2794, write buffer=w2792, error in (no error)=w2793) -> (VISA resource name out=w2796:refnum<visa-resource-name>, error out=w2795:errorcluster)  [unwired: 1 out]
              }
              frame #5 {
                n1630 = Wait (ms)(milliseconds to wait=w2797) -> ()  [unwired: 1 out]
              }
              frame #6 {
                n1631 = Concatenate Strings("enter main ", "\r") -> (w2804:string)
                n1632 = VISA Write(VISA resource name=w2803, write buffer=w2804, error in (no error)=w2802) -> (VISA resource name out=w2801:refnum<visa-resource-name>, error out=w2800:errorcluster)  [unwired: 1 out]
                n1633 = VISA Close(VISA resource name=w2801, error in (no error)=w2800) -> ()  [unwired: 1 out]
              }
            }
            n1634 = Concatenate Strings("set units 4", "\r") -> (w2752:string)
            n1635 = Number To Decimal String(number="Normal \nRate (ul/hr)") -> (decimal integer string=w2750:string)  [unwired: 1 in]
            n1636 = Concatenate Strings("set rate", w2750, "\r") -> (w2755:string)
          }
          event "Normal \nRate (ul/hr)  2": Value Change {
            n1637 = event-data() -> ()  [unwired: 1 in, 5 out]
            n1638 = call-poly "VISA Configure Serial Port"("VISA resource name"=w2809) -> ("VISA resource name out"=w2817:refnum<visa-resource-name>, "error out"=w2816:errorcluster)  [unwired: 13 in]
            n1639 = local read "Write Wait"() -> (w2807:i32)
            n1640 = Concatenate Strings("enter pump2", "\r") -> (w2819:string)
            n1641 = flat-sequence {
              tunnel: w2816 -> [w2836]
              tunnel: w2817 -> [w2838]
              tunnel: [w2837] -> w2832
              tunnel: [w2835] -> w2831
              tunnel: w2819 -> [w2834]
              tunnel: w2832 -> [w2841]
              tunnel: [w2841] -> w2830
              tunnel: w2831 -> [w2840]
              tunnel: [w2840] -> w2829
              tunnel: w2807 -> [w2839]
              tunnel: w2830 -> [w2845]
              tunnel: [w2846] -> w2828
              tunnel: w2829 -> [w2844]
              tunnel: [w2843] -> w2827
              tunnel: w2810 -> [w2842]
              tunnel: w2828 -> [w2849]
              tunnel: w2827 -> [w2848]
              tunnel: [w2849] -> w2826
              tunnel: [w2848] -> w2825
              tunnel: w2807 -> [w2847]
              tunnel: [w2854] -> w2824
              tunnel: [w2853] -> w2823
              tunnel: w2826 -> [w2852]
              tunnel: w2825 -> [w2851]
              tunnel: w2813 -> [w2850]
              tunnel: w2824 -> [w2857]
              tunnel: [w2857] -> w2822
              tunnel: w2823 -> [w2856]
              tunnel: [w2856] -> w2821
              tunnel: w2807 -> [w2855]
              tunnel: w2822 -> [w2861]
              tunnel: w2821 -> [w2860]
              frame #0 {
                n1642 = VISA Write(VISA resource name=w2838, write buffer=w2834, error in (no error)=w2836) -> (VISA resource name out=w2837:refnum<visa-resource-name>, error out=w2835:errorcluster)  [unwired: 1 out]
              }
              frame #1 {
                n1643 = Wait (ms)(milliseconds to wait=w2839) -> ()  [unwired: 1 out]
              }
              frame #2 {
                n1644 = VISA Write(VISA resource name=w2845, write buffer=w2842, error in (no error)=w2844) -> (VISA resource name out=w2846:refnum<visa-resource-name>, error out=w2843:errorcluster)  [unwired: 1 out]
              }
              frame #3 {
                n1645 = Wait (ms)(milliseconds to wait=w2847) -> ()  [unwired: 1 out]
              }
              frame #4 {
                n1646 = VISA Write(VISA resource name=w2852, write buffer=w2850, error in (no error)=w2851) -> (VISA resource name out=w2854:refnum<visa-resource-name>, error out=w2853:errorcluster)  [unwired: 1 out]
              }
              frame #5 {
                n1647 = Wait (ms)(milliseconds to wait=w2855) -> ()  [unwired: 1 out]
              }
              frame #6 {
                n1648 = Concatenate Strings("enter main ", "\r") -> (w2862:string)
                n1649 = VISA Write(VISA resource name=w2861, write buffer=w2862, error in (no error)=w2860) -> (VISA resource name out=w2859:refnum<visa-resource-name>, error out=w2858:errorcluster)  [unwired: 1 out]
                n1650 = VISA Close(VISA resource name=w2859, error in (no error)=w2858) -> ()  [unwired: 1 out]
              }
            }
            n1651 = Concatenate Strings("set units 4", "\r") -> (w2810:string)
            n1652 = Number To Decimal String(number="Normal \nRate (ul/hr)  2") -> (decimal integer string=w2808:string)  [unwired: 1 in]
            n1653 = Concatenate Strings("set rate", w2808, "\r") -> (w2813:string)
          }
          event "Normal \nVolume (ul) 2": Value Change {
            n1654 = event-data() -> ()  [unwired: 1 in, 5 out]
            n1655 = call-poly "VISA Configure Serial Port"("VISA resource name"=w2868) -> ("VISA resource name out"=w2872:refnum<visa-resource-name>, "error out"=w2873:errorcluster)  [unwired: 13 in]
            n1656 = local read "Write Wait"() -> (w2865:i32)
            n1657 = Concatenate Strings("enter pump2", "\r") -> (w2870:string)
            n1658 = flat-sequence {
              tunnel: w2873 -> [w2894]
              tunnel: w2872 -> [w2896]
              tunnel: [w2895] -> w2891
              tunnel: [w2893] -> w2890
              tunnel: w2870 -> [w2892]
              tunnel: w2891 -> [w2899]
              tunnel: [w2899] -> w2889
              tunnel: w2890 -> [w2898]
              tunnel: [w2898] -> w2888
              tunnel: w2865 -> [w2897]
              tunnel: w2889 -> [w2903]
              tunnel: [w2904] -> w2887
              tunnel: w2888 -> [w2902]
              tunnel: [w2901] -> w2886
              tunnel: w2879 -> [w2900]
              tunnel: w2887 -> [w2907]
              tunnel: w2886 -> [w2906]
              tunnel: [w2907] -> w2885
              tunnel: [w2906] -> w2884
              tunnel: w2865 -> [w2905]
              tunnel: [w2912] -> w2883
              tunnel: [w2911] -> w2882
              tunnel: w2885 -> [w2910]
              tunnel: w2884 -> [w2909]
              tunnel: w2876 -> [w2908]
              tunnel: w2883 -> [w2915]
              tunnel: [w2915] -> w2881
              tunnel: w2882 -> [w2914]
              tunnel: [w2914] -> w2880
              tunnel: w2865 -> [w2913]
              tunnel: w2881 -> [w2919]
              tunnel: w2880 -> [w2918]
              frame #0 {
                n1659 = VISA Write(VISA resource name=w2896, write buffer=w2892, error in (no error)=w2894) -> (VISA resource name out=w2895:refnum<visa-resource-name>, error out=w2893:errorcluster)  [unwired: 1 out]
              }
              frame #1 {
                n1660 = Wait (ms)(milliseconds to wait=w2897) -> ()  [unwired: 1 out]
              }
              frame #2 {
                n1661 = VISA Write(VISA resource name=w2903, write buffer=w2900, error in (no error)=w2902) -> (VISA resource name out=w2904:refnum<visa-resource-name>, error out=w2901:errorcluster)  [unwired: 1 out]
              }
              frame #3 {
                n1662 = Wait (ms)(milliseconds to wait=w2905) -> ()  [unwired: 1 out]
              }
              frame #4 {
                n1663 = VISA Write(VISA resource name=w2910, write buffer=w2908, error in (no error)=w2909) -> (VISA resource name out=w2912:refnum<visa-resource-name>, error out=w2911:errorcluster)  [unwired: 1 out]
              }
              frame #5 {
                n1664 = Wait (ms)(milliseconds to wait=w2913) -> ()  [unwired: 1 out]
              }
              frame #6 {
                n1665 = Concatenate Strings("enter main ", "\r") -> (w2920:string)
                n1666 = VISA Write(VISA resource name=w2919, write buffer=w2920, error in (no error)=w2918) -> (VISA resource name out=w2917:refnum<visa-resource-name>, error out=w2916:errorcluster)  [unwired: 1 out]
                n1667 = VISA Close(VISA resource name=w2917, error in (no error)=w2916) -> ()  [unwired: 1 out]
              }
            }
            n1668 = Concatenate Strings("set units 4", "\r") -> (w2879:string)
            n1669 = Number To Decimal String(number="Normal \nVolume (ul) 2") -> (decimal integer string=w2866:string)  [unwired: 1 in]
            n1670 = Concatenate Strings("set volume", w2866, "\r") -> (w2876:string)
          }
        }
        n1671 = node-c288() -> ()  [unwired: 1 in, 1 out]
      }
      n1672 = node-c288(w2252) -> ()  [unwired: 1 out]
    }
    frame Enabled {
      n1673 = node-c288(2 ("Processor")) -> (w2932:T13)  [unwired: 3 in]
      n1674 = timed-loop "Pump Control" {
        timing: w2932 -> [_]
        timing-out: [_] -> w2931
        tunnel: refnum<visa-resource-name> "COM4" ("VISA resource name") -> [w2934]
        stop <- w2933 stop-if-true
        n1675 = node-c288() -> ()  [unwired: 1 in, 1 out]
        n1676 = event shown="[2] \"Inject Sample\": Value Change" {
          selector: _ -> [_ _ _ _ _]
          dyn-events: _ -> [_ _ _ _ _]
          timeout: _ -> [_ _ _ _ _]
          tunnel: w2934 -> [w2940 _ w3014 w3041 w3046]
          tunnel: [_ w3012 _ _ _] -> w2933
          event "Flush Sample": Value Change {
            n1677 = event-data() -> ()  [unwired: 1 in, 5 out]
            n1678 = local read "Write Wait"() -> (w2954:i32)
            n1679 = flat-sequence {
              tunnel: [w2978] -> w2974
              tunnel: [w2977] -> w2973
              tunnel: "CLD" -> [w2976]
              tunnel: w2940 -> [w2975]
              tunnel: w2974 -> [w2981]
              tunnel: [w2981] -> w2972
              tunnel: w2973 -> [w2980]
              tunnel: [w2980] -> w2971
              tunnel: w2954 -> [w2979]
              tunnel: [w2986] -> w2970
              tunnel: [w2983] -> w2969
              tunnel: w2972 -> [w2985]
              tunnel: w2971 -> [w2984]
              tunnel: "MODVOL" -> [w2982]
              tunnel: w2970 -> [w2989]
              tunnel: [w2989] -> w2968
              tunnel: [w2988] -> w2967
              tunnel: w2969 -> [w2988]
              tunnel: w2954 -> [w2987]
              tunnel: w2968 -> [w2994]
              tunnel: [w2993] -> w2966
              tunnel: w2956 -> [w2992]
              tunnel: w2967 -> [w2991]
              tunnel: [w2990] -> w2965
              tunnel: w2966 -> [w2997]
              tunnel: [w2997] -> w2964
              tunnel: [w2996] -> w2963
              tunnel: w2965 -> [w2996]
              tunnel: w2954 -> [w2995]
              tunnel: w2964 -> [w3002]
              tunnel: [w3001] -> w2962
              tunnel: w2958 -> [w3000]
              tunnel: w2963 -> [w2999]
              tunnel: [w2998] -> w2961
              tunnel: [w3005] -> w2959
              tunnel: w2962 -> [w3005]
              tunnel: [w3004] -> w2960
              tunnel: w2961 -> [w3004]
              tunnel: w2954 -> [w3003]
              tunnel: w2960 -> [w3010]
              tunnel: w2959 -> [w3011]
              tunnel: [w3009] -> w2949
              tunnel: "RUN " -> [w3008]
              frame #0 {
                n1680 = call "Write to pump 2.vi"("String to write"=w2976, "VISA resource name"=w2975) -> ("error out"=w2977:errorcluster, "VISA resource name out"=w2978:refnum<visa-resource-name>)  [unwired: 8 in]
              }
              frame #1 {
                n1681 = Wait (ms)(milliseconds to wait=w2979) -> ()  [unwired: 1 out]
              }
              frame #2 {
                n1682 = call "Write to pump 2.vi"("error in (no error)"=w2984, "String to write"=w2982, "VISA resource name"=w2985) -> ("error out"=w2983:errorcluster, "VISA resource name out"=w2986:refnum<visa-resource-name>)  [unwired: 7 in]
              }
              frame #3 {
                n1683 = Wait (ms)(milliseconds to wait=w2987) -> ()  [unwired: 1 out]
              }
              frame #4 {
                n1684 = call "Write to pump 2.vi"("error in (no error)"=w2991, "String to write"=w2992, "VISA resource name"=w2994) -> ("error out"=w2990:errorcluster, "VISA resource name out"=w2993:refnum<visa-resource-name>)  [unwired: 7 in]
              }
              frame #5 {
                n1685 = Wait (ms)(milliseconds to wait=w2995) -> ()  [unwired: 1 out]
              }
              frame #6 {
                n1686 = call "Write to pump 2.vi"("error in (no error)"=w2999, "String to write"=w3000, "VISA resource name"=w3002) -> ("error out"=w2998:errorcluster, "VISA resource name out"=w3001:refnum<visa-resource-name>)  [unwired: 7 in]
              }
              frame #7 {
                n1687 = Wait (ms)(milliseconds to wait=w3003) -> ()  [unwired: 1 out]
              }
              frame #8 {
                w3007 = TRUE ("Inject Pump 3")
                n1688 = Tick Count (ms)() -> (millisecond timer value=→"Flush Sample Start Time":u32)
                n1689 = call "Write to pump 2.vi"("error in (no error)"=w3010, "String to write"=w3008, "VISA resource name"=w3011) -> ("error out"=w3009:errorcluster)  [unwired: 7 in, 1 out]
                n1690 = local write "Inject Sample"(w3007) -> ()
                "Flushing Sample" <- w3007
              }
            }
            n1691 = Number To Fractional String(number="Flush \nRate (ul/min)  3") -> (F-format string=w2942:string)  [unwired: 3 in]
            n1692 = String Subset(string=w2942, length (rest)=6 ("length (rest)")) -> (substring=w2941:string)  [unwired: 1 in]
            n1693 = Concatenate Strings("RAT", w2941, "UM") -> (w2956:string)
            n1694 = Divide(x="Flush\nVolume (ul)  3", y=1000.0) -> (x/y=w2947:dbl)
            n1695 = Number To Fractional String(number=w2947) -> (F-format string=w2946:string)  [unwired: 3 in]
            n1696 = Divide(x="Flush\nVolume (ul)  3", y="Flush \nRate (ul/min)  3") -> (x/y=w2937:dbl)
            n1697 = Multiply(x=w2937, y=60.0) -> (x*y=→"Sample flush time (s)":dbl)
            n1698 = String Subset(string=w2946, length (rest)=6 ("length (rest)")) -> (substring=w2945:string)  [unwired: 1 in]
            n1699 = Concatenate Strings("TGT", w2945) -> (w2958:string)
            "error out" <- w2949
          }
          event "Stop": Value Change {
            n1700 = event-data() -> ()  [unwired: 1 in, 5 out]
            n1701 = local read "Stop"() -> (w3012:bool)
          }
          event "Inject Sample": Value Change {
            n1702 = event-data() -> ()  [unwired: 1 in, 5 out]
            n1703 = case shown="True" "Inject Sample" {
              tunnel: w3014 -> [w3016 w3017]
              frame False {
                n1704 = call "Write to pump 2.vi"("String to write"="STP", "VISA resource name"=w3016) -> ()  [unwired: 8 in, 2 out]
              }
              frame True {
                n1705 = local read "Normal \nRate (ul/hr)  3"() -> (w3018:dbl)
                n1706 = Number To Fractional String(number=w3018) -> (F-format string=w3021:string)  [unwired: 3 in]
                n1707 = String Subset(string=w3021, length (rest)=6 ("length (rest)")) -> (substring=w3019:string)  [unwired: 1 in]
                n1708 = flat-sequence {
                  tunnel: "RUN " -> [w3033]
                  tunnel: [w3035] -> _
                  tunnel: [w3034] -> _
                  tunnel: w3017 -> [w3032]
                  frame #0 {
                    n1709 = call "Write to pump 2.vi"("String to write"=w3033, "VISA resource name"=w3032) -> ("error out"=w3034:errorcluster, "VISA resource name out"=w3035:refnum<visa-resource-name>)  [unwired: 8 in]
                  }
                }
                n1710 = Concatenate Strings("RAT", w3019, "UH" ("string")) -> ()  [unwired: 1 out]
                n1711 = local read "Normal \nVolume (ul) 3"() -> (w3027:dbl)
                n1712 = Divide(x=w3027, y=1000.0) -> (x/y=w3022:dbl)
                n1713 = Number To Fractional String(number=w3022) -> (F-format string=w3025:string)  [unwired: 3 in]
                n1714 = String Subset(string=w3025, length (rest)=6 ("length (rest)")) -> (substring=w3023:string)  [unwired: 1 in]
                n1715 = Concatenate Strings("TGT", w3023) -> ()  [unwired: 1 out]
              }
            }
          }
          event "Normal \nRate (ul/hr)  3": Value Change {
            n1716 = event-data() -> ()  [unwired: 1 in, 5 out]
            n1717 = Number To Fractional String(number="Normal \nRate (ul/hr)  3") -> (F-format string=w3039:string)  [unwired: 3 in]
            n1718 = String Subset(string=w3039, length (rest)=6 ("length (rest)")) -> (substring=w3037:string)  [unwired: 1 in]
            n1719 = Concatenate Strings("RAT", w3037, "UH") -> (w3040:string)
            n1720 = call "Write to pump 2.vi"("String to write"=w3040, "VISA resource name"=w3041) -> ()  [unwired: 8 in, 2 out]
          }
          event "Clear Volume": Value Change {
            n1721 = event-data() -> ()  [unwired: 1 in, 5 out]
            n1722 = Divide(x="Normal \nVolume (ul) 3", y=1000.0) -> (x/y=w3059:dbl)
            n1723 = Number To Fractional String(number=w3059) -> (F-format string=w3062:string)  [unwired: 3 in]
            n1724 = String Subset(string=w3062, length (rest)=6 ("length (rest)")) -> (substring=w3060:string)  [unwired: 1 in]
            n1725 = flat-sequence {
              tunnel: [w3069] -> w3057
              tunnel: [w3068] -> w3056
              tunnel: w3046 -> [w3067]
              tunnel: w3045 -> [w3066]
              tunnel: [w3071] -> w3054
              tunnel: [w3070] -> w3055
              tunnel: w3051 -> [w3072]
              tunnel: w3057 -> [w3071]
              tunnel: w3056 -> [w3070]
              tunnel: w3055 -> [w3076]
              tunnel: w3054 -> [w3077]
              tunnel: [w3075] -> _
              tunnel: [w3074] -> _
              tunnel: w3044 -> [w3073]
              frame #0 {
                n1726 = call "Write to pump 2.vi"("String to write"=w3066, "VISA resource name"=w3067) -> ("error out"=w3068:errorcluster, "VISA resource name out"=w3069:refnum<visa-resource-name>)  [unwired: 8 in]
              }
              frame #1 {
                n1727 = Wait (ms)(milliseconds to wait=w3072) -> ()  [unwired: 1 out]
              }
              frame #2 {
                n1728 = call "Write to pump 2.vi"("error in (no error)"=w3076, "String to write"=w3073, "VISA resource name"=w3077) -> ("error out"=w3074:errorcluster, "VISA resource name out"=w3075:refnum<visa-resource-name>)  [unwired: 7 in]
              }
            }
            n1729 = local read "Write Wait"() -> (w3051:i32)
            n1730 = Concatenate Strings("TGT", w3060) -> (w3045:string)
            n1731 = local read "Normal \nRate (ul/hr)  3"() -> (w3047:dbl)
            n1732 = local write "Clear Volume"(FALSE ("Clear Volume")) -> ()
            n1733 = Number To Fractional String(number=w3047) -> (F-format string=w3050:string)  [unwired: 3 in]
            n1734 = String Subset(string=w3050, length (rest)=6 ("length (rest)")) -> (substring=w3048:string)  [unwired: 1 in]
            n1735 = Concatenate Strings("RAT", w3048, "UH" ("string")) -> (w3044:string)
          }
        }
        n1736 = node-c288() -> ()  [unwired: 1 in, 1 out]
      }
      n1737 = node-c288(w2931) -> ()  [unwired: 1 out]
    }
  }
  n1738 = node-c288() -> (w90:T13)  [unwired: 4 in]
  n1739 = timed-loop {
    timing: w90 -> [_]
    timing-out: [_] -> w89
    stop <- w3084 stop-if-true
    n1740 = node-c288() -> ()  [unwired: 1 in, 1 out]
    n1741 = event shown="[1] \"Stop\": Value Change" {
      selector: _ -> [_ _]
      dyn-events: _ -> [_ _]
      timeout: _ -> [_ _]
      tunnel: [_ w3085] -> w3084
      event Timeout {
        n1742 = event-data() -> ()  [unwired: 1 in, 2 out]
      }
      event "Stop": Value Change {
        n1743 = event-data() -> ()  [unwired: 1 in, 4 out]
        n1744 = flat-sequence {
          tunnel: ["Stop"] -> w3085
          frame #0 {
            w3086 = FALSE ("Force Feedback")
            n1745 = local write "Force Feedback 1"(w3086) -> ()
            n1746 = local write "Force Feedback 2"(w3086) -> ()
            n1747 = property on="Cancel dwell" class="Bool (strict)"("Val(Sgnl)"=TRUE ("Value (Signaling)")) -> ()  [unwired: 2 in, 2 out]
          }
          frame #1 {
            w3088 = FALSE
            n1748 = local write "Raster scanning..."(w3088) -> ()
            n1749 = local write "Cancel dwell"(w3088) -> ()
            n1750 = local write "Stage moving"(w3088) -> ()
            n1751 = local write "Saving Move"(w3088) -> ()
          }
        }
      }
    }
    n1752 = node-c288() -> ()  [unwired: 1 in, 1 out]
  }
  n1753 = case shown="True" w80 {
    tunnel: w85 -> [_ w3094]
    tunnel: w84 -> [_ w3093]
    tunnel: w83 -> [_ w3092]
    frame False {
    }
    frame True {
      w3096 = T24 3 items=["no dialog", "OK message", "continue or stop message", "OK message + warnings", "continue/stop + warnings"] ("type of dialog (OK msg:1)")
      w3095 = T24 3 items=["no dialog", "OK message", "continue or stop message", "OK message + warnings", "continue/stop + warnings"] ("type of dialog (OK msg:1)")
      n1754 = call <vilib>:"DAQmx Clear Task.vi"("task in"=w3094, "error in"=w3092) -> ("error out"=w3097:errorcluster)  [unwired: 13 in]
      n1755 = call <vilib>:"DAQmx Clear Task.vi"("task in"=w3093) -> ("error out"=w3098:errorcluster)  [unwired: 14 in]
      n1756 = call <vilib>:"Simple Error Handler.vi"("type of dialog (OK msg:1)"=w3096, "error in (no error)"=w3097) -> ()  [unwired: 3 in, 5 out]
      n1757 = call <vilib>:"Simple Error Handler.vi"("type of dialog (OK msg:1)"=w3095, "error in (no error)"=w3098) -> ()  [unwired: 3 in, 5 out]
    }
  }
  n1758 = case shown="\"Raster scan\"" "?" {
    frame "Force Feedback", Default {
    }
    frame "Raster scan" {
    }
  }
  n1759 = node-c288(w89) -> ()  [unwired: 1 out]
  n1760 = node-c288(w92) -> ()  [unwired: 1 out]
  n1761 = local write "Pause Mouse/Mirror Connection"(FALSE ("Pause Mouse/Mirror Connection")) -> ()
  n1762 = local write "Stop"(FALSE ("Stop all")) -> ()
  "CoordinatesMousePressed" <- T5 {"Horizontal"=0, "Vertical"=0} ("Coords when pressed")
  "Deflection" <- T5 {"Horizontal"=0, "Vertical"=0} ("Coords when pressed")
